vi "CRYSoundCard Editor.vi"() -> ()   [LabVIEW 2013]
uses:
  Typedef Control/CRYHardware.ctl
  Typedef Control/CRYHardware Channel Info.ctl
  <vilib>/Utility/miscctls.llb/LVBoundsTypeDef.ctl
  Typedef Control/CRYCalibration Channel ID Cluster.ctl
  CRYProject/CRYProject Editor Global.vi
  CRYMainGlobal.vi
  CRYWindow/SubVI/CRYMain Sub Window Global.vi
  Calibration/SubVI/CRYCal Global.vi
panel:
  in  "AI_HW_Changed":bool caption="啊瓷"
  in  "AO_HW_Changed":bool caption="啊瓷"
  in  "Mode":string
  out "O_Name":string[][](array[string])
  out "I_Name":string[][](array[string])
  in  "DC_Table":string[][](table)
  in  "DC_Enable":bool caption="使能"
  out "EndFlag":bool
  in  "AddStep":bool caption="Save As"
  in  "I_Cal Channel ID":T1
  in  "O_Cal Channel ID":T1
  in  "Curve Change":enum16{"Curves", "Values", "Results", "WFM"}[](array[ring])
  in  "stop":bool
  in  "Load Test":bool
  in  "Board Tab":enum32{"Page 1", "Page 2"}(tab)
  in  "Refresh":bool caption="Open_Table"
  in  "Main Tab":enum32{"Audio", "", "Help 3", "Help"}(tab)
  in  "Audio I/O Tab":enum32{"Output", "Input"}(tab)
  in  "AO_Launch":bool caption="Open_Table"
  in  "AO_Select Channel1":u16(ring) caption="选择通道" items=["左边", "右边"]
  in  "AO_Audio Driver":enum32{"Radio Selection 1", "Radio Selection 2"}(radio) caption="声卡驱动"
  out "AO_%FSD":dbl=100.0 caption="%FSD"
  in  "AO_Rename":bool caption="Open_Table"
  in  "AO_Delete":bool caption="Open_Table"
  in  "AO_Vp":dbl=0.01 caption="峰值电压（Vp）" min=0.01 format="%#.3p"
  in  "AO_Bit Depth":u16(ring) caption="比特数" items=["8 bit"=8, "16 bit"=16, "24 bit"=24, "32 bit"=32]
  in  "AO_Alias freq":u32 caption="分析频率上限" max=22050 format="%#_6f"
  in  "AO_Sampling Rate":u32(ring) caption="采样率" items=["8000 Hz"=8000, "11025 Hz"=11025, "16000 Hz"=16000, "22050 Hz"=22050, "32000 Hz"=32000, "44100 Hz"=44100, "48000 Hz"=48000, "88200 Hz"=88200, "96000 Hz"=96000, "176400 Hz"=176400, "192000 Hz"=192000, "200000 Hz"=200000, "User"=0]
  in  "AO_Select SMode":enum32{"Analog", "Digital"}(radio) caption="AO_Select Channel2"
  in  "AO_Sampling User":u32=1 caption="(Hz)" min=8000 max=200000
  in  "AO_Device Name":u16(ring) caption="设备名称" items=["扬声器 (High Definition Audio 设备)", "数字音频(S/PDIF) (High Definition A", "扬声器 (QUARTET Audio Driver)", "SPDIF 接口 (QUARTET Audio Driver)"]
  out "Advance Out Rect":bool
  in  "AO_Add":bool caption="Open_Table"
  in  "AO_SoundCard Channel":u16(ring) caption="声卡通道" items=["Output 1", "Output 2", "Output 3", "Output 4"]
  in  "AI_Audio Driver":enum32{"Radio Selection 1", "Radio Selection 2"}(radio) caption="声卡驱动"
  out "Advance In Rect":bool
  in  "AI_Vp":dbl=0.01 caption="峰值电压（Vp）" min=0.01 format="%#.3p"
  in  "AI_Bit Depth":u16(ring) caption="比特数" items=["8 bit"=8, "16 bit"=16, "24 bit"=24, "32 bit"=32]
  in  "AI_Alias freq":u32 caption="分析频率上限" max=22050 format="%#_6f"
  in  "AI_Sampling Rate":u32(ring) caption="采样率" items=["8000 Hz"=8000, "11025 Hz"=11025, "16000 Hz"=16000, "22050 Hz"=22050, "32000 Hz"=32000, "44100 Hz"=44100, "48000 Hz"=48000, "88200 Hz"=88200, "96000 Hz"=96000, "176400 Hz"=176400, "192000 Hz"=192000, "200000 Hz"=200000, "User"=0]
  in  "AI_Select SMode":enum32{"Analog", "Digital"}(radio) caption="AI_Select Channel2"
  in  "AI_Latency":u32 caption="延迟"
  in  "AI_Device Name":u16(ring) caption="设备名称" items=["麦克风 (QUARTET Audio Driver)", "线路 (QUARTET Audio Driver)"]
  in  "AI_Sampling User":u32 caption="(Hz)" min=8000 max=200000
  in  "AI_SoundCard Channel":u16(ring) caption="声卡通道" items=["Input 1", "Input 2", "Input 3", "Input 4"]
  in  "AI_Add":bool caption="Open_Table"
  in  "AI_Delete":bool caption="Open_Table"
  in  "AI_Rename":bool caption="Open_Table"
  out "AI_%FSD":dbl=100.0 caption="%FSD"
  in  "AI_Select Channel1":u16(ring) caption="选择通道" items=["左边", "右边"]
  in  "AI_Launch":bool caption="Open_Table"
  in  "Advanced View":bool
  in  "Calibration Seq":u16(ring) caption="校准序列" items=["CRY6181 Calibration"]
  in  "Calibrartion":bool caption="Open_Table"
  in  "D_Select Channel":enum32{"Radio Selection 1", "Radio Selection 2"}(radio) caption="选择通道"
  in  "D_Port No.":u32(ring) caption="端口编号"
  in  "D_PortWidth":u32 caption="端口宽度"
  in  "D_No.of Ports":u8=1 caption="端口数量" min=1
  in  "D_Device ID":u32 caption="设备编号" format="%_1f"
  in  "D_Enable":bool caption="启用"
  in  "I_Data bits":u8 caption="数据位" min=5 max=8
  in  "I_Baud":u16 caption="波特率"
  in  "I_COM Port":u8=1 caption="串行通讯端口" min=1
  in  "I_Flow control":u8(ring) caption="流控制" items=["Xon/Xoff", "Hardware", "None"]
  in  "I_Stop bits":u8(ring) caption="停止位" items=["1", "1.5", "2"]
  in  "I_Parity":u8(ring) caption="奇偶性" items=["None", "Odd", "Even", "Mark", "Space"]
  in  "I_No":u32(ring) caption="接口号"
  in  "I_Type":u8(ring) caption="类型" items=["IEEE-488", "RS-232", "Footswitch", "Buzzer"]
  in  "I_How many":u32 caption="接口数量"
  in  "I_Dev ID IEEE":u8 caption="设备标识 IEEE"
  in  "Help":string
  in  "Open_Table":bool
  in  "SaveSoundCard":bool caption="Apply"
  in  "Cancel":bool caption="Apply"
  in  "Load...":bool caption="Apply"
  in  "Revert":bool caption="Apply"
  out "Channel Info":T2={"ID"=0, "Name"="", "Digital"=FALSE, "Input"=FALSE, "Device Name"="", "Hardware Ch ID"=0, "Vmax (V)"=0.0, "Latency (samples)"=0.0, "Sampling Rate (Hz)"=0, "Bit Depth"=0, "Anti-aliasing Factor (%fs)"=0.475, "DAQmx Channel"="", "term config"=-1, "Coupling"=10050, "IEPE en"=FALSE, "ASIOChannel Name"="", "Audio Driver"=0, "ASIOChannel Index"=0} {"Coupling" items=["Default"=-1, "RSE"=10083, "NRSE"=10078, "Differential"=10106, "Pseudodifferential"=12529]; "term config" items=["Default"=-1, "RSE"=10083, "NRSE"=10078, "Differential"=10106, "Pseudodifferential"=12529]; "Anti-aliasing Factor (%fs)" format="%.2f"}
  out "O_Channel Info":T2[](array[typedef]) {"Coupling" items=["Default"=-1, "RSE"=10083, "NRSE"=10078, "Differential"=10106, "Pseudodifferential"=12529]; "term config" items=["Default"=-1, "RSE"=10083, "NRSE"=10078, "Differential"=10106, "Pseudodifferential"=12529]; "Anti-aliasing Factor (%fs)" format="%.2f"}
  in  "I_Channel Info":T2[](array[typedef]) {"Coupling" items=["Default"=-1, "RSE"=10083, "NRSE"=10078, "Differential"=10106, "Pseudodifferential"=12529]; "term config" items=["Default"=-1, "RSE"=10083, "NRSE"=10078, "Differential"=10106, "Pseudodifferential"=12529]; "Anti-aliasing Factor (%fs)" format="%.2f"}
  out "I_Device Info":T3(array[cluster])
  out "O_Device Info":T3(array[cluster])
  out "Proper VI No":i32
  out "VIMiniumBound":T4
  in  "SoundCard":T5={"Name"="", "Analog I/O"=0, "Digital I/O"=0, "Channels"=2, "Dig Dev ID"=1, "N ports"=3, "Interface"=0, "Dig I/O Ports"=[{"port #"=1, "width"=8, "direction"=0}, {"port #"=2, "width"=8, "direction"=0}, {"port #"=3, "width"=8, "direction"=0}], "Interf settings"=[], "N interfs"=3, "udev SNs"=[], "udev enable"=FALSE, "Channel Array"=[], "Cal sequence"="", "SelectedIn"=0, "SelectedOut"=0, "SelectedTab"=0, "State"=FALSE, "Help"="", "Advanced"=FALSE, "In Audio Driver"=0, "Out Audio Driver"=0} caption="Hardware" {"Channel Array"."Coupling" items=["Default"=-1, "RSE"=10083, "NRSE"=10078, "Differential"=10106, "Pseudodifferential"=12529]; "Channel Array"."term config" items=["Default"=-1, "RSE"=10083, "NRSE"=10078, "Differential"=10106, "Pseudodifferential"=12529]; "Channel Array"."Anti-aliasing Factor (%fs)" format="%.2f"}
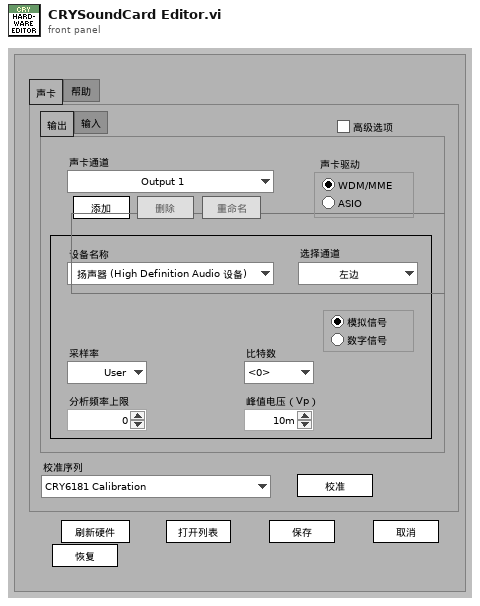
[diagram p1: front panel]
types:
  T1 = typedef "CRYCalibration Channel ID Cluster.ctl" = cluster{"Edit Name":string, "Edit ID":i8}[]
  T2 = typedef "CRYHardware Channel Info.ctl" = cluster{"ID":i32, "Name":string, "Digital":bool, "Input":bool, "Device Name":string, "Hardware Ch ID":u8, "Vmax (V)":dbl, "Latency (samples)":dbl, "Sampling Rate (Hz)":u32, "Bit Depth":u32, "Anti-aliasing Factor (%fs)":sgl, "DAQmx Channel":tag, "term config":i32, "Coupling":i32, "IEPE en":bool, "ASIOChannel Name":string, "Audio Driver":u16, "ASIOChannel Index":u8}
  T3 = cluster{"Name":string, "MinFreq":dbl, "MaxFreq":dbl, "Channel":i32[], "Depths":i32[], "Channel Names":string[], "SampleRates Array":dbl[], "Driver Type":string}[]
  T4 = typedef "LVBoundsTypeDef.ctl" = cluster{"Width":u32, "Height":u32}
  T5 = typedef "CRYHardware.ctl" = cluster{"Name":string, "Analog I/O":u16, "Digital I/O":u16, "Channels":u8, "Dig Dev ID":u8, "N ports":u8, "Interface":u32, "Dig I/O Ports":cluster{"port #":i16, "width":i16, "direction":i32}[], "Interf settings":cluster{"Type":u16, "COM Port":u8, "Baud rate":u32, "Data bits":u32, "Parity":u16, "Stop bits":u16, "Flow control":u16, "Dev ID IEEE":u8}[], "N interfs":i32, "udev SNs":i16[], "udev enable":bool, "Channel Array":T2[], "Cal sequence":string, "SelectedIn":u16, "SelectedOut":u16, "SelectedTab":u16, "State":bool, "Help":string, "Advanced":bool, "In Audio Driver":u16, "Out Audio Driver":u16}
  T6 = typedef "CRYStep.ctl" = cluster{"No.VI":i32, "Category":string, "StepName":string, "Seq setup flattened":string, "Comment":string, "Steps config.":bool[], "Jump config":i32[], "Start":dbl, "Increment":dbl, "Name":string, "Unit":string, "Y data":u16, "Y prefix":string, "Y dB ref":dbl, "Y unit":string, "Repeat State Array":cluster{"Start":dbl, "Increment":dbl, "Count":i32, "Num":i32}[]}
  T7 = enum8{"Enabled", "Disabled", "Disabled and Grayed Out"}
  T8 = enum16{"OK", "Yes", "YesNo", "YesNoCancel", "ReplaceAppend"}
  T9 = cluster{"port #":i16, "width":i16, "direction":i32}[]
  T10 = cluster{"port #":i16, "width":i16, "direction":i32}
  T11 = cluster{"Type":u16, "COM Port":u8, "Baud rate":u32, "Data bits":u32, "Parity":u16, "Stop bits":u16, "Flow control":u16, "Dev ID IEEE":u8}
  T12 = cluster{"Name":string, "MinFreq":dbl, "MaxFreq":dbl, "Channel":i32[], "Depths":i32[], "Channel Names":string[], "SampleRates Array":dbl[], "Driver Type":string}
  T13 = typedef "LVStringsAndValuesArrayTypeDef_U32.ctl" = cluster{"String":string, "Value":u32}[]
  T14 = cluster{"Type":u16, "COM Port":u8, "Baud rate":u32, "Data bits":u32, "Parity":u16, "Stop bits":u16, "Flow control":u16, "Dev ID IEEE":u8}[]
  T15 = cluster{bool, "AO_Add":bool, "AO_Delete":bool, "AO_Rename":bool, "AI_Add":bool, "AI_Delete":bool, "AI_Rename":bool, "Open_Table":bool, "Calibrartion":bool, "SaveSoundCard":bool, "Cancel":bool}
  T16 = typedef "CRYData Cluster Array.ctl" = T17[]
  T17 = typedef "CRYData Cluster.ctl" = cluster{"Name":string, "Curve":cluster{"x":dbl, "y":dbl, "z":dbl}[], "X data":u16, "Y data":u16, "Z data":u16, "X axis":u16, "Y axis":u16, "Z axis":u16, "X unit":string, "Y unit":string, "Z unit":string, "X dB ref":dbl, "Y dB ref":dbl, "Z dB ref":dbl, "single val":bool, "protected":bool, "display X":bool, "display Y":bool, "display Z":bool, "Test Info":string, "Step No.":i32, "Plot Settings":cluster{"Color":u32, "Interpolation":u8, "Point Style":u8, "Line Style":u8, "Point Color":u32, "Line Width":u8, "Bar Plot Style":u8, "Fill To":i16}, "AutoProtect":bool}
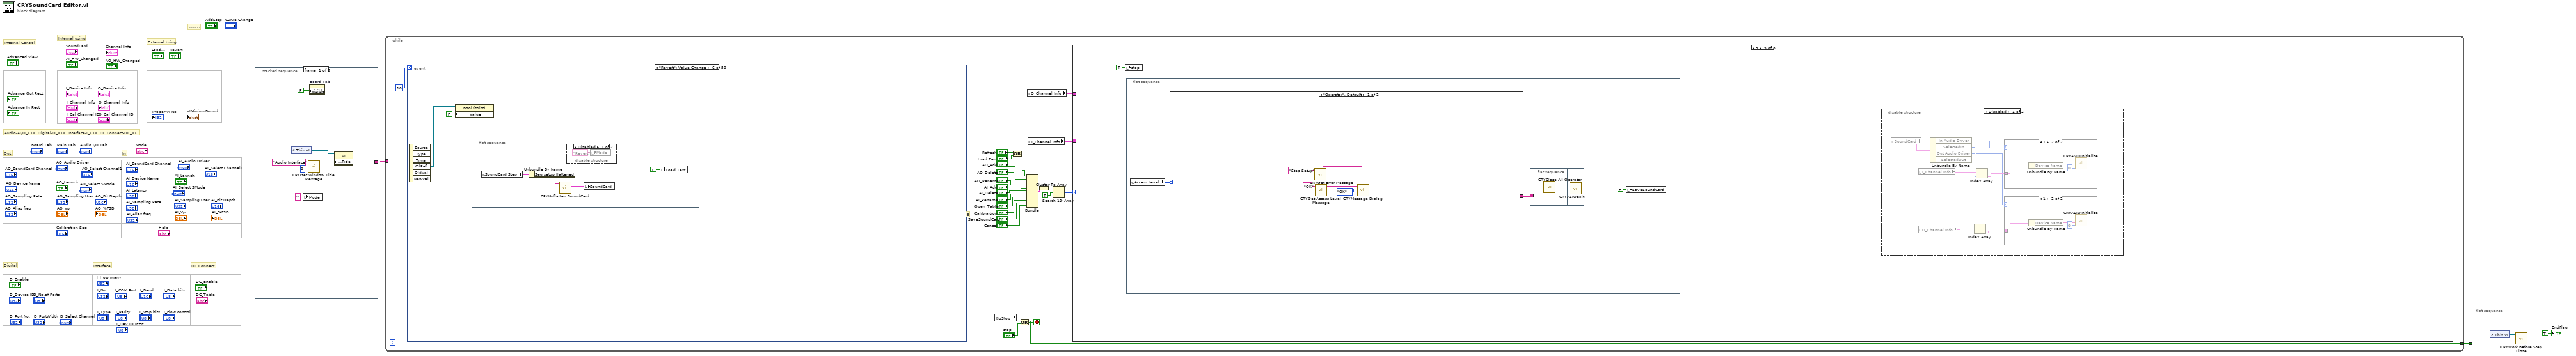
[diagram p0: block diagram]
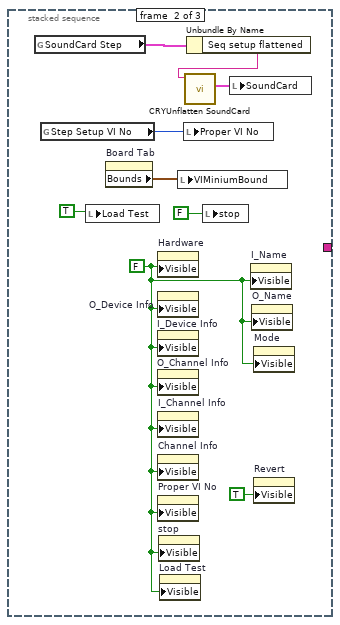
[diagram p2: hidden frame]
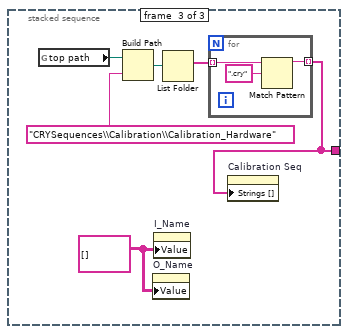
[diagram p3: hidden frame]
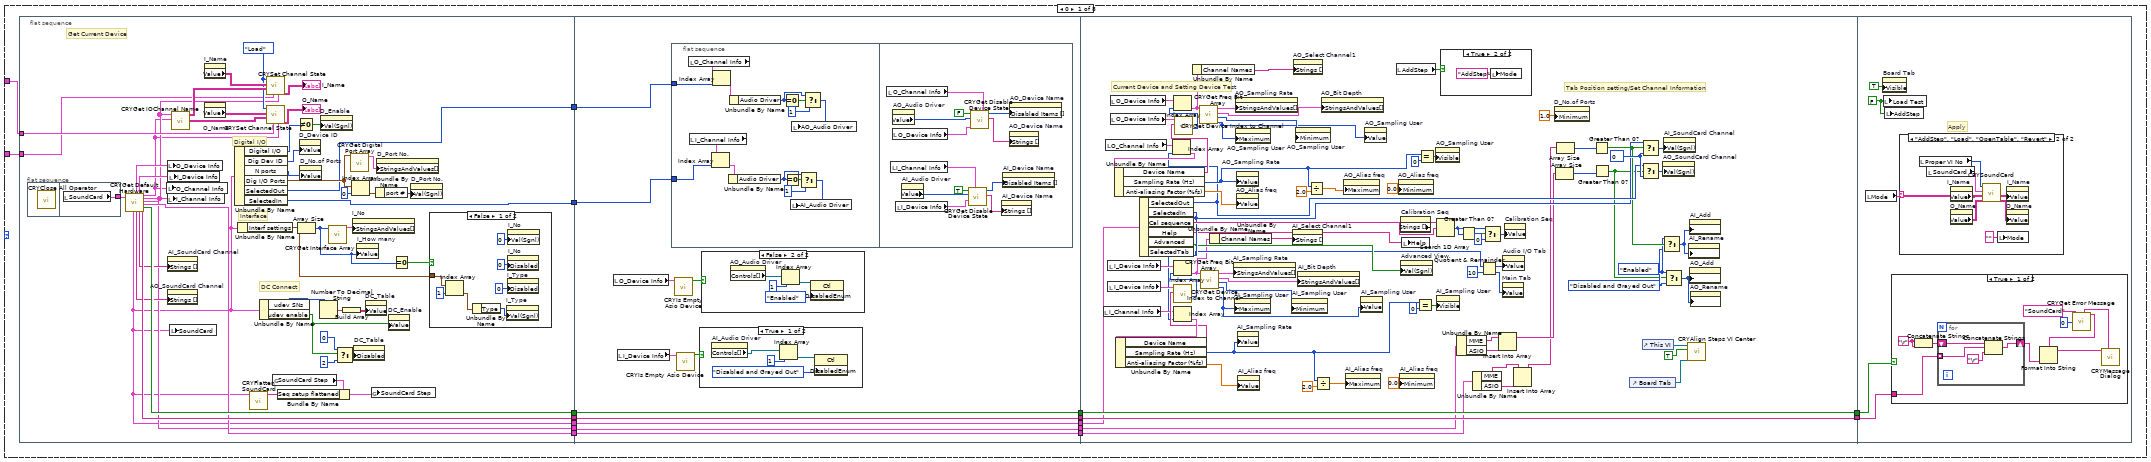
[diagram p4: hidden frame]
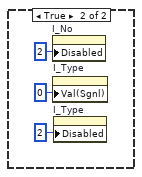
[diagram p5: hidden frame]
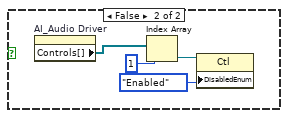
[diagram p6: hidden frame]
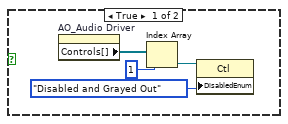
[diagram p7: hidden frame]
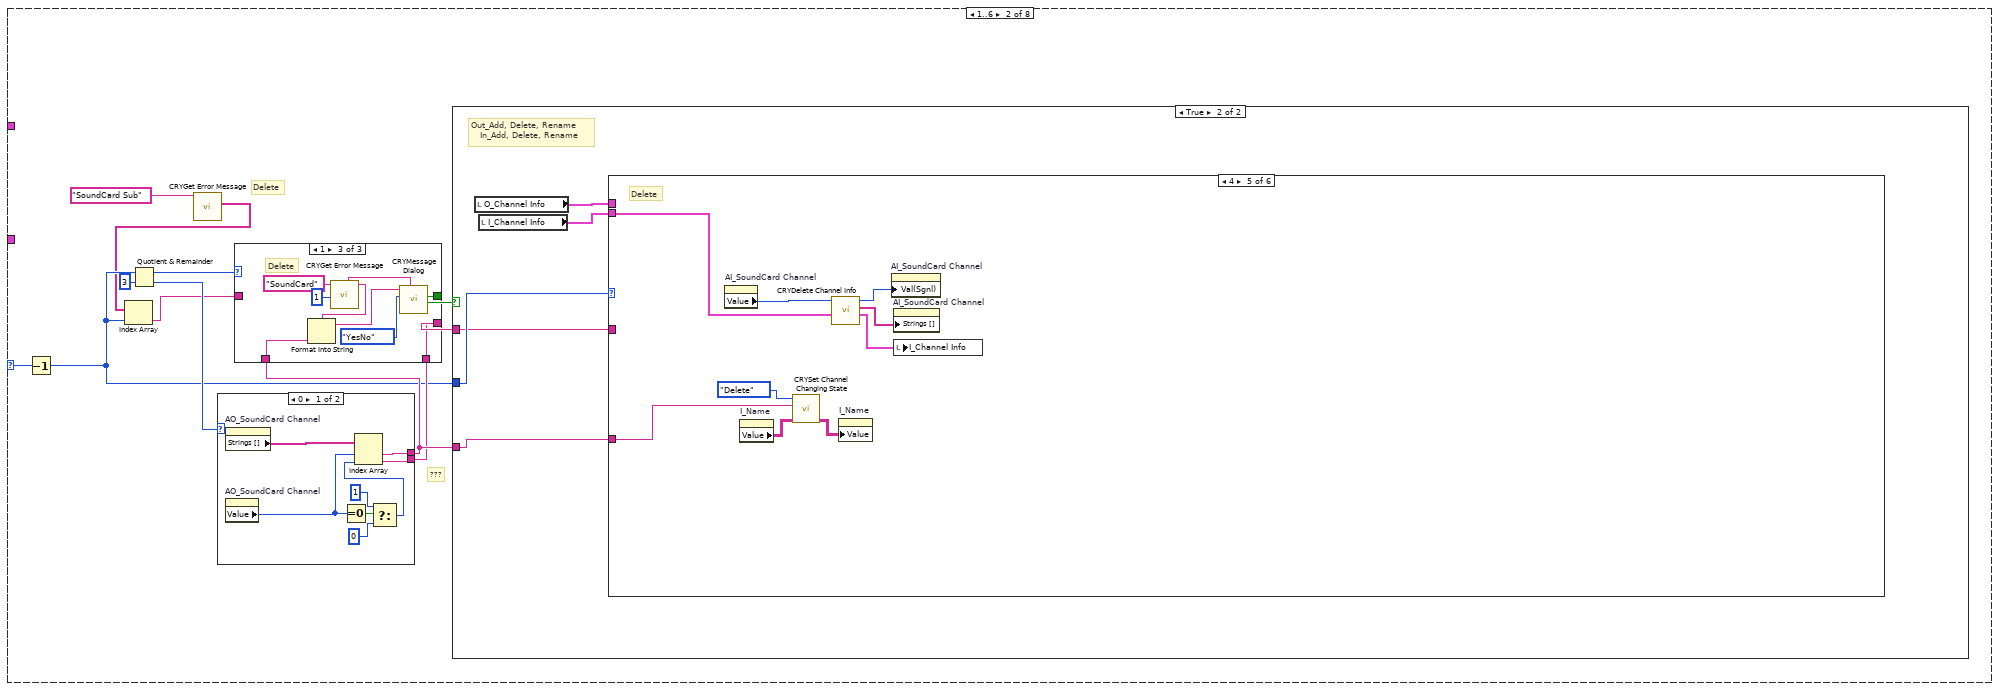
[diagram p11: hidden frame]
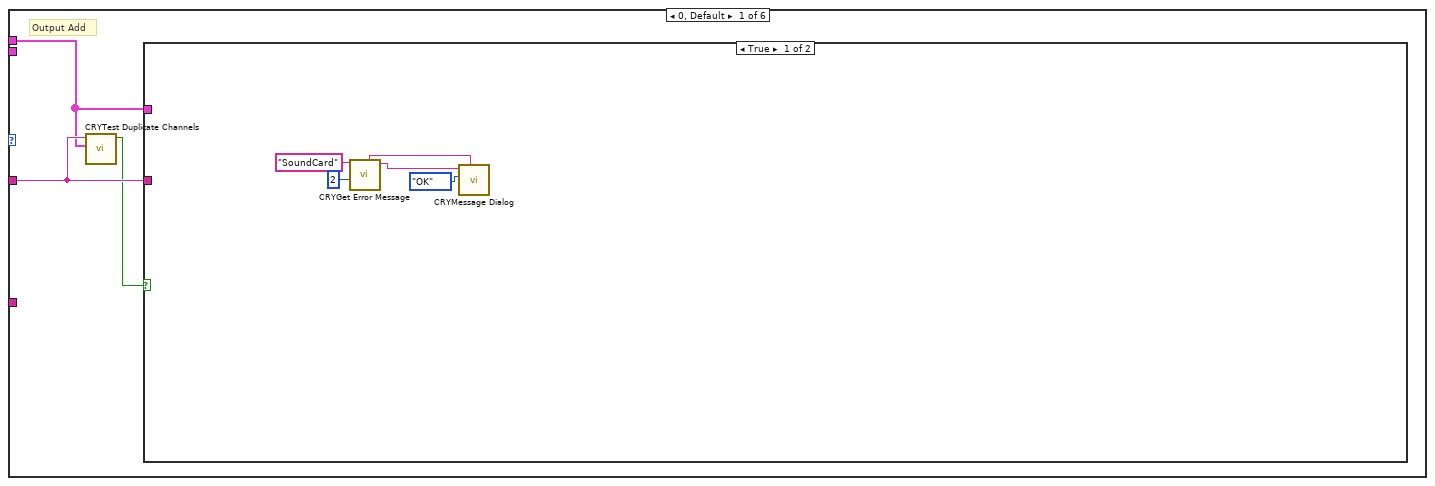
[diagram p13: hidden frame]
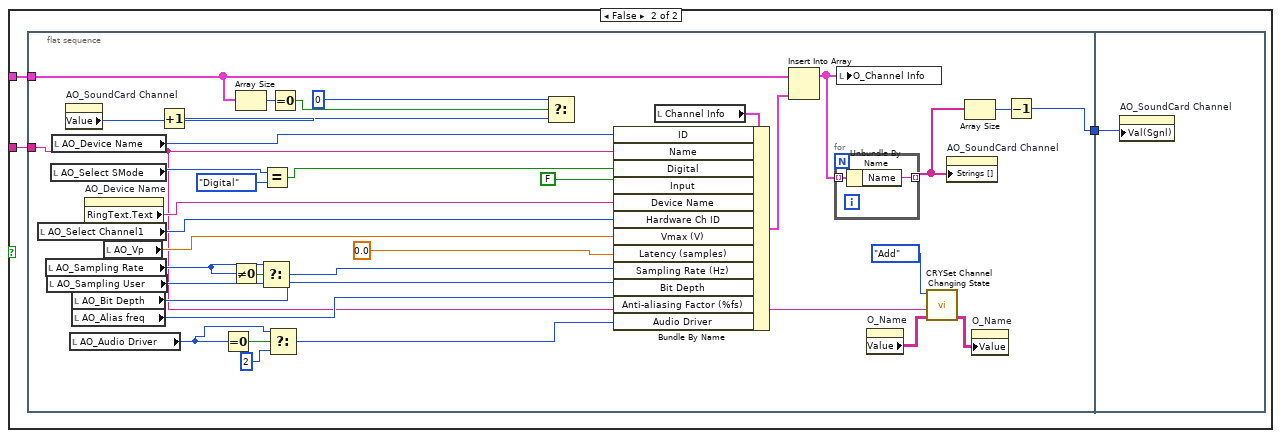
[diagram p14: hidden frame]
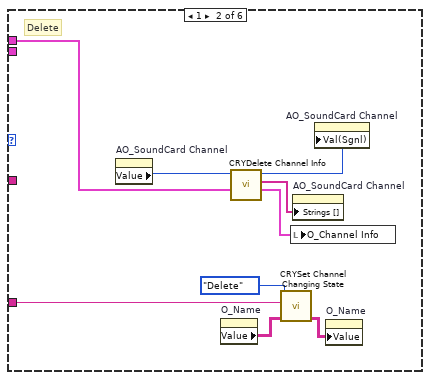
[diagram p15: hidden frame]
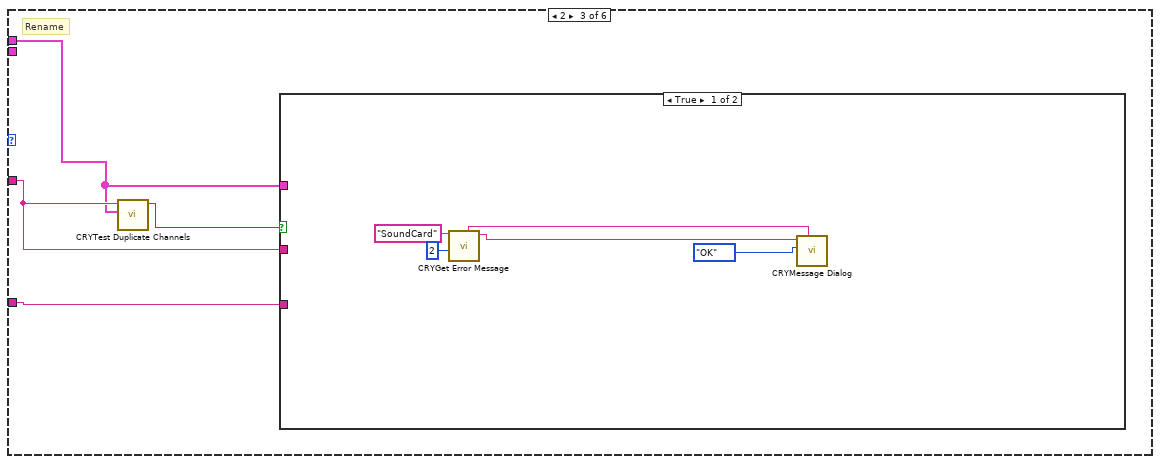
[diagram p16: hidden frame]
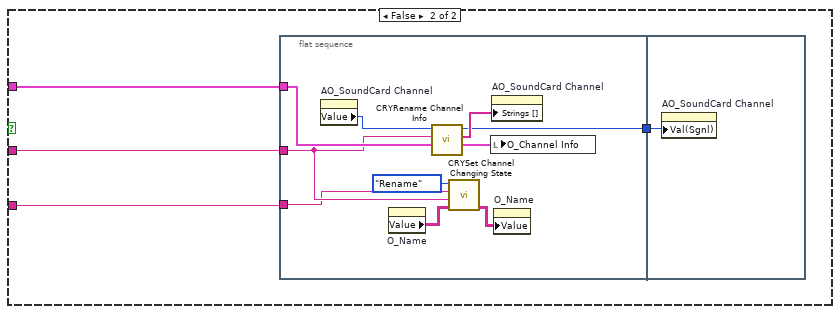
[diagram p17: hidden frame]
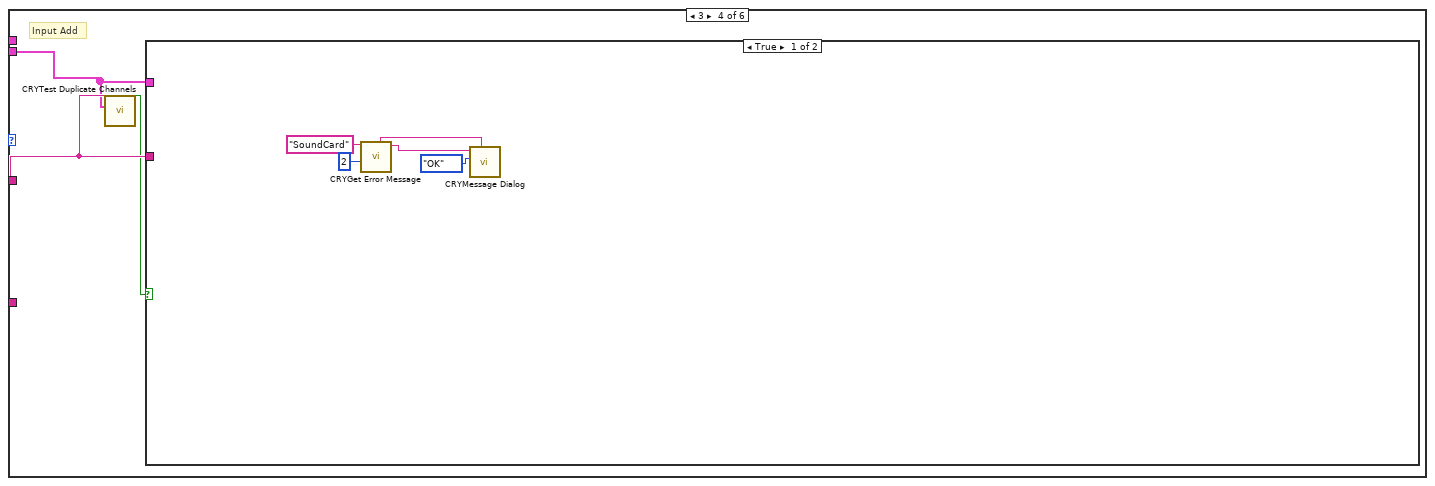
[diagram p18: hidden frame]
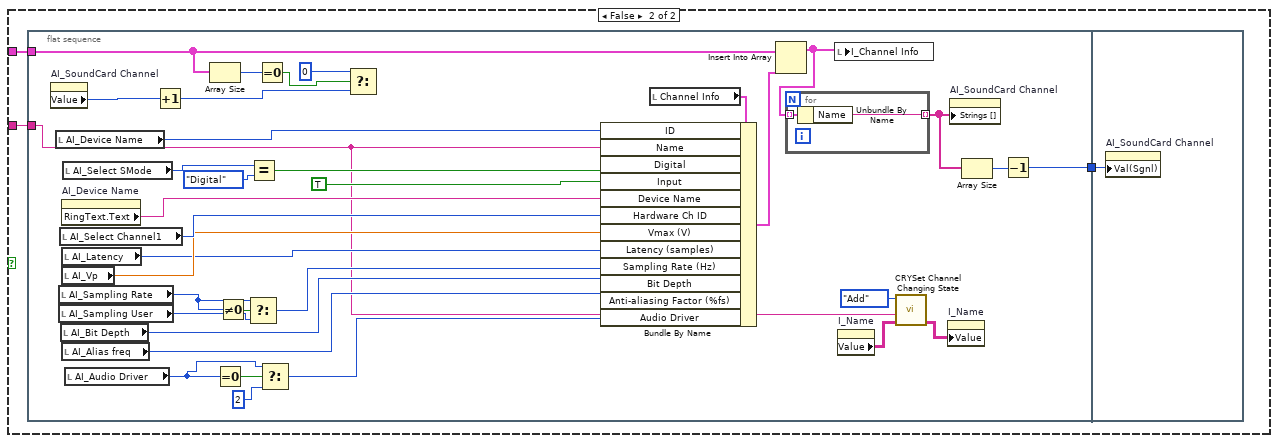
[diagram p19: hidden frame]
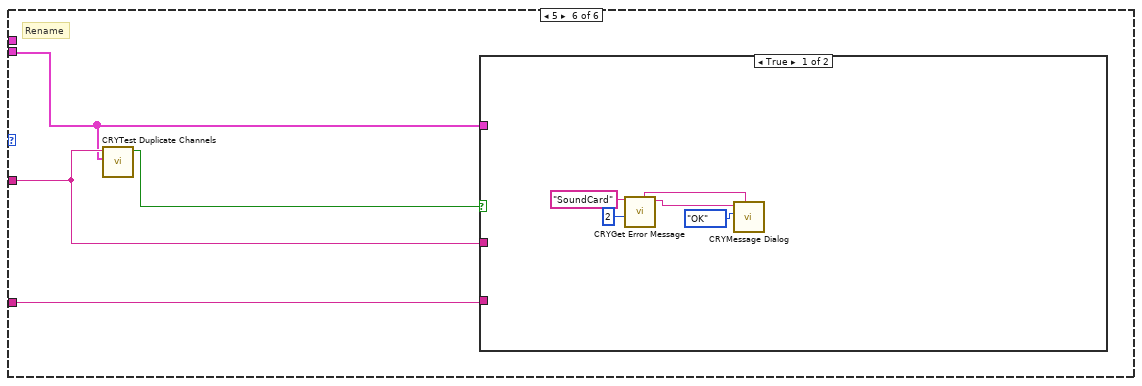
[diagram p20: hidden frame]
diagram:
  # "Internal using"
  # "??????"
  # "Internal Control"
  # "External Using"
  # "DC Connect"
  # "Interface"
  # "Digital"
  # "Out"
  # "In"
  # "Audio-AI/O_XXX, Digital-D_XXX, Interface-I_XXX, DC Connect-DC_XX"
  n1 = stacked-sequence {
    tunnel: [_ _ w19] -> w2
    frame #0 {
      n2 = control-ref of="This VI"() -> (w3:refnum<vi>)
      n3 = local write "Mode"("" ("Mode")) -> ()
      n4 = call "CRYGet Window Title Message.vi"("No"=0, "Kind"="Audio Interface") -> ("Multibyte String"=w4:string)  [unwired: 4 in, 5 out]
      n5 = property on="Board Tab" class="TabCtl (strict)"("Visible"=FALSE) -> ()  [unwired: 2 in, 2 out]
      n6 = property class="VI"(reference=w3, "Front Panel.Title"=w4) -> ()  [unwired: 1 in, 2 out]
    }
    frame #1 {
      w10 = FALSE ("Visible")
      n7 = global read "CRYProject Editor Global.vi" "SoundCard Step"() -> (w17:T6)
      n8 = global read "CRYProject Editor Global.vi" "Step Setup VI No"() -> (w14:i32)
      n9 = local write "Load Test"(TRUE ("Load Test")) -> ()
      n10 = property on="Board Tab" class="TabCtl (strict)"() -> ("Bounds"=w12:T4)  [unwired: 2 in, 2 out]
      n11 = property on="Hardware" class="Clust (strict)"("Visible"=w10) -> ()  [unwired: 2 in, 2 out]
      n12 = property on="O_Device Info" class="Arr (strict)"("Visible"=w10) -> ()  [unwired: 2 in, 2 out]
      n13 = property on="I_Device Info" class="Arr (strict)"("Visible"=w10) -> ()  [unwired: 2 in, 2 out]
      n14 = property on="O_Channel Info" class="Arr (strict)"("Visible"=w10) -> ()  [unwired: 2 in, 2 out]
      n15 = property on="I_Channel Info" class="Arr (strict)"("Visible"=w10) -> ()  [unwired: 2 in, 2 out]
      n16 = property on="Channel Info" class="Clust (strict)"("Visible"=w10) -> ()  [unwired: 2 in, 2 out]
      n17 = property on="Proper VI No" class="DigNum (strict)"("Visible"=w10) -> ()  [unwired: 2 in, 2 out]
      n18 = property on="stop" class="Bool (strict)"("Visible"=w10) -> ()  [unwired: 2 in, 2 out]
      n19 = property on="Load Test" class="Bool (strict)"("Visible"=w10) -> ()  [unwired: 2 in, 2 out]
      n20 = local write "VIMiniumBound"(w12) -> ()
      n21 = local write "Proper VI No"(w14) -> ()
      n22 = Unbundle By Name(w17) -> ("Seq setup flattened"=w16:string)
      n23 = call "CRYUnflatten SoundCard.vi"("Flatten SoundCard"=w16) -> ("SoundCard"=w13:T5)  [unwired: 10 out]
      n24 = local write "stop"(FALSE ("Open Table")) -> ()
      n25 = local write "SoundCard"(w13) -> ()
      n26 = property on="I_Name" class="Arr (strict)"("Visible"=w10) -> ()  [unwired: 2 in, 2 out]
      n27 = property on="O_Name" class="Arr (strict)"("Visible"=w10) -> ()  [unwired: 2 in, 2 out]
      n28 = property on="Mode" class="Str"("Visible"=w10) -> ()  [unwired: 2 in, 2 out]
      n29 = property on="Revert" class="Bool (strict)"("Visible"=TRUE) -> ()  [unwired: 2 in, 2 out]
    }
    frame #2 {
      w18 = string[][] [] ("I_Name")
      n30 = global read "CRYMainGlobal.vi" "top path"() -> (w21:path)
      n31 = Build Path(base path=w21, name or relative path="CRYSequences\\Calibration\\Calibration_Hardware") -> (appended path=w23:path)
      n32 = property on="O_Name" class="Arr (strict)"("Value"=w18) -> ()  [unwired: 2 in, 2 out]
      n33 = property on="I_Name" class="Arr (strict)"("Value"=w18) -> ()  [unwired: 2 in, 2 out]
      n34 = List Folder(path=w23) -> (filenames=w22:string[])  [unwired: 1 in, 5 out]
      n35 = for {
        tunnel: w22 -> [w25] mode=indexing
        tunnel: [w24] -> w19 mode=indexing
        n36 = Match Pattern(string=w25, regular expression=".cry") -> (before substring=w24:string)  [unwired: 4 out]
      }
      n37 = property on="Calibration Seq" class="Ring (strict)"("Strings []"=w19) -> ()  [unwired: 2 in, 2 out]
    }
  }
  n38 = while {
    tunnel: w2 -> [_]
    tunnel: [w29] -> w1
    stop <- w29 stop-if-true
    # "8"
    n39 = event shown="[5] \"Revert\": Value Change" {
      selector: _ -> [_ _ _ _ _ _ _ _ _ _ _ _ _ _ _ _ _ _ _ _ _ _ _ _ _ _ _ _ _ _ _ _ _ _ _ _ _ _ _ _ _ _ _ _ _ _ _ _ _ _]
      dyn-events: _ -> [_ _ _ _ _ _ _ _ _ _ _ _ _ _ _ _ _ _ _ _ _ _ _ _ _ _ _ _ _ _ _ _ _ _ _ _ _ _ _ _ _ _ _ _ _ _ _ _ _ _]
      timeout: 10 -> [_ _ _ _ _ _ _ _ _ _ _ _ _ _ _ _ _ _ _ _ _ _ _ _ _ _ _ _ _ _ _ _ _ _ _ _ _ _ _ _ _ _ _ _ _ _ _ _ _ _]
      event Timeout {
        n40 = event-data() -> ()  [unwired: 3 out]
      }
      event Pane Size {
        n41 = event-data() -> ()  [unwired: 7 out]
        n42 = control-ref of="Board Tab"() -> (w808:refnum<vi>)
        n43 = control-ref of="This VI"() -> (w806:refnum<vi>)
        n44 = call "CRYAlign Steps VI Center.vi"("Tab2"=w808, "Input/Output"=TRUE ("Preview"), "VIRef"=w806) -> ()  [unwired: 1 in, 8 out]
      }
      event "Load...": Value Change {
        n45 = event-data() -> ("CtlRef"=w809:refnum<vi>)  [unwired: 6 out]
        n46 = local read "Load Test"() -> (w811:bool)
        n47 = property class="Bool (strict)"(reference=w809, "Value"=FALSE) -> ()  [unwired: 1 in, 2 out]
        n48 = case shown="False" w811 {
          frame True {
          }
          frame False {
            n49 = global read "CRYMainGlobal.vi" "Steps path"() -> (w816:path)
            n50 = Build Path(base path=w816, name or relative path="CRYSoundCard") -> (appended path=w815:path)
            n51 = call "CRYStep Read.vi"("Category Name"="SoundCard" ("Step File Name"), "Step File Path"=w815) -> ("status"=w814:bool, "selected path"=w812:path, "Flatten Step"=w813:string)  [unwired: 2 in, 3 out]
            n52 = case shown="True" w814 {
              tunnel: w813 -> [_ w819]
              tunnel: w812 -> [_ w820]
              frame False {
              }
              frame True {
                n53 = call "CRYUnflatten SoundCard.vi"("Flatten SoundCard"=w819) -> ("Error?"=w821:bool, "SoundCard"=w822:T5)  [unwired: 9 out]
                n54 = case shown="False" w821 {
                  tunnel: w822 -> [w825 _]
                  tunnel: w820 -> [w824 _]
                  tunnel: w819 -> [w823 _]
                  frame False {
                    n55 = flat-sequence {
                      tunnel: w824 -> [w828]
                      tunnel: w825 -> [w827]
                      tunnel: w823 -> [w826]
                      frame #0 {
                        # "Applay"
                        n56 = Strip Path(path=w828) -> (name=w838:string)  [unwired: 1 out]
                        n57 = Reverse String(1:w838) -> (0:w837:string)
                        n58 = local write "Mode"("Load" ("Mode")) -> ()
                        n59 = Match Pattern(string=w837, regular expression="[.]") -> (after substring=w836:string)  [unwired: 4 out]
                        n60 = global read "CRYProject Editor Global.vi" "SoundCard Step"() -> (w830:T6)
                        n61 = Bundle By Name(cluster=w830, "Seq setup flattened"=w826) -> (w829:T6)
                        n62 = local read "Proper VI No"() -> (w831:i32)
                        n63 = Reverse String(1:w836) -> (0:w835:string)
                        n64 = global write "CRYProject Editor Global.vi" "G_Audi Interface Step path"(w828) -> ()
                        n65 = local write "SoundCard"(w827) -> ()
                        n66 = call "CRYPreUpdate Sequence.vi"("EventName"="Load", "StepName Arg3"=w835, "Proper VI No"=w831, "Project View Step Name Identifier Arg1"="", "Step flattened Arg2"=w826, "AllChangeFlg"=TRUE ("Name/Identifier")) -> ()  [unwired: 10 in]
                        n67 = global write "CRYProject Editor Global.vi" "SoundCard Step"(w829) -> ()
                      }
                      frame #1 {
                        n68 = local write "Load Test"(TRUE ("Load Test")) -> ()
                      }
                    }
                  }
                  frame True {
                  }
                }
              }
            }
          }
        }
      }
      event "AO_Launch": Value Change {
        n69 = event-data() -> ("CtlRef"=w843:refnum<vi>)  [unwired: 6 out]
        n70 = flat-sequence {
          tunnel: w843 -> [w844]
          tunnel: [w844] -> w842
          tunnel: w842 -> [w845]
          frame #0 {
            n71 = call "CRYClose All Operator.vi"() -> ()  [unwired: 12 in]
          }
          frame #1 {
            n72 = property class="Bool (strict)"(reference=w845, "Value"=FALSE) -> ()  [unwired: 1 in, 2 out]
          }
          frame #2 {
            n73 = property on="AO_Sampling Rate" class="Ring (strict)"() -> ("RingText.Text"=w848:string)  [unwired: 2 in, 2 out]
            n74 = property on="AO_Device Name" class="Ring (strict)"() -> ("RingText.Text"=w847:string)  [unwired: 2 in, 2 out]
            n75 = Decimal String To Number(string=w848, default (0L)=44100 ("default (0 I32)")) -> (number=w850:i32)  [unwired: 1 in, 1 out]
            n76 = call "CRYASIOLaunchControlPanel.vi"("Fs"=w850, "Driver Name"=w847) -> ()  [unwired: 9 in, 1 out]
          }
        }
      }
      event "AI_Launch": Value Change {
        n77 = event-data() -> ("CtlRef"=w852:refnum<vi>)  [unwired: 6 out]
        n78 = flat-sequence {
          tunnel: w852 -> [w853]
          tunnel: [w853] -> w851
          tunnel: w851 -> [w855]
          frame #0 {
            n79 = call "CRYClose All Operator.vi"() -> ()  [unwired: 12 in]
          }
          frame #1 {
            n80 = property class="Bool (strict)"(reference=w855, "Value"=FALSE) -> ()  [unwired: 1 in, 2 out]
          }
          frame #2 {
            n81 = property on="AI_Sampling Rate" class="Ring (strict)"() -> ("RingText.Text"=w859:string)  [unwired: 2 in, 2 out]
            n82 = property on="AI_Device Name" class="Ring (strict)"() -> ("RingText.Text"=w858:string)  [unwired: 2 in, 2 out]
            n83 = Decimal String To Number(string=w859, default (0L)=44100 ("default (0 I32)")) -> (number=w857:i32)  [unwired: 1 in, 1 out]
            n84 = call "CRYASIOLaunchControlPanel.vi"("Fs"=w857, "Driver Name"=w858) -> ()  [unwired: 9 in, 1 out]
          }
        }
      }
      event "Revert": Value Change {
        n85 = event-data() -> ("CtlRef"=w861:refnum<vi>)  [unwired: 6 out]
        n86 = property class="Bool (strict)"(reference=w861, "Value"=FALSE) -> ()  [unwired: 1 in, 2 out]
        n87 = flat-sequence {
          frame #0 {
            n88 = global read "CRYProject Editor Global.vi" "SoundCard Step"() -> (w864:T6)
            n89 = Unbundle By Name(w864) -> ("Seq setup flattened"=w863:string)
            n90 = call "CRYUnflatten SoundCard.vi"("Flatten SoundCard"=w863) -> ("SoundCard"=w862:T5)  [unwired: 10 out]
            n91 = disable-structure shown="Disabled" {
              frame Disabled {
                n92 = local write "Mode"("Revert" ("Mode")) -> ()
              }
              frame Enabled {
              }
            }
            n93 = local write "SoundCard"(w862) -> ()
          }
          frame #1 {
            n94 = local write "Load Test"(TRUE ("Load Test")) -> ()
          }
        }
      }
      event Panel Close {
        n95 = event-data() -> ()  [unwired: 5 out]
        n96 = local write "Cancel"(TRUE ("Cancel")) -> ()
        n97 = control-ref of="This VI"() -> (w868:refnum<vi>)
        n98 = call "CRYWork Before Step Close.vi"("StepVI Ref"=w868) -> ()  [unwired: 11 in]
      }
      event "Main Tab": Value Change {
        n99 = event-data() -> ("NewVal"=w872:enum32{"Audio", "", "Help 3", "Help"})  [unwired: 6 out]
        n100 = property on="Audio I/O Tab" class="TabCtl (strict)"() -> ("Value"=w871:enum32{"Output", "Input"})  [unwired: 2 in, 2 out]
        n101 = Multiply(x=w872, y=u16 10) -> (x*y=w874:u32)
        n102 = Add(x=w874, y=w871) -> (x+y=w873:u32)
        n103 = local read "SoundCard"() -> (w870:T5)
        n104 = Bundle By Name(cluster=w870, "SelectedTab"=w873) -> (w869:T5)
        n105 = local write "SoundCard"(w869) -> ()
      }
      event "Audio I/O Tab": Value Change {
        n106 = event-data() -> ("NewVal"=w880:enum32{"Output", "Input"})  [unwired: 6 out]
        n107 = property on="Main Tab" class="TabCtl (strict)"() -> ("Value"=w878:enum32{"Audio", "", "Help 3", "Help"})  [unwired: 2 in, 2 out]
        n108 = Multiply(x=w878, y=u16 10) -> (x*y=w881:u32)
        n109 = Add(x=w881, y=w880) -> (x+y=w879:u32)
        n110 = local read "SoundCard"() -> (w877:T5)
        n111 = Bundle By Name(cluster=w877, "SelectedTab"=w879) -> (w876:T5)
        n112 = local write "SoundCard"(w876) -> ()
      }
      event "AO_SoundCard Channel": Value Change {
        n113 = event-data() -> ("NewVal"=w902:u16)  [unwired: 6 out]
        n114 = local read "O_Channel Info"() -> (w912:T2[])
        n115 = local read "SoundCard"() -> (w899:T5)
        n116 = Bundle By Name(cluster=w899, "SelectedOut"=w902) -> (w898:T5)
        n117 = Index Array(array=w912, index=w902) -> (element=w911:T2)
        n118 = flat-sequence {
          tunnel: w897 -> [w935]
          frame #0 {
            n119 = local write "AO_HW_Changed"(TRUE ("HW_Changed")) -> ()
          }
          frame #1 {
            n120 = property on="AO_Audio Driver" class="RadioBtnsControl (strict)"("Val(Sgnl)"=w935) -> ()  [unwired: 2 in, 2 out]
          }
        }
        n121 = Unbundle By Name(w911) -> ("Name"=w895:string, "Digital"=w906:bool, "Device Name"=w901:string, "Hardware Ch ID"=w908:u8, "Vmax (V)"=w909:dbl, "Sampling Rate (Hz)"=w904:u32, "Bit Depth"=w910:u32, "Anti-aliasing Factor (%fs)"=w903:sgl, "Audio Driver"=w897:u16)  [unwired: 2 out]
        n122 = local write "SoundCard"(w898) -> ()
        n123 = local write "AO_Bit Depth"(w910) -> ()
        n124 = local write "AO_Alias freq"(w903) -> ()
        n125 = local write "AO_Vp"(w909) -> ()
        n126 = local write "AO_Select Channel1"(w908) -> ()
        n127 = Select(t=enum32{"Analog", "Digital"}."Digital" ("AO_Select Channel2"), s=w906, f=enum32{"Analog", "Digital"}."Analog" ("AO_Select Channel2")) -> (s? t:f=w900:enum32{"Analog", "Digital"})
        n128 = local read "O_Channel Info"() -> (w892:T2[])
        n129 = property on="AO_Audio Driver" class="RadioBtnsControl (strict)"() -> ("Value"=w893:enum32{"Radio Selection 1", "Radio Selection 2"})  [unwired: 2 in, 2 out]
        n130 = local read "O_Device Info"() -> (w890:T3)
        n131 = property on="AO_Select SMode" class="RadioBtnsControl (strict)"("Val(Sgnl)"=w900) -> ()  [unwired: 2 in, 2 out]
        n132 = call "CRYGet Disable Device State.vi"("O_Channel Info"=w892, "O_Device Info In"=w890, "Audio Driver"=w893, "In/Out"=FALSE) -> ("All I/O_Device Info Out"=w885:T3)  [unwired: 5 in, 2 out]
        n133 = call "CRYGet Device Index to Channel.vi"("Device Name In"=w901, "Device Info In"=w885) -> ("Device Index Out"=w883:i32)  [unwired: 9 out]
        n134 = Index Array(array=w885, index=w883) -> (element=w889:T12)
        n135 = Unbundle By Name(w889) -> ("Channel Names"=w888:string[])
        n136 = Index Array(array=w888) -> (element=w887:string)  [unwired: 1 in]
        n137 = Not Equal?(x=w887, y="No") -> (x != y?=w884:bool)
        n138 = case shown="True" w884 {
          tunnel: w904 -> [_ w917]
          frame False {
          }
          frame True {
            n139 = property on="AO_Sampling Rate" class="Ring (strict)"() -> ("StringsAndValues[]"=w921:T13)  [unwired: 2 in, 2 out]
            n140 = for {
              tunnel: w921 -> [w933] mode=indexing
              shift-right: [w932] -> w916
              shift-left: u32[] [] -> [w930]
              n141 = Unbundle By Name(w933) -> ("Value"=w931:u32)
              n142 = Insert Into Array(array=w930, new element=w931) -> (w932:u32[])  [unwired: 1 in]
            }
            n143 = Search 1D Array(1D array=w916, element=w917) -> (index of element=w919:i32)  [unwired: 1 out]
            n144 = Equal?(x=w919, y=-1) -> (x = y?=w918:bool)
            n145 = case shown="True" w918 {
              tunnel: w919 -> [_ w928]
              tunnel: w917 -> [w922 _]
              tunnel: w916 -> [_ w929]
              frame True {
                w923 = u32 0 items=["User"] ("AO_Sampling Rate")
                n146 = property on="AO_Sampling User" class="DigNum (strict)"("Visible"=TRUE) -> ()  [unwired: 2 in, 2 out]
                n147 = property on="AO_Sampling User" class="DigNum (strict)"("Value"=w922) -> ()  [unwired: 2 in, 2 out]
                n148 = property on="AO_Sampling Rate" class="Ring (strict)"("Value"=w923) -> ()  [unwired: 2 in, 2 out]
              }
              frame False {
                n149 = Index Array(array=w929, index=w928) -> (element=w926:u32)
                n150 = Equal?(x=w926, y=u32 0) -> (x = y?=w925:bool)
                n151 = property on="AO_Sampling Rate" class="Ring (strict)"("Value"=w926) -> ()  [unwired: 2 in, 2 out]
                n152 = property on="AO_Sampling User" class="DigNum (strict)"("Visible"=w925) -> ()  [unwired: 2 in, 2 out]
              }
            }
          }
        }
        n153 = case shown="0, Default" w883 {
          selector: w883 -> [_ w914]
          frame -1 {
            n154 = property on="AO_Device Name" class="Ring (strict)"("Value"=0) -> ()  [unwired: 2 in, 2 out]
          }
          frame 0, Default {
            n155 = property on="AO_Device Name" class="Ring (strict)"("Value"=w914) -> ()  [unwired: 2 in, 2 out]
          }
        }
        n156 = call "CRYGet Button State.vi"("Channel Name"=w895, "Input/Output"=FALSE) -> ("State"=w894:T7)  [unwired: 8 in, 1 out]
        n157 = property on="AO_Delete" class="Bool"("DisabledEnum"=w894) -> ()  [unwired: 2 in, 2 out]
        n158 = property on="AO_Rename" class="Bool"("DisabledEnum"=w894) -> ()  [unwired: 2 in, 2 out]
      }
      event "AI_SoundCard Channel": Value Change {
        n159 = event-data() -> ("NewVal"=w956:u16)  [unwired: 6 out]
        n160 = local read "I_Channel Info"() -> (w966:T2[])
        n161 = local read "SoundCard"() -> (w952:T5)
        n162 = Bundle By Name(cluster=w952, "SelectedIn"=w956) -> (w951:T5)
        n163 = Index Array(array=w966, index=w956) -> (element=w965:T2)
        n164 = local write "SoundCard"(w951) -> ()
        n165 = Unbundle By Name(w965) -> ("Name"=w949:string, "Digital"=w960:bool, "Device Name"=w955:string, "Hardware Ch ID"=w962:u8, "Vmax (V)"=w963:dbl, "Latency (samples)"=w954:dbl, "Sampling Rate (Hz)"=w958:u32, "Bit Depth"=w964:u32, "Anti-aliasing Factor (%fs)"=w957:sgl, "Audio Driver"=w950:u16)  [unwired: 2 out]
        n166 = flat-sequence {
          tunnel: w950 -> [w988]
          frame #0 {
            n167 = local write "AI_HW_Changed"(TRUE ("HW_Changed")) -> ()
          }
          frame #1 {
            n168 = property on="AI_Audio Driver" class="RadioBtnsControl (strict)"("Val(Sgnl)"=w988) -> ()  [unwired: 2 in, 2 out]
          }
        }
        n169 = local write "AI_Select Channel1"(w962) -> ()
        n170 = local write "AI_Bit Depth"(w964) -> ()
        n171 = local write "AI_Vp"(w963) -> ()
        n172 = local write "AI_Latency"(w954) -> ()
        n173 = local write "AI_Alias freq"(w957) -> ()
        n174 = local read "I_Channel Info"() -> (w946:T2[])
        n175 = local read "I_Device Info"() -> (w945:T3)
        n176 = property on="AI_Audio Driver" class="RadioBtnsControl (strict)"() -> ("Value"=w947:enum32{"Radio Selection 1", "Radio Selection 2"})  [unwired: 2 in, 2 out]
        n177 = Select(t=enum32{"Analog", "Digital"}."Digital" ("AO_Select Channel2"), s=w960, f=enum32{"Analog", "Digital"}."Analog" ("AO_Select Channel2")) -> (s? t:f=w953:enum32{"Analog", "Digital"})
        n178 = property on="AI_Select SMode" class="RadioBtnsControl (strict)"("Val(Sgnl)"=w953) -> ()  [unwired: 2 in, 2 out]
        n179 = call "CRYGet Disable Device State.vi"("I_Channel Info"=w946, "I_Device Info In"=w945, "Audio Driver"=w947, "In/Out"=TRUE) -> ("All I/O_Device Info Out"=w943:T3)  [unwired: 5 in, 2 out]
        n180 = call "CRYGet Device Index to Channel.vi"("Device Name In"=w955, "Device Info In"=w943) -> ("Device Index Out"=w936:i32)  [unwired: 9 out]
        n181 = Index Array(array=w943, index=w936) -> (element=w942:T12)
        n182 = Unbundle By Name(w942) -> ("Channel Names"=w941:string[])
        n183 = Index Array(array=w941) -> (element=w940:string)  [unwired: 1 in]
        n184 = Not Equal?(x=w940, y="No") -> (x != y?=w937:bool)
        n185 = case shown="True" w937 {
          tunnel: w958 -> [_ w970]
          frame False {
          }
          frame True {
            n186 = property on="AI_Sampling Rate" class="Ring (strict)"() -> ("StringsAndValues[]"=w974:T13)  [unwired: 2 in, 2 out]
            n187 = for {
              tunnel: w974 -> [w986] mode=indexing
              shift-right: [w985] -> w969
              shift-left: u32[] [] -> [w983]
              n188 = Unbundle By Name(w986) -> ("Value"=w984:u32)
              n189 = Insert Into Array(array=w983, new element=w984) -> (w985:u32[])  [unwired: 1 in]
            }
            n190 = Search 1D Array(1D array=w969, element=w970) -> (index of element=w972:i32)  [unwired: 1 out]
            n191 = Equal?(x=w972, y=-1) -> (x = y?=w971:bool)
            n192 = case shown="False" w971 {
              tunnel: w972 -> [_ w981]
              tunnel: w970 -> [w975 _]
              tunnel: w969 -> [_ w982]
              frame True {
                w976 = u32 0 items=["User"] ("AO_Sampling Rate")
                n193 = property on="AI_Sampling User" class="DigNum (strict)"("Visible"=TRUE) -> ()  [unwired: 2 in, 2 out]
                n194 = property on="AI_Sampling User" class="DigNum (strict)"("Value"=w975) -> ()  [unwired: 2 in, 2 out]
                n195 = property on="AI_Sampling Rate" class="Ring (strict)"("Value"=w976) -> ()  [unwired: 2 in, 2 out]
              }
              frame False {
                n196 = Index Array(array=w982, index=w981) -> (element=w979:u32)
                n197 = Equal?(x=w979, y=u32 0) -> (x = y?=w978:bool)
                n198 = property on="AI_Sampling Rate" class="Ring (strict)"("Value"=w979) -> ()  [unwired: 2 in, 2 out]
                n199 = property on="AI_Sampling User" class="DigNum (strict)"("Visible"=w978) -> ()  [unwired: 2 in, 2 out]
              }
            }
          }
        }
        n200 = case shown="0, Default" w936 {
          selector: w936 -> [_ w967]
          frame -1 {
          }
          frame 0, Default {
            n201 = property on="AI_Device Name" class="Ring (strict)"("Value"=w967) -> ()  [unwired: 2 in, 2 out]
          }
        }
        n202 = call "CRYGet Button State.vi"("Channel Name"=w949, "Input/Output"=TRUE) -> ("State"=w948:T7)  [unwired: 8 in, 1 out]
        n203 = property on="AI_Delete" class="Bool"("DisabledEnum"=w948) -> ()  [unwired: 2 in, 2 out]
        n204 = property on="AI_Rename" class="Bool"("DisabledEnum"=w948) -> ()  [unwired: 2 in, 2 out]
      }
      event "AO_Audio Driver": Value Change {
        n205 = event-data() -> ("NewVal"=w1002:enum32{"Radio Selection 1", "Radio Selection 2"})  [unwired: 6 out]
        n206 = flat-sequence {
          tunnel: w1002 -> [w1005]
          tunnel: [w1005] -> w1000
          tunnel: [w1003] -> w999
          frame #0 {
            n207 = Equal To 0?(x=w1005) -> (x = 0?=w1010:bool)
            n208 = To Unsigned Long Integer(number=w1005) -> (unsigned 32bit integer=w1008:u32)
            n209 = Select(t=w1008, s=w1010, f=u32 2) -> (s? t:f=w1007:u32)
            n210 = local read "O_Channel Info"() -> (w1003:T2[])
            n211 = property on="AO_SoundCard Channel" class="Ring (strict)"() -> ("Value"=w1017:u16)  [unwired: 2 in, 2 out]
            n212 = To Unsigned Word Integer(number=w1007) -> (unsigned 16bit integer=w1006:u16)
            n213 = Index Array(array=w1003, index=w1017) -> (element=w1016:T2)
            n214 = Bundle By Name(cluster=w1016, "Audio Driver"=w1006) -> (w1015:T2)
            n215 = local read "I_Channel Info"() -> (w1014:T2[])
            n216 = Replace Array Subset(array=w1003, new element=w1015, index=w1017) -> (w1004:T2[])
            n217 = local read "SoundCard"() -> (w1013:T5)
            n218 = local write "O_Channel Info"(w1004) -> ()
            n219 = Insert Into Array(array=w1004, new element=w1014) -> (w1012:T2[])  [unwired: 1 in]
            n220 = Bundle By Name(cluster=w1013, "Channel Array"=w1012, "Out Audio Driver"=w1005) -> (w1011:T5)
            n221 = local write "SoundCard"(w1011) -> ()
          }
        }
        n222 = flat-sequence {
          tunnel: [w1018] -> w1001
          tunnel: [w1019] -> _
          tunnel: [w1018] -> _
          frame #0 {
            n223 = call "CRYClose All Operator.vi"() -> ()  [unwired: 12 in]
          }
          frame #1 {
            n224 = call "CRYGet Default Hardware.vi"() -> ("O_Device Info Out"=w1018:T3, "I_Device Info Out"=w1019:T3)  [unwired: 1 in, 17 out]
            n225 = local write "O_Device Info"(w1018) -> ()
            n226 = local write "I_Device Info"(w1019) -> ()
          }
        }
        n227 = property on="AI_Device Name" class="Ring (strict)"() -> ("Value"=w995:u16)  [unwired: 2 in, 2 out]
        n228 = property on="AI_Device Name" class="Ring (strict)"() -> ("Disabled Items []"=w996:i32[])  [unwired: 2 in, 2 out]
        n229 = case shown="\"Radio Selection 2\"" w1000 {
          tunnel: w1001 -> [_ _]
          tunnel: w999 -> [w1033 w1075]
          tunnel: [w1021 w1065] -> w998
          tunnel: [w1020 w1064] -> w993
          frame "Radio Selection 1", Default {
            n230 = property on="AO_Audio Driver" class="RadioBtnsControl (strict)"() -> ("Value"=w1029:enum32{"Radio Selection 1", "Radio Selection 2"})  [unwired: 2 in, 2 out]
            n231 = local read "O_Device Info"() -> (w1031:T3)
            n232 = property on="Advanced View" class="Bool (strict)"() -> ("Value"=w1032:bool)  [unwired: 2 in, 2 out]
            n233 = case shown="True" w1032 {
              frame False {
              }
              frame True {
                n234 = property on="AO_Launch" class="Bool (strict)"("Visible"=FALSE) -> ()  [unwired: 2 in, 2 out]
              }
            }
            n235 = call "CRYGet Disable Device State.vi"("O_Channel Info"=w1033, "O_Device Info In"=w1031, "Audio Driver"=w1029, "In/Out"=FALSE) -> ("All I/O_Device Info Out"=w1030:T3, "Device Names"=w1028:string[], "Disabled Items"=w1023:i32[])  [unwired: 5 in]
            n236 = flat-sequence {
              tunnel: w1028 -> [w1039]
              tunnel: [w1039] -> _
              tunnel: [w1037] -> w1022
              tunnel: w1023 -> [w1044]
              tunnel: [w1044] -> w1027
              frame #0 {
                n237 = local read "AO_HW_Changed"() -> (w1038:bool)
                n238 = property on="AO_Device Name" class="Ring (strict)"("Strings []"=w1039) -> ()  [unwired: 2 in, 2 out]
                n239 = case shown="True" w1038 {
                  tunnel: [w1040 w1042] -> w1037
                  frame False {
                    w1040 = 0
                    n240 = property on="AO_Device Name" class="Ring (strict)"("Val(Sgnl)"=w1040) -> (error out=w1041:errorcluster)  [unwired: 2 in, 1 out]
                    n241 = property on="AO_Select Channel1" class="Ring (strict)"(error in=w1041, "Val(Sgnl)"=w1040) -> ()  [unwired: 1 in, 2 out]
                  }
                  frame True {
                    n242 = property on="AO_Device Name" class="Ring (strict)"() -> ("Value"=w1042:u16)  [unwired: 2 in, 2 out]
                    n243 = local write "AO_HW_Changed"(FALSE ("HW_Changed")) -> ()
                  }
                }
              }
              frame #1 {
                n244 = property on="AO_Device Name" class="Ring (strict)"("Disabled Items []"=w1044) -> ()  [unwired: 2 in, 2 out]
              }
            }
            n245 = Search 1D Array(1D array=w1023, element=w1022) -> (index of element=w1024:i32)  [unwired: 1 in]
            n246 = Less Than 0?(x=w1024) -> (x < 0?=w1020:bool)
            n247 = Select(t=T7."Enabled" ("Disabled"), s=w1020, f=T7."Disabled and Grayed Out" ("Disabled")) -> (s? t:f=w1021:T7)
            n248 = Array Size(array=w1028) -> (size(s)=w1035:i32)
            n249 = case shown="1, Default" w1035 {
              tunnel: w1030 -> [_ w1063]
              tunnel: w1027 -> [_ _]
              tunnel: w1022 -> [_ w1053]
              frame 0 {
                n250 = local read "O_Channel Info"() -> (w1047:T2[])
                n251 = property on="AO_SoundCard Channel" class="Ring (strict)"() -> ("Value"=w1046:u16)  [unwired: 2 in, 2 out]
                n252 = property on="AO_Select Channel1" class="Ring (strict)"("Strings []"=string[] []) -> ()  [unwired: 2 in, 2 out]
                n253 = Index Array(array=w1047, index=w1046) -> (element=w1048:T2)
                n254 = Bundle By Name(cluster=w1048, "Device Name"="") -> (w1049:T2)
                n255 = Replace Array Subset(array=w1047, new element=w1049, index=w1046) -> (w1050:T2[])
                n256 = property on="AO_Sampling Rate" class="Ring (strict)"("StringsAndValues[]"=cluster{"String":string, "Value":ext}[] []) -> ()  [unwired: 2 in, 2 out]
                n257 = local write "O_Channel Info"(w1050) -> ()
              }
              frame 1, Default {
                n258 = local read "O_Channel Info"() -> (w1056:T2[])
                n259 = property on="AO_SoundCard Channel" class="Ring (strict)"() -> ("Value"=w1054:u16)  [unwired: 2 in, 2 out]
                n260 = property on="AO_Device Name" class="Ring (strict)"() -> ("RingText.Text"=w1055:string)  [unwired: 2 in, 2 out]
                n261 = Index Array(array=w1063, index=w1053) -> (element=w1060:T12)
                n262 = Unbundle By Name(w1060) -> ("Channel Names"=w1062:string[])
                n263 = call "CRYGet Freq Bit Array.vi"("Device Infor"=w1060) -> ("Samplein Rate"=w1061:cluster{"String":string, "Value":ext}[])  [unwired: 1 in, 9 out]
                n264 = Index Array(array=w1056, index=w1054) -> (element=w1057:T2)
                n265 = Bundle By Name(cluster=w1057, "Device Name"=w1055) -> (w1058:T2)
                n266 = property on="AO_Sampling Rate" class="Ring (strict)"("StringsAndValues[]"=w1061) -> ()  [unwired: 2 in, 2 out]
                n267 = Replace Array Subset(array=w1056, new element=w1058, index=w1054) -> (w1059:T2[])
                n268 = property on="AO_Select Channel1" class="Ring (strict)"("Strings []"=w1062) -> ()  [unwired: 2 in, 2 out]
                n269 = local write "O_Channel Info"(w1059) -> ()
              }
            }
          }
          frame "Radio Selection 2" {
            n270 = local read "O_Device Info"() -> (w1074:T3)
            n271 = property on="Advanced View" class="Bool (strict)"() -> ("Value"=w1077:bool)  [unwired: 2 in, 2 out]
            n272 = property on="AO_Audio Driver" class="RadioBtnsControl (strict)"() -> ("Value"=w1072:enum32{"Radio Selection 1", "Radio Selection 2"})  [unwired: 2 in, 2 out]
            n273 = case shown="True" w1077 {
              frame False {
              }
              frame True {
                n274 = property on="AO_Launch" class="Bool (strict)"("Visible"=TRUE) -> ()  [unwired: 2 in, 2 out]
              }
            }
            n275 = call "CRYGet Disable Device State.vi"("O_Channel Info"=w1075, "O_Device Info In"=w1074, "Audio Driver"=w1072, "In/Out"=FALSE) -> ("All I/O_Device Info Out"=w1073:T3, "Device Names"=w1071:string[], "Disabled Items"=w1067:i32[])  [unwired: 5 in]
            n276 = flat-sequence {
              tunnel: w1071 -> [w1080]
              tunnel: [w1081] -> w1066
              tunnel: w1067 -> [w1087]
              frame #0 {
                n277 = local read "AO_HW_Changed"() -> (w1082:bool)
                n278 = property on="AO_Device Name" class="Ring (strict)"("Strings []"=w1080) -> ()  [unwired: 2 in, 2 out]
                n279 = case shown="False" w1082 {
                  tunnel: [w1083 w1085] -> w1081
                  frame False {
                    w1083 = 0
                    n280 = property on="AO_Device Name" class="Ring (strict)"("Val(Sgnl)"=w1083) -> (error out=w1084:errorcluster)  [unwired: 2 in, 1 out]
                    n281 = property on="AO_Select Channel1" class="Ring (strict)"(error in=w1084, "Val(Sgnl)"=w1083) -> ()  [unwired: 1 in, 2 out]
                  }
                  frame True {
                    n282 = property on="AO_Device Name" class="Ring (strict)"() -> ("Value"=w1085:u16)  [unwired: 2 in, 2 out]
                    n283 = local write "AO_HW_Changed"(FALSE ("HW_Changed")) -> ()
                  }
                }
              }
              frame #1 {
                n284 = property on="AO_Device Name" class="Ring (strict)"("Disabled Items []"=w1087) -> ()  [unwired: 2 in, 2 out]
              }
            }
            n285 = Search 1D Array(1D array=w1067, element=w1066) -> (index of element=w1068:i32)  [unwired: 1 in]
            n286 = Less Than 0?(x=w1068) -> (x < 0?=w1064:bool)
            n287 = Select(t=T7."Enabled" ("Disabled"), s=w1064, f=T7."Disabled and Grayed Out" ("Disabled")) -> (s? t:f=w1065:T7)
            n288 = Array Size(array=w1071) -> (size(s)=w1078:i32)
            n289 = case shown="1, Default" w1078 {
              tunnel: w1073 -> [_ w1106]
              tunnel: w1066 -> [_ w1096]
              frame 0 {
                n290 = local read "O_Channel Info"() -> (w1090:T2[])
                n291 = property on="AO_SoundCard Channel" class="Ring (strict)"() -> ("Value"=w1089:u16)  [unwired: 2 in, 2 out]
                n292 = property on="AO_Select Channel1" class="Ring (strict)"("Strings []"=string[] []) -> ()  [unwired: 2 in, 2 out]
                n293 = Index Array(array=w1090, index=w1089) -> (element=w1091:T2)
                n294 = Bundle By Name(cluster=w1091, "Device Name"="") -> (w1092:T2)
                n295 = Replace Array Subset(array=w1090, new element=w1092, index=w1089) -> (w1093:T2[])
                n296 = property on="AO_Sampling Rate" class="Ring (strict)"("StringsAndValues[]"=cluster{"String":string, "Value":ext}[] []) -> ()  [unwired: 2 in, 2 out]
                n297 = local write "O_Channel Info"(w1093) -> ()
              }
              frame 1, Default {
                n298 = local read "O_Channel Info"() -> (w1099:T2[])
                n299 = property on="AO_SoundCard Channel" class="Ring (strict)"() -> ("Value"=w1097:u16)  [unwired: 2 in, 2 out]
                n300 = property on="AO_Device Name" class="Ring (strict)"() -> ("RingText.Text"=w1098:string)  [unwired: 2 in, 2 out]
                n301 = Index Array(array=w1106, index=w1096) -> (element=w1103:T12)
                n302 = Unbundle By Name(w1103) -> ("Channel Names"=w1105:string[])
                n303 = call "CRYGet Freq Bit Array.vi"("Device Infor"=w1103) -> ("Samplein Rate"=w1104:cluster{"String":string, "Value":ext}[])  [unwired: 1 in, 9 out]
                n304 = Index Array(array=w1099, index=w1097) -> (element=w1100:T2)
                n305 = Bundle By Name(cluster=w1100, "Device Name"=w1098) -> (w1101:T2)
                n306 = property on="AO_Sampling Rate" class="Ring (strict)"("StringsAndValues[]"=w1104) -> ()  [unwired: 2 in, 2 out]
                n307 = Replace Array Subset(array=w1099, new element=w1101, index=w1097) -> (w1102:T2[])
                n308 = property on="AO_Select Channel1" class="Ring (strict)"("Strings []"=w1105) -> ()  [unwired: 2 in, 2 out]
                n309 = local write "O_Channel Info"(w1102) -> ()
              }
            }
          }
        }
        n310 = Search 1D Array(1D array=w996, element=w995) -> (index of element=w997:i32)  [unwired: 1 in]
        n311 = Less Than 0?(x=w997) -> (x < 0?=w994:bool)
        n312 = And(x=w993, y=w994) -> (x .and. y?=w990:bool)
        n313 = Select(t=T7."Enabled" ("Disabled"), s=w990, f=T7."Disabled and Grayed Out" ("Disabled")) -> (s? t:f=w989:T7)
        n314 = property on="Calibration Seq" class="Ring (strict)"("DisabledEnum"=w989) -> ()  [unwired: 2 in, 2 out]
        n315 = property on="Calibrartion" class="Bool (strict)"("DisabledEnum"=w989) -> ()  [unwired: 2 in, 2 out]
        n316 = property on="AO_Launch" class="Bool (strict)"("DisabledEnum"=w998) -> ()  [unwired: 2 in, 2 out]
        n317 = property on="AO_Sampling Rate" class="Ring (strict)"("DisabledEnum"=w998) -> ()  [unwired: 2 in, 2 out]
        n318 = property on="AO_Alias freq" class="DigNum (strict)"("DisabledEnum"=w998) -> ()  [unwired: 2 in, 2 out]
        n319 = property on="AO_Select SMode" class="RadioBtnsControl (strict)"("DisabledEnum"=w998) -> ()  [unwired: 2 in, 2 out]
        n320 = property on="AO_Sampling User" class="DigNum (strict)"("DisabledEnum"=w998) -> ()  [unwired: 2 in, 2 out]
        n321 = property on="AO_Vp" class="DigNum (strict)"("DisabledEnum"=w998) -> ()  [unwired: 2 in, 2 out]
        n322 = property on="AO_Select Channel1" class="Ring (strict)"("DisabledEnum"=w998) -> ()  [unwired: 2 in, 2 out]
        n323 = property on="AO_Bit Depth" class="Ring (strict)"("DisabledEnum"=w998) -> ()  [unwired: 2 in, 2 out]
      }
      event "AI_Audio Driver": Value Change {
        n324 = event-data() -> ("NewVal"=w1119:enum32{"Radio Selection 1", "Radio Selection 2"})  [unwired: 6 out]
        n325 = flat-sequence {
          tunnel: w1119 -> [w1123]
          tunnel: [w1123] -> w1118
          tunnel: [w1121] -> w1117
          frame #0 {
            n326 = Equal To 0?(x=w1123) -> (x = 0?=w1130:bool)
            n327 = To Unsigned Long Integer(number=w1123) -> (unsigned 32bit integer=w1128:u32)
            n328 = property on="AI_SoundCard Channel" class="Ring (strict)"() -> ("Value"=w1125:u16)  [unwired: 2 in, 2 out]
            n329 = local read "I_Channel Info"() -> (w1121:T2[])
            n330 = Select(t=w1128, s=w1130, f=u32 2) -> (s? t:f=w1127:u32)
            n331 = To Unsigned Word Integer(number=w1127) -> (unsigned 16bit integer=w1126:u16)
            n332 = Index Array(array=w1121, index=w1125) -> (element=w1135:T2)
            n333 = Bundle By Name(cluster=w1135, "Audio Driver"=w1126) -> (w1134:T2)
            n334 = Replace Array Subset(array=w1121, new element=w1134, index=w1125) -> (w1122:T2[])
            n335 = local read "O_Channel Info"() -> (w1124:T2[])
            n336 = local read "SoundCard"() -> (w1133:T5)
            n337 = local write "I_Channel Info"(w1122) -> ()
            n338 = Insert Into Array(array=w1124, new element=w1122) -> (w1132:T2[])  [unwired: 1 in]
            n339 = Bundle By Name(cluster=w1133, "Channel Array"=w1132, "In Audio Driver"=w1123) -> (w1131:T5)
            n340 = local write "SoundCard"(w1131) -> ()
          }
        }
        n341 = flat-sequence {
          tunnel: [w1136] -> w1120
          frame #0 {
            n342 = call "CRYClose All Operator.vi"() -> ()  [unwired: 12 in]
          }
          frame #1 {
            n343 = call "CRYGet Default Hardware.vi"() -> ("O_Device Info Out"=w1136:T3, "I_Device Info Out"=w1137:T3)  [unwired: 1 in, 17 out]
            n344 = local write "O_Device Info"(w1136) -> ()
            n345 = local write "I_Device Info"(w1137) -> ()
          }
        }
        n346 = property on="AO_Device Name" class="Ring (strict)"() -> ("Disabled Items []"=w1112:i32[])  [unwired: 2 in, 2 out]
        n347 = property on="AO_Device Name" class="Ring (strict)"() -> ("Value"=w1111:u16)  [unwired: 2 in, 2 out]
        n348 = Search 1D Array(1D array=w1112, element=w1111) -> (index of element=w1113:i32)  [unwired: 1 in]
        n349 = Less Than 0?(x=w1113) -> (x < 0?=w1110:bool)
        n350 = case shown="\"Radio Selection 2\"" w1118 {
          tunnel: w1120 -> [_ _]
          tunnel: w1117 -> [w1149 w1191]
          tunnel: [w1141 w1182] -> w1116
          tunnel: [w1138 w1181] -> w1109
          frame "Radio Selection 2" {
            n351 = local read "I_Device Info"() -> (w1148:T3)
            n352 = property on="Advanced View" class="Bool (strict)"() -> ("Value"=w1151:bool)  [unwired: 2 in, 2 out]
            n353 = property on="AI_Audio Driver" class="RadioBtnsControl (strict)"() -> ("Value"=w1146:enum32{"Radio Selection 1", "Radio Selection 2"})  [unwired: 2 in, 2 out]
            n354 = case shown="True" w1151 {
              frame False {
              }
              frame True {
                n355 = property on="AI_Launch" class="Bool (strict)"("Visible"=TRUE) -> ()  [unwired: 2 in, 2 out]
              }
            }
            n356 = call "CRYGet Disable Device State.vi"("I_Channel Info"=w1149, "I_Device Info In"=w1148, "Audio Driver"=w1146, "In/Out"=TRUE) -> ("All I/O_Device Info Out"=w1147:T3, "Device Names"=w1145:string[], "Disabled Items"=w1140:i32[])  [unwired: 5 in]
            n357 = Search 1D Array(1D array=w1140, element=w1139) -> (index of element=w1142:i32)  [unwired: 1 in]
            n358 = flat-sequence {
              tunnel: [w1154] -> _
              tunnel: [w1155] -> w1139
              tunnel: w1145 -> [w1154]
              tunnel: w1140 -> [w1161]
              frame #0 {
                n359 = local read "AI_HW_Changed"() -> (w1156:bool)
                n360 = property on="AI_Device Name" class="Ring (strict)"("Strings []"=w1154) -> ()  [unwired: 2 in, 2 out]
                n361 = case shown="False" w1156 {
                  tunnel: [w1157 w1159] -> w1155
                  frame False {
                    w1157 = 0
                    n362 = property on="AI_Device Name" class="Ring (strict)"("Val(Sgnl)"=w1157) -> (error out=w1158:errorcluster)  [unwired: 2 in, 1 out]
                    n363 = property on="AI_Select Channel1" class="Ring (strict)"(error in=w1158, "Val(Sgnl)"=w1157) -> ()  [unwired: 1 in, 2 out]
                  }
                  frame True {
                    n364 = property on="AI_Device Name" class="Ring (strict)"() -> ("Value"=w1159:u16)  [unwired: 2 in, 2 out]
                    n365 = local write "AI_HW_Changed"(FALSE ("HW_Changed")) -> ()
                  }
                }
              }
              frame #1 {
                n366 = property on="AI_Device Name" class="Ring (strict)"("Disabled Items []"=w1161) -> ()  [unwired: 2 in, 2 out]
              }
            }
            n367 = Less Than 0?(x=w1142) -> (x < 0?=w1138:bool)
            n368 = Select(t=T7."Enabled" ("Disabled"), s=w1138, f=T7."Disabled and Grayed Out" ("Disabled")) -> (s? t:f=w1141:T7)
            n369 = Array Size(array=w1145) -> (size(s)=w1152:i32)
            n370 = case shown="1, Default" w1152 {
              tunnel: w1147 -> [_ w1180]
              tunnel: w1139 -> [_ w1170]
              frame 0 {
                n371 = local read "I_Channel Info"() -> (w1162:T2[])
                n372 = property on="AI_SoundCard Channel" class="Ring (strict)"() -> ("Value"=w1165:u16)  [unwired: 2 in, 2 out]
                n373 = property on="AI_Select Channel1" class="Ring (strict)"("Strings []"=string[] []) -> ()  [unwired: 2 in, 2 out]
                n374 = Index Array(array=w1162, index=w1165) -> (element=w1163:T2)
                n375 = Bundle By Name(cluster=w1163, "Device Name"="") -> (w1164:T2)
                n376 = Replace Array Subset(array=w1162, new element=w1164, index=w1165) -> (w1166:T2[])
                n377 = property on="AI_Sampling Rate" class="Ring (strict)"("StringsAndValues[]"=cluster{"String":string, "Value":ext}[] []) -> ()  [unwired: 2 in, 2 out]
                n378 = local write "I_Channel Info"(w1166) -> ()
              }
              frame 1, Default {
                n379 = property on="AI_Device Name" class="Ring (strict)"() -> ("RingText.Text"=w1171:string)  [unwired: 2 in, 2 out]
                n380 = local read "I_Channel Info"() -> (w1172:T2[])
                n381 = property on="AI_SoundCard Channel" class="Ring (strict)"() -> ("Value"=w1175:u16)  [unwired: 2 in, 2 out]
                n382 = Index Array(array=w1180, index=w1170) -> (element=w1179:T12)
                n383 = Unbundle By Name(w1179) -> ("Channel Names"=w1177:string[])
                n384 = call "CRYGet Freq Bit Array.vi"("Device Infor"=w1179) -> ("Samplein Rate"=w1178:cluster{"String":string, "Value":ext}[])  [unwired: 1 in, 9 out]
                n385 = Index Array(array=w1172, index=w1175) -> (element=w1173:T2)
                n386 = Bundle By Name(cluster=w1173, "Device Name"=w1171) -> (w1174:T2)
                n387 = property on="AI_Sampling Rate" class="Ring (strict)"("StringsAndValues[]"=w1178) -> ()  [unwired: 2 in, 2 out]
                n388 = Replace Array Subset(array=w1172, new element=w1174, index=w1175) -> (w1176:T2[])
                n389 = property on="AI_Select Channel1" class="Ring (strict)"("Strings []"=w1177) -> ()  [unwired: 2 in, 2 out]
                n390 = local write "I_Channel Info"(w1176) -> ()
              }
            }
          }
          frame "Radio Selection 1", Default {
            n391 = local read "I_Device Info"() -> (w1192:T3)
            n392 = property on="AI_Audio Driver" class="RadioBtnsControl (strict)"() -> ("Value"=w1189:enum32{"Radio Selection 1", "Radio Selection 2"})  [unwired: 2 in, 2 out]
            n393 = property on="Advanced View" class="Bool (strict)"() -> ("Value"=w1194:bool)  [unwired: 2 in, 2 out]
            n394 = case shown="True" w1194 {
              frame False {
              }
              frame True {
                n395 = property on="AI_Launch" class="Bool (strict)"("Visible"=FALSE) -> ()  [unwired: 2 in, 2 out]
              }
            }
            n396 = call "CRYGet Disable Device State.vi"("I_Channel Info"=w1191, "I_Device Info In"=w1192, "Audio Driver"=w1189, "In/Out"=TRUE) -> ("All I/O_Device Info Out"=w1190:T3, "Device Names"=w1188:string[], "Disabled Items"=w1187:i32[])  [unwired: 5 in]
            n397 = flat-sequence {
              tunnel: w1188 -> [w1199]
              tunnel: [w1197] -> w1186
              tunnel: w1187 -> [w1204]
              frame #0 {
                n398 = local read "AI_HW_Changed"() -> (w1198:bool)
                n399 = property on="AI_Device Name" class="Ring (strict)"("Strings []"=w1199) -> ()  [unwired: 2 in, 2 out]
                n400 = case shown="True" w1198 {
                  tunnel: [w1200 w1202] -> w1197
                  frame False {
                    w1200 = 0
                    n401 = property on="AI_Device Name" class="Ring (strict)"("Val(Sgnl)"=w1200) -> (error out=w1201:errorcluster)  [unwired: 2 in, 1 out]
                    n402 = property on="AI_Select Channel1" class="Ring (strict)"(error in=w1201, "Val(Sgnl)"=w1200) -> ()  [unwired: 1 in, 2 out]
                  }
                  frame True {
                    n403 = property on="AI_Device Name" class="Ring (strict)"() -> ("Value"=w1202:u16)  [unwired: 2 in, 2 out]
                    n404 = local write "AI_HW_Changed"(FALSE ("HW_Changed")) -> ()
                  }
                }
              }
              frame #1 {
                n405 = property on="AI_Device Name" class="Ring (strict)"("Disabled Items []"=w1204) -> ()  [unwired: 2 in, 2 out]
              }
            }
            n406 = Search 1D Array(1D array=w1187, element=w1186) -> (index of element=w1183:i32)  [unwired: 1 in]
            n407 = Less Than 0?(x=w1183) -> (x < 0?=w1181:bool)
            n408 = Select(t=T7."Enabled" ("Disabled"), s=w1181, f=T7."Disabled and Grayed Out" ("Disabled")) -> (s? t:f=w1182:T7)
            n409 = Array Size(array=w1188) -> (size(s)=w1195:i32)
            n410 = case shown="1, Default" w1195 {
              tunnel: w1190 -> [_ w1223]
              tunnel: w1186 -> [_ w1213]
              frame 0 {
                n411 = local read "I_Channel Info"() -> (w1205:T2[])
                n412 = property on="AI_SoundCard Channel" class="Ring (strict)"() -> ("Value"=w1208:u16)  [unwired: 2 in, 2 out]
                n413 = property on="AI_Select Channel1" class="Ring (strict)"("Strings []"=string[] []) -> ()  [unwired: 2 in, 2 out]
                n414 = Index Array(array=w1205, index=w1208) -> (element=w1206:T2)
                n415 = Bundle By Name(cluster=w1206, "Device Name"="") -> (w1207:T2)
                n416 = Replace Array Subset(array=w1205, new element=w1207, index=w1208) -> (w1209:T2[])
                n417 = property on="AI_Sampling Rate" class="Ring (strict)"("StringsAndValues[]"=cluster{"String":string, "Value":ext}[] []) -> ()  [unwired: 2 in, 2 out]
                n418 = local write "I_Channel Info"(w1209) -> ()
              }
              frame 1, Default {
                n419 = property on="AI_Device Name" class="Ring (strict)"() -> ("RingText.Text"=w1214:string)  [unwired: 2 in, 2 out]
                n420 = local read "I_Channel Info"() -> (w1215:T2[])
                n421 = property on="AI_SoundCard Channel" class="Ring (strict)"() -> ("Value"=w1218:u16)  [unwired: 2 in, 2 out]
                n422 = Index Array(array=w1223, index=w1213) -> (element=w1222:T12)
                n423 = call "CRYGet Freq Bit Array.vi"("Device Infor"=w1222) -> ("Samplein Rate"=w1221:cluster{"String":string, "Value":ext}[])  [unwired: 1 in, 9 out]
                n424 = Unbundle By Name(w1222) -> ("Channel Names"=w1220:string[])
                n425 = Index Array(array=w1215, index=w1218) -> (element=w1216:T2)
                n426 = Bundle By Name(cluster=w1216, "Device Name"=w1214) -> (w1217:T2)
                n427 = property on="AI_Sampling Rate" class="Ring (strict)"("StringsAndValues[]"=w1221) -> ()  [unwired: 2 in, 2 out]
                n428 = Replace Array Subset(array=w1215, new element=w1217, index=w1218) -> (w1219:T2[])
                n429 = property on="AI_Select Channel1" class="Ring (strict)"("Strings []"=w1220) -> ()  [unwired: 2 in, 2 out]
                n430 = local write "I_Channel Info"(w1219) -> ()
              }
            }
          }
        }
        n431 = And(x=w1109, y=w1110) -> (x .and. y?=w1108:bool)
        n432 = Select(t=T7."Enabled" ("Disabled"), s=w1108, f=T7."Disabled and Grayed Out" ("Disabled")) -> (s? t:f=w1107:T7)
        n433 = property on="Calibration Seq" class="Ring (strict)"("DisabledEnum"=w1107) -> ()  [unwired: 2 in, 2 out]
        n434 = property on="Calibrartion" class="Bool (strict)"("DisabledEnum"=w1107) -> ()  [unwired: 2 in, 2 out]
        n435 = property on="AI_Launch" class="Bool (strict)"("DisabledEnum"=w1116) -> ()  [unwired: 2 in, 2 out]
        n436 = property on="AI_Latency" class="DigNum (strict)"("DisabledEnum"=w1116) -> ()  [unwired: 2 in, 2 out]
        n437 = property on="AI_Sampling Rate" class="Ring (strict)"("DisabledEnum"=w1116) -> ()  [unwired: 2 in, 2 out]
        n438 = property on="AI_Alias freq" class="DigNum (strict)"("DisabledEnum"=w1116) -> ()  [unwired: 2 in, 2 out]
        n439 = property on="AI_Select Channel1" class="Ring (strict)"("DisabledEnum"=w1116) -> ()  [unwired: 2 in, 2 out]
        n440 = property on="AI_Select SMode" class="RadioBtnsControl (strict)"("DisabledEnum"=w1116) -> ()  [unwired: 2 in, 2 out]
        n441 = property on="AI_Sampling User" class="DigNum (strict)"("DisabledEnum"=w1116) -> ()  [unwired: 2 in, 2 out]
        n442 = property on="AI_Vp" class="DigNum (strict)"("DisabledEnum"=w1116) -> ()  [unwired: 2 in, 2 out]
        n443 = property on="AI_Bit Depth" class="Ring (strict)"("DisabledEnum"=w1116) -> ()  [unwired: 2 in, 2 out]
      }
      event "Advanced View": Value Change {
        n444 = event-data() -> ("NewVal"=w1225:bool)  [unwired: 6 out]
        n445 = property on="AO_Sampling Rate" class="Ring (strict)"("Visible"=w1225) -> ()  [unwired: 2 in, 2 out]
        n446 = property on="AO_Alias freq" class="DigNum (strict)"("Visible"=w1225) -> ()  [unwired: 2 in, 2 out]
        n447 = property on="AO_Bit Depth" class="Ring (strict)"("Visible"=w1225) -> ()  [unwired: 2 in, 2 out]
        n448 = property on="AO_Sampling Rate" class="Ring (strict)"() -> ("Value"=w1226:u32)  [unwired: 2 in, 2 out]
        n449 = property on="AO_Device Name" class="Ring (strict)"("Visible"=w1225) -> ()  [unwired: 2 in, 2 out]
        n450 = property on="AO_Select SMode" class="RadioBtnsControl (strict)"("Visible"=w1225) -> ()  [unwired: 2 in, 2 out]
        n451 = property on="Advance Out Rect" class="Bool (strict)"("Visible"=w1225) -> ()  [unwired: 2 in, 2 out]
        n452 = case shown="True" w1225 {
          frame False {
            w1239 = FALSE ("Visible")
            n453 = property on="AO_%FSD" class="DigNum (strict)"("Visible"=w1239) -> ()  [unwired: 2 in, 2 out]
            n454 = property on="AO_Vp" class="DigNum (strict)"("Visible"=w1239) -> ()  [unwired: 2 in, 2 out]
          }
          frame True {
            n455 = property on="AO_Select SMode" class="RadioBtnsControl (strict)"() -> ("Value"=w1243:enum32{"Analog", "Digital"})  [unwired: 2 in, 2 out]
            n456 = Equal?(x=w1243, y=enum32{"Analog", "Digital"}."Digital") -> (x = y?=w1241:bool)
            n457 = Not(x=w1241) -> (.not. x?=w1240:bool)
            n458 = property on="AO_%FSD" class="DigNum (strict)"("Visible"=w1241) -> ()  [unwired: 2 in, 2 out]
            n459 = property on="AO_Vp" class="DigNum (strict)"("Visible"=w1240) -> ()  [unwired: 2 in, 2 out]
          }
        }
        n460 = Equal?(x=w1226, y=u32 0) -> (x = y?=w1228:bool)
        n461 = And(x=w1228, y=w1225) -> (x .and. y?=w1227:bool)
        n462 = property on="AO_Sampling User" class="DigNum (strict)"("Visible"=w1227) -> ()  [unwired: 2 in, 2 out]
        n463 = property on="AO_Select Channel1" class="Ring (strict)"("Visible"=w1225) -> ()  [unwired: 2 in, 2 out]
        n464 = property on="Advance In Rect" class="Bool (strict)"("Visible"=w1225) -> ()  [unwired: 2 in, 2 out]
        n465 = property on="AI_Device Name" class="Ring (strict)"("Visible"=w1225) -> ()  [unwired: 2 in, 2 out]
        n466 = property on="AI_Select SMode" class="RadioBtnsControl (strict)"("Visible"=w1225) -> ()  [unwired: 2 in, 2 out]
        n467 = property on="AI_Sampling Rate" class="Ring (strict)"("Visible"=w1225) -> ()  [unwired: 2 in, 2 out]
        n468 = property on="AI_Alias freq" class="DigNum (strict)"("Visible"=w1225) -> ()  [unwired: 2 in, 2 out]
        n469 = property on="AI_Bit Depth" class="Ring (strict)"("Visible"=w1225) -> ()  [unwired: 2 in, 2 out]
        n470 = property on="AI_Sampling Rate" class="Ring (strict)"() -> ("Value"=w1231:u32)  [unwired: 2 in, 2 out]
        n471 = property on="AI_Select Channel1" class="Ring (strict)"("Visible"=w1225) -> ()  [unwired: 2 in, 2 out]
        n472 = Equal?(x=w1231, y=u32 0) -> (x = y?=w1233:bool)
        n473 = case shown="False" w1225 {
          frame False {
            w1244 = FALSE ("Visible")
            n474 = property on="AI_Vp" class="DigNum (strict)"("Visible"=w1244) -> ()  [unwired: 2 in, 2 out]
            n475 = property on="AI_%FSD" class="DigNum (strict)"("Visible"=w1244) -> ()  [unwired: 2 in, 2 out]
          }
          frame True {
            n476 = property on="AI_Select SMode" class="RadioBtnsControl (strict)"() -> ("Value"=w1247:enum32{"Analog", "Digital"})  [unwired: 2 in, 2 out]
            n477 = Equal?(x=w1247, y=enum32{"Analog", "Digital"}."Digital") -> (x = y?=w1245:bool)
            n478 = Not(x=w1245) -> (.not. x?=w1246:bool)
            n479 = property on="AI_Vp" class="DigNum (strict)"("Visible"=w1246) -> ()  [unwired: 2 in, 2 out]
            n480 = property on="AI_%FSD" class="DigNum (strict)"("Visible"=w1245) -> ()  [unwired: 2 in, 2 out]
          }
        }
        n481 = And(x=w1233, y=w1225) -> (x .and. y?=w1230:bool)
        n482 = disable-structure shown="Disabled" {
          disable-tunnel: w1225 -> [w1238 _]
          frame Disabled {
            n483 = property on="Calibration Seq" class="Ring (strict)"("Visible"=w1238) -> ()  [unwired: 2 in, 2 out]
            n484 = property on="Calibrartion" class="Bool (strict)"("Visible"=w1238) -> ()  [unwired: 2 in, 2 out]
          }
          frame Enabled {
          }
        }
        n485 = property on="AI_Latency" class="DigNum (strict)"("Visible"=w1225) -> ()  [unwired: 2 in, 2 out]
        n486 = local read "AO_Audio Driver"() -> (w1224:enum32{"Radio Selection 1", "Radio Selection 2"})
        n487 = property on="AI_Sampling User" class="DigNum (strict)"("Visible"=w1230) -> ()  [unwired: 2 in, 2 out]
        n488 = local read "SoundCard"() -> (w1235:T5)
        n489 = Bundle By Name(cluster=w1235, "Advanced"=w1225) -> (w1234:T5)
        n490 = local write "SoundCard"(w1234) -> ()
        n491 = case shown="\"Radio Selection 2\"" w1224 {
          tunnel: w1225 -> [_ w1237]
          frame "Radio Selection 1", Default {
            w1236 = FALSE ("Visible")
            n492 = property on="AO_Launch" class="Bool (strict)"("Visible"=w1236) -> ()  [unwired: 2 in, 2 out]
            n493 = property on="AI_Launch" class="Bool (strict)"("Visible"=w1236) -> ()  [unwired: 2 in, 2 out]
          }
          frame "Radio Selection 2" {
            n494 = property on="AO_Launch" class="Bool (strict)"("Visible"=w1237) -> ()  [unwired: 2 in, 2 out]
            n495 = property on="AI_Launch" class="Bool (strict)"("Visible"=w1237) -> ()  [unwired: 2 in, 2 out]
          }
        }
      }
      event "AO_Device Name": Value Change {
        n496 = event-data() -> ("NewVal"=w1279:u16)  [unwired: 6 out]
        n497 = local read "O_Device Info"() -> (w1267:T3)
        n498 = for {
          tunnel: w1267 -> [w1300] mode=indexing
          shift-right: [w1298] -> w1265
          shift-left: T3 [] ("O_Device Info") -> [w1299]
          n499 = local read "AO_Audio Driver"() -> (w1302:enum32{"Radio Selection 1", "Radio Selection 2"})
          n500 = Unbundle By Name(w1300) -> ("Driver Type"=w1301:string)
          n501 = case shown="\"Radio Selection 2\"" w1302 {
            tunnel: w1301 -> [w1308 w1318]
            tunnel: w1300 -> [w1305 w1315]
            tunnel: w1299 -> [w1304 w1314]
            tunnel: [w1303 w1313] -> w1298
            frame "Radio Selection 1", Default {
              n502 = Equal?(x=w1308, y="MME") -> (x = y?=w1306:bool)
              n503 = case shown="True" w1306 {
                tunnel: w1305 -> [_ w1312]
                tunnel: w1304 -> [w1309 w1311]
                tunnel: [w1309 w1310] -> w1303
                frame False {
                }
                frame True {
                  n504 = Build Array (concatenate)(w1311, w1312) -> (w1310:T3)
                }
              }
            }
            frame "Radio Selection 2" {
              n505 = Equal?(x=w1318, y="ASIO") -> (x = y?=w1316:bool)
              n506 = case shown="True" w1316 {
                tunnel: w1315 -> [_ w1322]
                tunnel: w1314 -> [w1319 w1321]
                tunnel: [w1319 w1320] -> w1313
                frame False {
                }
                frame True {
                  n507 = Build Array (concatenate)(w1321, w1322) -> (w1320:T3)
                }
              }
            }
          }
        }
        n508 = Index Array(array=w1265, index=w1279) -> (element=w1283:T12)
        n509 = flat-sequence {
          tunnel: w1268 -> [w1296]
          tunnel: [w1297] -> w1264
          frame #0 {
            n510 = property on="AO_Select Channel1" class="Ring (strict)"("Strings []"=w1296) -> ()  [unwired: 2 in, 2 out]
          }
          frame #1 {
            n511 = property on="AO_Select Channel1" class="Ring (strict)"() -> ("RingText.Text"=w1297:string)  [unwired: 2 in, 2 out]
          }
        }
        n512 = Unbundle By Name(w1283) -> ("Name"=w1282:string, "Channel Names"=w1268:string[])
        n513 = call "CRYGet Freq Bit Array.vi"("Device Infor"=w1283) -> ("MaxFreq"=w1280:u32, "MinFreq"=w1281:u32, "Bit Depth"=w1292:cluster{"String":string, "Value":ext}[], "Samplein Rate"=w1276:cluster{"String":string, "Value":ext}[])  [unwired: 1 in, 6 out]
        n514 = property on="AO_Sampling Rate" class="Ring (strict)"("StringsAndValues[]"=w1276) -> ()  [unwired: 2 in, 2 out]
        n515 = property on="AO_Bit Depth" class="Ring (strict)"("StringsAndValues[]"=w1292) -> ()  [unwired: 2 in, 2 out]
        n516 = property on="AO_Sampling User" class="DigNum (strict)"("Minimum"=w1281) -> ()  [unwired: 2 in, 2 out]
        n517 = property on="AO_Sampling User" class="DigNum (strict)"("Maximum"=w1280) -> ()  [unwired: 2 in, 2 out]
        n518 = Index Array(array=w1292, index=0) -> (element=w1294:cluster{"String":string, "Value":ext})
        n519 = Unbundle By Name(w1294) -> ()  [unwired: 1 out]
        n520 = property on="AO_Bit Depth" class="Ring (strict)"() -> ("Value"=w1278:u16)  [unwired: 2 in, 2 out]
        n521 = property on="AO_Device Name" class="Ring (strict)"() -> ("Value"=w1258:u16)  [unwired: 2 in, 2 out]
        n522 = property on="AI_Device Name" class="Ring (strict)"() -> ("Value"=w1254:u16)  [unwired: 2 in, 2 out]
        n523 = property on="AO_Device Name" class="Ring (strict)"() -> ("Disabled Items []"=w1257:i32[])  [unwired: 2 in, 2 out]
        n524 = property on="AI_Device Name" class="Ring (strict)"() -> ("Disabled Items []"=w1252:i32[])  [unwired: 2 in, 2 out]
        n525 = local read "O_Channel Info"() -> (w1291:T2[])
        n526 = property on="AO_SoundCard Channel" class="Ring (strict)"() -> ("Value"=w1290:u16)  [unwired: 2 in, 2 out]
        n527 = Search 1D Array(1D array=w1252, element=w1254) -> (index of element=w1253:i32)  [unwired: 1 in]
        n528 = for {
          tunnel: w1276 -> [w1324] mode=indexing
          tunnel: [w1323] -> w1277 mode=indexing
          n529 = Unbundle By Name(w1324) -> ("Value"=w1323:ext)
        }
        n530 = Less Than 0?(x=w1253) -> (x < 0?=w1255:bool)
        n531 = property on="AO_Sampling Rate" class="Ring (strict)"() -> ("Value"=w1275:u32)  [unwired: 2 in, 2 out]
        n532 = Index Array(array=w1291, index=w1290) -> (element=w1289:T2)
        n533 = Search 1D Array(1D array=w1277, element=w1275) -> (index of element=w1273:i32)  [unwired: 1 out]
        n534 = Search 1D Array(1D array=w1257, element=w1258) -> (index of element=w1251:i32)  [unwired: 1 in]
        n535 = Not Equal To 0?(x=w1273) -> (x != 0?=w1274:bool)
        n536 = local read "I_Channel Info"() -> (w1286:T2[])
        n537 = Less Than 0?(x=w1251) -> (x < 0?=w1262:bool)
        n538 = Select(t=w1273, s=w1274, f=0) -> (s? t:f=w1271:i32)
        n539 = Index Array(array=w1276, index=w1271) -> (element=w1293:cluster{"String":string, "Value":ext})
        n540 = Unbundle By Name(w1293) -> ("Value"=w1287:ext)
        n541 = Bundle By Name(cluster=w1289, "ID"=w1279, "Sampling Rate (Hz)"=w1287, "Bit Depth"=w1278, "Device Name"=w1282, "ASIOChannel Name"=w1264) -> (w1288:T2)
        n542 = Replace Array Subset(array=w1291, new element=w1288, index=w1290) -> (w1284:T2[])
        n543 = local write "O_Channel Info"(w1284) -> ()
        n544 = And(x=w1255, y=w1262) -> (x .and. y?=w1260:bool)
        n545 = property on="AO_Sampling Rate" class="Ring (strict)"("Val(Sgnl)"=w1287) -> ()  [unwired: 2 in, 2 out]
        n546 = Select(t=T7."Enabled" ("Disabled"), s=w1260, f=T7."Disabled and Grayed Out" ("Disabled")) -> (s? t:f=w1263:T7)
        n547 = Select(t=T7."Enabled" ("Disabled"), s=w1262, f=T7."Disabled and Grayed Out" ("Disabled")) -> (s? t:f=w1259:T7)
        n548 = Insert Into Array(array=w1284, new element=w1286) -> (w1285:T2[])  [unwired: 1 in]
        n549 = property on="AO_Launch" class="Bool (strict)"("DisabledEnum"=w1259) -> ()  [unwired: 2 in, 2 out]
        n550 = property on="AO_Sampling Rate" class="Ring (strict)"("DisabledEnum"=w1259) -> ()  [unwired: 2 in, 2 out]
        n551 = property on="AO_Alias freq" class="DigNum (strict)"("DisabledEnum"=w1259) -> ()  [unwired: 2 in, 2 out]
        n552 = property on="Calibrartion" class="Bool (strict)"("DisabledEnum"=w1263) -> ()  [unwired: 2 in, 2 out]
        n553 = local read "SoundCard"() -> (w1270:T5)
        n554 = Bundle By Name(cluster=w1270, "Channel Array"=w1285) -> (w1269:T5)
        n555 = property on="Calibration Seq" class="Ring (strict)"("DisabledEnum"=w1263) -> ()  [unwired: 2 in, 2 out]
        n556 = property on="AO_Select SMode" class="RadioBtnsControl (strict)"("DisabledEnum"=w1259) -> ()  [unwired: 2 in, 2 out]
        n557 = property on="AO_Sampling User" class="DigNum (strict)"("DisabledEnum"=w1259) -> ()  [unwired: 2 in, 2 out]
        n558 = property on="AO_Vp" class="DigNum (strict)"("DisabledEnum"=w1259) -> ()  [unwired: 2 in, 2 out]
        n559 = local write "SoundCard"(w1269) -> ()
        n560 = property on="AO_Select Channel1" class="Ring (strict)"("DisabledEnum"=w1259) -> ()  [unwired: 2 in, 2 out]
        n561 = property on="AO_Bit Depth" class="Ring (strict)"("DisabledEnum"=w1259) -> ()  [unwired: 2 in, 2 out]
      }
      event "AI_Device Name": Value Change {
        n562 = event-data() -> ("NewVal"=w1356:u16)  [unwired: 6 out]
        n563 = local read "I_Device Info"() -> (w1344:T3)
        n564 = for {
          tunnel: w1344 -> [w1376] mode=indexing
          shift-right: [w1374] -> w1343
          shift-left: T3 [] ("O_Device Info") -> [w1375]
          n565 = local read "AI_Audio Driver"() -> (w1378:enum32{"Radio Selection 1", "Radio Selection 2"})
          n566 = Unbundle By Name(w1376) -> ("Driver Type"=w1377:string)
          n567 = case shown="\"Radio Selection 1\", Default" w1378 {
            tunnel: w1377 -> [w1384 w1394]
            tunnel: w1376 -> [w1381 w1391]
            tunnel: w1375 -> [w1380 w1390]
            tunnel: [w1379 w1389] -> w1374
            frame "Radio Selection 1", Default {
              n568 = Equal?(x=w1384, y="MME") -> (x = y?=w1382:bool)
              n569 = case shown="True" w1382 {
                tunnel: w1381 -> [_ w1388]
                tunnel: w1380 -> [w1385 w1387]
                tunnel: [w1385 w1386] -> w1379
                frame False {
                }
                frame True {
                  n570 = Build Array (concatenate)(w1387, w1388) -> (w1386:T3)
                }
              }
            }
            frame "Radio Selection 2" {
              n571 = Equal?(x=w1394, y="ASIO") -> (x = y?=w1392:bool)
              n572 = case shown="True" w1392 {
                tunnel: w1391 -> [_ w1398]
                tunnel: w1390 -> [w1395 w1397]
                tunnel: [w1395 w1396] -> w1389
                frame False {
                }
                frame True {
                  n573 = Build Array (concatenate)(w1397, w1398) -> (w1396:T3)
                }
              }
            }
          }
        }
        n574 = Index Array(array=w1343, index=w1356) -> (element=w1360:T12)
        n575 = call "CRYGet Freq Bit Array.vi"("Device Infor"=w1360) -> ("MaxFreq"=w1357:u32, "MinFreq"=w1358:u32, "Bit Depth"=w1368:cluster{"String":string, "Value":ext}[], "Samplein Rate"=w1354:cluster{"String":string, "Value":ext}[])  [unwired: 1 in, 6 out]
        n576 = Unbundle By Name(w1360) -> ("Name"=w1359:string, "Channel Names"=w1342:string[])
        n577 = property on="AI_Bit Depth" class="Ring (strict)"("StringsAndValues[]"=w1368) -> ()  [unwired: 2 in, 2 out]
        n578 = property on="AI_Sampling Rate" class="Ring (strict)"("StringsAndValues[]"=w1354) -> ()  [unwired: 2 in, 2 out]
        n579 = flat-sequence {
          tunnel: w1342 -> [w1372]
          tunnel: [w1373] -> w1340
          frame #0 {
            n580 = property on="AI_Select Channel1" class="Ring (strict)"("Strings []"=w1372) -> ()  [unwired: 2 in, 2 out]
          }
          frame #1 {
            n581 = property on="AI_Select Channel1" class="Ring (strict)"() -> ("RingText.Text"=w1373:string)  [unwired: 2 in, 2 out]
          }
        }
        n582 = property on="AI_Sampling User" class="DigNum (strict)"("Minimum"=w1358) -> ()  [unwired: 2 in, 2 out]
        n583 = property on="AI_Sampling User" class="DigNum (strict)"("Maximum"=w1357) -> ()  [unwired: 2 in, 2 out]
        n584 = Index Array(array=w1368, index=0) -> (element=w1370:cluster{"String":string, "Value":ext})
        n585 = Unbundle By Name(w1370) -> ()  [unwired: 1 out]
        n586 = property on="AI_Bit Depth" class="Ring (strict)"() -> ("Value"=w1355:u16)  [unwired: 2 in, 2 out]
        n587 = local read "I_Channel Info"() -> (w1367:T2[])
        n588 = for {
          tunnel: w1354 -> [w1400] mode=indexing
          tunnel: [w1399] -> w1353 mode=indexing
          n589 = Unbundle By Name(w1400) -> ("Value"=w1399:ext)
        }
        n590 = property on="AI_SoundCard Channel" class="Ring (strict)"() -> ("Value"=w1366:u16)  [unwired: 2 in, 2 out]
        n591 = property on="AI_Sampling Rate" class="Ring (strict)"() -> ("Value"=w1352:u32)  [unwired: 2 in, 2 out]
        n592 = Search 1D Array(1D array=w1353, element=w1352) -> (index of element=w1350:i32)  [unwired: 1 out]
        n593 = property on="AO_Device Name" class="Ring (strict)"() -> ("Value"=w1325:u16)  [unwired: 2 in, 2 out]
        n594 = property on="AI_Device Name" class="Ring (strict)"() -> ("Value"=w1334:u16)  [unwired: 2 in, 2 out]
        n595 = property on="AO_Device Name" class="Ring (strict)"() -> ("Disabled Items []"=w1326:i32[])  [unwired: 2 in, 2 out]
        n596 = property on="AI_Device Name" class="Ring (strict)"() -> ("Disabled Items []"=w1333:i32[])  [unwired: 2 in, 2 out]
        n597 = Not Equal To 0?(x=w1350) -> (x != 0?=w1351:bool)
        n598 = Index Array(array=w1367, index=w1366) -> (element=w1365:T2)
        n599 = Select(t=w1350, s=w1351, f=0) -> (s? t:f=w1348:i32)
        n600 = Index Array(array=w1354, index=w1348) -> (element=w1369:cluster{"String":string, "Value":ext})
        n601 = Unbundle By Name(w1369) -> ("Value"=w1347:ext)
        n602 = Bundle By Name(cluster=w1365, "ID"=w1356, "Sampling Rate (Hz)"=w1347, "Bit Depth"=w1355, "Device Name"=w1359, "ASIOChannel Name"=w1340) -> (w1364:T2)
        n603 = property on="AI_Sampling Rate" class="Ring (strict)"("Val(Sgnl)"=w1347) -> ()  [unwired: 2 in, 2 out]
        n604 = Replace Array Subset(array=w1367, new element=w1364, index=w1366) -> (w1361:T2[])
        n605 = Search 1D Array(1D array=w1326, element=w1325) -> (index of element=w1327:i32)  [unwired: 1 in]
        n606 = local write "I_Channel Info"(w1361) -> ()
        n607 = local read "O_Channel Info"() -> (w1362:T2[])
        n608 = Less Than 0?(x=w1327) -> (x < 0?=w1331:bool)
        n609 = local read "SoundCard"() -> (w1346:T5)
        n610 = Search 1D Array(1D array=w1333, element=w1334) -> (index of element=w1328:i32)  [unwired: 1 in]
        n611 = Insert Into Array(array=w1362, new element=w1361) -> (w1363:T2[])  [unwired: 1 in]
        n612 = Bundle By Name(cluster=w1346, "Channel Array"=w1363) -> (w1345:T5)
        n613 = Less Than 0?(x=w1328) -> (x < 0?=w1339:bool)
        n614 = And(x=w1331, y=w1339) -> (x .and. y?=w1338:bool)
        n615 = Select(t=T7."Enabled" ("Disabled"), s=w1339, f=T7."Disabled and Grayed Out" ("Disabled")) -> (s? t:f=w1332:T7)
        n616 = Select(t=T7."Enabled" ("Disabled"), s=w1338, f=T7."Disabled and Grayed Out" ("Disabled")) -> (s? t:f=w1337:T7)
        n617 = local write "SoundCard"(w1345) -> ()
        n618 = property on="AI_Launch" class="Bool (strict)"("DisabledEnum"=w1332) -> ()  [unwired: 2 in, 2 out]
        n619 = property on="AI_Latency" class="DigNum (strict)"("DisabledEnum"=w1332) -> ()  [unwired: 2 in, 2 out]
        n620 = property on="AI_Sampling Rate" class="Ring (strict)"("DisabledEnum"=w1332) -> ()  [unwired: 2 in, 2 out]
        n621 = property on="AI_Alias freq" class="DigNum (strict)"("DisabledEnum"=w1332) -> ()  [unwired: 2 in, 2 out]
        n622 = property on="Calibrartion" class="Bool (strict)"("DisabledEnum"=w1337) -> ()  [unwired: 2 in, 2 out]
        n623 = property on="Calibration Seq" class="Ring (strict)"("DisabledEnum"=w1337) -> ()  [unwired: 2 in, 2 out]
        n624 = property on="AI_Select Channel1" class="Ring (strict)"("DisabledEnum"=w1332) -> ()  [unwired: 2 in, 2 out]
        n625 = property on="AI_Select SMode" class="RadioBtnsControl (strict)"("DisabledEnum"=w1332) -> ()  [unwired: 2 in, 2 out]
        n626 = property on="AI_Sampling User" class="DigNum (strict)"("DisabledEnum"=w1332) -> ()  [unwired: 2 in, 2 out]
        n627 = property on="AI_Vp" class="DigNum (strict)"("DisabledEnum"=w1332) -> ()  [unwired: 2 in, 2 out]
        n628 = property on="AI_Bit Depth" class="Ring (strict)"("DisabledEnum"=w1332) -> ()  [unwired: 2 in, 2 out]
      }
      event "AI_Latency": Value Change {
        n629 = event-data() -> ("NewVal"=w1403:u32)  [unwired: 6 out]
        n630 = local read "I_Channel Info"() -> (w1408:T2[])
        n631 = property on="AI_SoundCard Channel" class="Ring (strict)"() -> ("Value"=w1407:u16)  [unwired: 2 in, 2 out]
        n632 = Index Array(array=w1408, index=w1407) -> (element=w1410:T2)
        n633 = Bundle By Name(cluster=w1410, "Latency (samples)"=w1403) -> (w1409:T2)
        n634 = Replace Array Subset(array=w1408, new element=w1409, index=w1407) -> (w1404:T2[])
        n635 = local write "I_Channel Info"(w1404) -> ()
        n636 = local read "O_Channel Info"() -> (w1406:T2[])
        n637 = local read "SoundCard"() -> (w1402:T5)
        n638 = Insert Into Array(array=w1406, new element=w1404) -> (w1405:T2[])  [unwired: 1 in]
        n639 = Bundle By Name(cluster=w1402, "Channel Array"=w1405) -> (w1401:T5)
        n640 = local write "SoundCard"(w1401) -> ()
      }
      event "AO_Sampling Rate": Value Change {
        n641 = event-data() -> ("OldVal"=w1426:u32, "NewVal"=w1425:u32)  [unwired: 5 out]
        n642 = Equal?(x=w1425, y=u32 0) -> (x = y?=w1427:bool)
        n643 = Select(t=w1426, s=w1427, f=w1425) -> (s? t:f=w1422:u32)
        n644 = property on="AO_Sampling User" class="DigNum (strict)"("Visible"=w1427) -> ()  [unwired: 2 in, 2 out]
        n645 = property on="AO_Sampling User" class="DigNum (strict)"("Value"=w1426) -> ()  [unwired: 2 in, 2 out]
        n646 = Divide(x=w1422, y=2.0) -> (x/y=w1421:dbl)
        n647 = Divide(x=w1422, y=2.10526) -> (x/y=w1420:dbl)
        n648 = property on="AO_Alias freq" class="DigNum (strict)"("Maximum"=w1421) -> ()  [unwired: 2 in, 2 out]
        n649 = local read "O_Channel Info"() -> (w1419:T2[])
        n650 = property on="AO_SoundCard Channel" class="Ring (strict)"() -> ("Value"=w1418:u16)  [unwired: 2 in, 2 out]
        n651 = property on="AO_Alias freq" class="DigNum (strict)"("Value"=w1420) -> ()  [unwired: 2 in, 2 out]
        n652 = Index Array(array=w1419, index=w1418) -> (element=w1417:T2)
        n653 = Bundle By Name(cluster=w1417, "Sampling Rate (Hz)"=w1422, "Anti-aliasing Factor (%fs)"=w1420) -> (w1416:T2)
        n654 = Replace Array Subset(array=w1419, new element=w1416, index=w1418) -> (w1412:T2[])
        n655 = local read "I_Channel Info"() -> (w1415:T2[])
        n656 = local read "SoundCard"() -> (w1414:T5)
        n657 = local write "O_Channel Info"(w1412) -> ()
        n658 = Insert Into Array(array=w1412, new element=w1415) -> (w1413:T2[])  [unwired: 1 in]
        n659 = Bundle By Name(cluster=w1414, "Channel Array"=w1413) -> (w1411:T5)
        n660 = local write "SoundCard"(w1411) -> ()
      }
      event "AI_Sampling Rate": Value Change {
        n661 = event-data() -> ("OldVal"=w1444:u32, "NewVal"=w1443:u32)  [unwired: 5 out]
        n662 = Equal?(x=w1443, y=u32 0) -> (x = y?=w1445:bool)
        n663 = Select(t=w1444, s=w1445, f=w1443) -> (s? t:f=w1441:u32)
        n664 = property on="AI_Sampling User" class="DigNum (strict)"("Visible"=w1445) -> ()  [unwired: 2 in, 2 out]
        n665 = property on="AI_Sampling User" class="DigNum (strict)"("Value"=w1444) -> ()  [unwired: 2 in, 2 out]
        n666 = Divide(x=w1441, y=2.0) -> (x/y=w1439:dbl)
        n667 = Divide(x=w1441, y=2.10526) -> (x/y=w1438:dbl)
        n668 = property on="AI_Alias freq" class="DigNum (strict)"("Maximum"=w1439) -> ()  [unwired: 2 in, 2 out]
        n669 = property on="AI_Alias freq" class="DigNum (strict)"("Value"=w1438) -> ()  [unwired: 2 in, 2 out]
        n670 = local read "I_Channel Info"() -> (w1437:T2[])
        n671 = property on="AI_SoundCard Channel" class="Ring (strict)"() -> ("Value"=w1436:u16)  [unwired: 2 in, 2 out]
        n672 = Index Array(array=w1437, index=w1436) -> (element=w1435:T2)
        n673 = Bundle By Name(cluster=w1435, "Sampling Rate (Hz)"=w1441, "Anti-aliasing Factor (%fs)"=w1438) -> (w1434:T2)
        n674 = Replace Array Subset(array=w1437, new element=w1434, index=w1436) -> (w1430:T2[])
        n675 = local write "I_Channel Info"(w1430) -> ()
        n676 = local read "O_Channel Info"() -> (w1433:T2[])
        n677 = local read "SoundCard"() -> (w1432:T5)
        n678 = Insert Into Array(array=w1433, new element=w1430) -> (w1431:T2[])  [unwired: 1 in]
        n679 = Bundle By Name(cluster=w1432, "Channel Array"=w1431) -> (w1429:T5)
        n680 = local write "SoundCard"(w1429) -> ()
      }
      event "AO_Bit Depth": Value Change {
        n681 = event-data() -> ("NewVal"=w1452:u16)  [unwired: 1 out]
        n682 = local read "O_Channel Info"() -> (w1456:T2[])
        n683 = property on="AO_SoundCard Channel" class="Ring (strict)"() -> ("Value"=w1455:u16)  [unwired: 2 in, 2 out]
        n684 = Index Array(array=w1456, index=w1455) -> (element=w1454:T2)
        n685 = Bundle By Name(cluster=w1454, "Bit Depth"=w1452) -> (w1453:T2)
        n686 = local read "I_Channel Info"() -> (w1449:T2[])
        n687 = local read "SoundCard"() -> (w1450:T5)
        n688 = Replace Array Subset(array=w1456, new element=w1453, index=w1455) -> (w1448:T2[])
        n689 = local write "O_Channel Info"(w1448) -> ()
        n690 = Insert Into Array(array=w1448, new element=w1449) -> (w1451:T2[])  [unwired: 1 in]
        n691 = Bundle By Name(cluster=w1450, "Channel Array"=w1451) -> (w1447:T5)
        n692 = local write "SoundCard"(w1447) -> ()
      }
      event "AI_Bit Depth": Value Change {
        n693 = event-data() -> ("NewVal"=w1462:u16)  [unwired: 1 out]
        n694 = local read "I_Channel Info"() -> (w1466:T2[])
        n695 = property on="AI_SoundCard Channel" class="Ring (strict)"() -> ("Value"=w1465:u16)  [unwired: 2 in, 2 out]
        n696 = Index Array(array=w1466, index=w1465) -> (element=w1464:T2)
        n697 = Bundle By Name(cluster=w1464, "Bit Depth"=w1462) -> (w1463:T2)
        n698 = Replace Array Subset(array=w1466, new element=w1463, index=w1465) -> (w1458:T2[])
        n699 = local write "I_Channel Info"(w1458) -> ()
        n700 = local read "O_Channel Info"() -> (w1461:T2[])
        n701 = local read "SoundCard"() -> (w1460:T5)
        n702 = Insert Into Array(array=w1461, new element=w1458) -> (w1459:T2[])  [unwired: 1 in]
        n703 = Bundle By Name(cluster=w1460, "Channel Array"=w1459) -> (w1457:T5)
        n704 = local write "SoundCard"(w1457) -> ()
      }
      event "AO_Sampling User": Value Change {
        n705 = event-data() -> ("NewVal"=w1468:u32)  [unwired: 1 out]
        n706 = Divide(x=w1468, y=2.0) -> (x/y=w1473:dbl)
        n707 = local read "O_Channel Info"() -> (w1477:T2[])
        n708 = property on="AO_SoundCard Channel" class="Ring (strict)"() -> ("Value"=w1476:u16)  [unwired: 2 in, 2 out]
        n709 = property on="AO_Alias freq" class="DigNum (strict)"("Maximum"=w1473) -> ()  [unwired: 2 in, 2 out]
        n710 = property on="AO_Alias freq" class="DigNum (strict)"("Value"=w1473) -> ()  [unwired: 2 in, 2 out]
        n711 = Index Array(array=w1477, index=w1476) -> (element=w1475:T2)
        n712 = Bundle By Name(cluster=w1475, "Sampling Rate (Hz)"=w1468, "Anti-aliasing Factor (%fs)"=w1473) -> (w1474:T2)
        n713 = local read "I_Channel Info"() -> (w1470:T2[])
        n714 = Replace Array Subset(array=w1477, new element=w1474, index=w1476) -> (w1469:T2[])
        n715 = local read "SoundCard"() -> (w1471:T5)
        n716 = local write "O_Channel Info"(w1469) -> ()
        n717 = Insert Into Array(array=w1469, new element=w1470) -> (w1472:T2[])  [unwired: 1 in]
        n718 = Bundle By Name(cluster=w1471, "Channel Array"=w1472) -> (w1467:T5)
        n719 = local write "SoundCard"(w1467) -> ()
      }
      event "AI_Sampling User": Value Change {
        n720 = event-data() -> ("NewVal"=w1480:u32)  [unwired: 1 out]
        n721 = local read "I_Channel Info"() -> (w1489:T2[])
        n722 = Divide(x=w1480, y=2.0) -> (x/y=w1485:dbl)
        n723 = property on="AI_SoundCard Channel" class="Ring (strict)"() -> ("Value"=w1488:u16)  [unwired: 2 in, 2 out]
        n724 = property on="AI_Alias freq" class="DigNum (strict)"("Maximum"=w1485) -> ()  [unwired: 2 in, 2 out]
        n725 = property on="AI_Alias freq" class="DigNum (strict)"("Value"=w1485) -> ()  [unwired: 2 in, 2 out]
        n726 = Index Array(array=w1489, index=w1488) -> (element=w1487:T2)
        n727 = Bundle By Name(cluster=w1487, "Sampling Rate (Hz)"=w1480, "Anti-aliasing Factor (%fs)"=w1485) -> (w1486:T2)
        n728 = local read "O_Channel Info"() -> (w1484:T2[])
        n729 = Replace Array Subset(array=w1489, new element=w1486, index=w1488) -> (w1481:T2[])
        n730 = local read "SoundCard"() -> (w1483:T5)
        n731 = local write "I_Channel Info"(w1481) -> ()
        n732 = Insert Into Array(array=w1484, new element=w1481) -> (w1482:T2[])  [unwired: 1 in]
        n733 = Bundle By Name(cluster=w1483, "Channel Array"=w1482) -> (w1479:T5)
        n734 = local write "SoundCard"(w1479) -> ()
      }
      event "AO_Alias freq": Value Change {
        n735 = event-data() -> ("NewVal"=w1500:u32)  [unwired: 1 out]
        n736 = local read "O_Channel Info"() -> (w1499:T2[])
        n737 = property on="AO_SoundCard Channel" class="Ring (strict)"() -> ("Value"=w1498:u16)  [unwired: 2 in, 2 out]
        n738 = Index Array(array=w1499, index=w1498) -> (element=w1496:T2)
        n739 = Bundle By Name(cluster=w1496, "Anti-aliasing Factor (%fs)"=w1500) -> (w1497:T2)
        n740 = Replace Array Subset(array=w1499, new element=w1497, index=w1498) -> (w1492:T2[])
        n741 = local read "I_Channel Info"() -> (w1493:T2[])
        n742 = local read "SoundCard"() -> (w1494:T5)
        n743 = local write "O_Channel Info"(w1492) -> ()
        n744 = Insert Into Array(array=w1492, new element=w1493) -> (w1495:T2[])  [unwired: 1 in]
        n745 = Bundle By Name(cluster=w1494, "Channel Array"=w1495) -> (w1491:T5)
        n746 = local write "SoundCard"(w1491) -> ()
      }
      event "AI_Alias freq": Value Change {
        n747 = event-data() -> ("NewVal"=w1503:u32)  [unwired: 1 out]
        n748 = local read "I_Channel Info"() -> (w1509:T2[])
        n749 = To Single Precision Float(number=w1503) -> (single precision float=w1502:sgl)
        n750 = property on="AI_SoundCard Channel" class="Ring (strict)"() -> ("Value"=w1508:u16)  [unwired: 2 in, 2 out]
        n751 = Index Array(array=w1509, index=w1508) -> (element=w1510:T2)
        n752 = Bundle By Name(cluster=w1510, "Anti-aliasing Factor (%fs)"=w1502) -> (w1511:T2)
        n753 = Replace Array Subset(array=w1509, new element=w1511, index=w1508) -> (w1504:T2[])
        n754 = local write "I_Channel Info"(w1504) -> ()
        n755 = local read "O_Channel Info"() -> (w1507:T2[])
        n756 = local read "SoundCard"() -> (w1506:T5)
        n757 = Insert Into Array(array=w1507, new element=w1504) -> (w1505:T2[])  [unwired: 1 in]
        n758 = Bundle By Name(cluster=w1506, "Channel Array"=w1505) -> (w1501:T5)
        n759 = local write "SoundCard"(w1501) -> ()
      }
      event "AO_Select Channel1": Value Change {
        n760 = event-data() -> ("NewVal"=w1519:u16, "CtlRef"=w1513:refnum<vi>)  [unwired: 1 out]
        n761 = property class="Ring (strict)"(reference=w1513) -> ("RingText.Text"=w1512:string)  [unwired: 1 in, 2 out]
        n762 = local read "O_Channel Info"() -> (w1523:T2[])
        n763 = property on="AO_SoundCard Channel" class="Ring (strict)"() -> ("Value"=w1522:u16)  [unwired: 2 in, 2 out]
        n764 = Index Array(array=w1523, index=w1522) -> (element=w1520:T2)
        n765 = Bundle By Name(cluster=w1520, "Hardware Ch ID"=w1519, "ASIOChannel Name"=w1512) -> (w1521:T2)
        n766 = Replace Array Subset(array=w1523, new element=w1521, index=w1522) -> (w1515:T2[])
        n767 = local read "I_Channel Info"() -> (w1516:T2[])
        n768 = local write "O_Channel Info"(w1515) -> ()
        n769 = local read "SoundCard"() -> (w1517:T5)
        n770 = Insert Into Array(array=w1515, new element=w1516) -> (w1518:T2[])  [unwired: 1 in]
        n771 = Bundle By Name(cluster=w1517, "Channel Array"=w1518) -> (w1514:T5)
        n772 = local write "SoundCard"(w1514) -> ()
      }
      event "AI_Select Channel1": Value Change {
        n773 = event-data() -> ("NewVal"=w1533:u16, "CtlRef"=w1525:refnum<vi>)  [unwired: 1 out]
        n774 = property class="Ring (strict)"(reference=w1525) -> ("RingText.Text"=w1524:string)  [unwired: 1 in, 2 out]
        n775 = local read "I_Channel Info"() -> (w1532:T2[])
        n776 = property on="AI_SoundCard Channel" class="Ring (strict)"() -> ("Value"=w1531:u16)  [unwired: 2 in, 2 out]
        n777 = Index Array(array=w1532, index=w1531) -> (element=w1534:T2)
        n778 = Bundle By Name(cluster=w1534, "Hardware Ch ID"=w1533, "ASIOChannel Name"=w1524) -> (w1535:T2)
        n779 = Replace Array Subset(array=w1532, new element=w1535, index=w1531) -> (w1527:T2[])
        n780 = local write "I_Channel Info"(w1527) -> ()
        n781 = local read "O_Channel Info"() -> (w1530:T2[])
        n782 = local read "SoundCard"() -> (w1529:T5)
        n783 = Insert Into Array(array=w1530, new element=w1527) -> (w1528:T2[])  [unwired: 1 in]
        n784 = Bundle By Name(cluster=w1529, "Channel Array"=w1528) -> (w1526:T5)
        n785 = local write "SoundCard"(w1526) -> ()
      }
      event "AO_Select SMode": Value Change {
        n786 = event-data() -> ("NewVal"=w1545:enum32{"Analog", "Digital"})  [unwired: 1 out]
        n787 = property on="Advanced View" class="Bool (strict)"() -> ("Value"=w1539:bool)  [unwired: 2 in, 2 out]
        n788 = Equal?(x=w1545, y=enum32{"Analog", "Digital"}."Digital" ("AO_Select Channel2")) -> (x = y?=w1537:bool)
        n789 = case shown="True" w1539 {
          tunnel: w1537 -> [_ w1554]
          frame False {
            w1552 = FALSE ("Visible")
            n790 = property on="AO_Vp" class="DigNum (strict)"("Visible"=w1552) -> ()  [unwired: 2 in, 2 out]
            n791 = property on="AO_%FSD" class="DigNum (strict)"("Visible"=w1552) -> ()  [unwired: 2 in, 2 out]
          }
          frame True {
            n792 = Not(x=w1554) -> (.not. x?=w1553:bool)
            n793 = property on="AO_Vp" class="DigNum (strict)"("Visible"=w1553) -> ()  [unwired: 2 in, 2 out]
            n794 = property on="AO_%FSD" class="DigNum (strict)"("Visible"=w1554) -> ()  [unwired: 2 in, 2 out]
          }
        }
        n795 = case shown="False" w1537 {
          tunnel: [w1550 w1551] -> w1536
          frame False {
            n796 = local read "AO_Vp"() -> (w1550:dbl)
          }
          frame True {
            w1551 = 1.0 ("AO_Vp")
            n797 = local write "AO_Vp"(w1551) -> ()
          }
        }
        n798 = property on="AO_SoundCard Channel" class="Ring (strict)"() -> ("Value"=w1548:u16)  [unwired: 2 in, 2 out]
        n799 = local read "O_Channel Info"() -> (w1549:T2[])
        n800 = Index Array(array=w1549, index=w1548) -> (element=w1546:T2)
        n801 = Bundle By Name(cluster=w1546, "Digital"=w1537, "Vmax (V)"=w1536) -> (w1547:T2)
        n802 = local read "I_Channel Info"() -> (w1541:T2[])
        n803 = Replace Array Subset(array=w1549, new element=w1547, index=w1548) -> (w1540:T2[])
        n804 = local write "O_Channel Info"(w1540) -> ()
        n805 = Insert Into Array(array=w1540, new element=w1541) -> (w1543:T2[])  [unwired: 1 in]
        n806 = local read "SoundCard"() -> (w1542:T5)
        n807 = Bundle By Name(cluster=w1542, "Channel Array"=w1543) -> (w1538:T5)
        n808 = local write "SoundCard"(w1538) -> ()
      }
      event "AI_Select SMode": Value Change {
        n809 = event-data() -> ("NewVal"=w1565:enum32{"Analog", "Digital"})  [unwired: 1 out]
        n810 = property on="Advanced View" class="Bool (strict)"() -> ("Value"=w1558:bool)  [unwired: 2 in, 2 out]
        n811 = Equal?(x=w1565, y=enum32{"Analog", "Digital"}."Digital" ("AO_Select Channel2")) -> (x = y?=w1556:bool)
        n812 = case shown="False" w1558 {
          tunnel: w1556 -> [_ w1572]
          frame False {
            w1571 = FALSE ("Visible")
            n813 = property on="AI_Vp" class="DigNum (strict)"("Visible"=w1571) -> ()  [unwired: 2 in, 2 out]
            n814 = property on="AI_%FSD" class="DigNum (strict)"("Visible"=w1571) -> ()  [unwired: 2 in, 2 out]
          }
          frame True {
            n815 = Not(x=w1572) -> (.not. x?=w1573:bool)
            n816 = property on="AI_Vp" class="DigNum (strict)"("Visible"=w1573) -> ()  [unwired: 2 in, 2 out]
            n817 = property on="AI_%FSD" class="DigNum (strict)"("Visible"=w1572) -> ()  [unwired: 2 in, 2 out]
          }
        }
        n818 = case shown="False" w1556 {
          tunnel: [w1569 w1570] -> w1555
          frame False {
            n819 = local read "AI_Vp"() -> (w1569:dbl)
          }
          frame True {
            w1570 = 1.0 ("AI_Vp")
            n820 = local write "AI_Vp"(w1570) -> ()
          }
        }
        n821 = local read "I_Channel Info"() -> (w1563:T2[])
        n822 = property on="AI_SoundCard Channel" class="Ring (strict)"() -> ("Value"=w1564:u16)  [unwired: 2 in, 2 out]
        n823 = Index Array(array=w1563, index=w1564) -> (element=w1567:T2)
        n824 = Bundle By Name(cluster=w1567, "Digital"=w1556, "Vmax (V)"=w1555) -> (w1568:T2)
        n825 = Replace Array Subset(array=w1563, new element=w1568, index=w1564) -> (w1559:T2[])
        n826 = local write "I_Channel Info"(w1559) -> ()
        n827 = local read "O_Channel Info"() -> (w1562:T2[])
        n828 = Insert Into Array(array=w1562, new element=w1559) -> (w1560:T2[])  [unwired: 1 in]
        n829 = local read "SoundCard"() -> (w1561:T5)
        n830 = Bundle By Name(cluster=w1561, "Channel Array"=w1560) -> (w1557:T5)
        n831 = local write "SoundCard"(w1557) -> ()
      }
      event "AO_Vp": Value Change {
        w1576 = 0.01 ("y")
        n832 = event-data() -> ("NewVal"=w1577:dbl)  [unwired: 1 out]
        n833 = Greater?(x=w1577, y=w1576) -> (0:w1578:bool)
        n834 = local read "O_Channel Info"() -> (w1586:T2[])
        n835 = property on="AO_SoundCard Channel" class="Ring (strict)"() -> ("Value"=w1585:u16)  [unwired: 2 in, 2 out]
        n836 = Select(t=w1577, s=w1578, f=w1576) -> (s? t:f=w1575:dbl)
        n837 = property on="AO_Vp" class="DigNum (strict)"("Value"=w1575) -> ()  [unwired: 2 in, 2 out]
        n838 = Index Array(array=w1586, index=w1585) -> (element=w1584:T2)
        n839 = Bundle By Name(cluster=w1584, "Vmax (V)"=w1575) -> (w1583:T2)
        n840 = local read "I_Channel Info"() -> (w1580:T2[])
        n841 = Replace Array Subset(array=w1586, new element=w1583, index=w1585) -> (w1579:T2[])
        n842 = local read "SoundCard"() -> (w1581:T5)
        n843 = local write "O_Channel Info"(w1579) -> ()
        n844 = Insert Into Array(array=w1579, new element=w1580) -> (w1582:T2[])  [unwired: 1 in]
        n845 = Bundle By Name(cluster=w1581, "Channel Array"=w1582) -> (w1574:T5)
        n846 = local write "SoundCard"(w1574) -> ()
      }
      event "AI_Vp": Value Change {
        w1589 = 0.01 ("y")
        n847 = event-data() -> ("NewVal"=w1590:dbl)  [unwired: 1 out]
        n848 = Greater?(x=w1590, y=w1589) -> (0:w1591:bool)
        n849 = local read "I_Channel Info"() -> (w1597:T2[])
        n850 = property on="AI_SoundCard Channel" class="Ring (strict)"() -> ("Value"=w1596:u16)  [unwired: 2 in, 2 out]
        n851 = Select(t=w1590, s=w1591, f=w1589) -> (s? t:f=w1588:dbl)
        n852 = Index Array(array=w1597, index=w1596) -> (element=w1599:T2)
        n853 = Bundle By Name(cluster=w1599, "Vmax (V)"=w1588) -> (w1598:T2)
        n854 = property on="AI_Vp" class="DigNum (strict)"("Value"=w1588) -> ()  [unwired: 2 in, 2 out]
        n855 = Replace Array Subset(array=w1597, new element=w1598, index=w1596) -> (w1592:T2[])
        n856 = local write "I_Channel Info"(w1592) -> ()
        n857 = local read "O_Channel Info"() -> (w1595:T2[])
        n858 = local read "SoundCard"() -> (w1594:T5)
        n859 = Insert Into Array(array=w1595, new element=w1592) -> (w1593:T2[])  [unwired: 1 in]
        n860 = Bundle By Name(cluster=w1594, "Channel Array"=w1593) -> (w1587:T5)
        n861 = local write "SoundCard"(w1587) -> ()
      }
      event "D_Enable": Value Change {
        n862 = event-data() -> ("NewVal"=w1603:bool)  [unwired: 1 out]
        n863 = Select(t=u8 0 ("Disabled"), s=w1603, f=u8 2 ("Disabled")) -> (s? t:f=w1604:u8)
        n864 = property on="D_Device ID" class="DigNum (strict)"("Disabled"=w1604) -> ()  [unwired: 2 in, 2 out]
        n865 = property on="D_No.of Ports" class="DigNum (strict)"("Disabled"=w1604) -> ()  [unwired: 2 in, 2 out]
        n866 = property on="D_Port No." class="Ring (strict)"("Disabled"=w1604) -> ()  [unwired: 2 in, 2 out]
        n867 = property on="D_PortWidth" class="DigNum (strict)"("Disabled"=w1604) -> ()  [unwired: 2 in, 2 out]
        n868 = property on="D_Select Channel" class="RadioBtnsControl (strict)"("Disabled"=w1604) -> ()  [unwired: 2 in, 2 out]
        n869 = Boolean To (0,1)(Boolean=w1603) -> (0, 1=w1601:i16)
        n870 = local read "SoundCard"() -> (w1602:T5)
        n871 = Bundle By Name(cluster=w1602, "Digital I/O"=w1601) -> (w1600:T5)
        n872 = local write "SoundCard"(w1600) -> ()
      }
      event "D_No.of Ports": Value Change {
        # "Digital I/O"
        n873 = event-data() -> ("NewVal"=w1608:u8)  [unwired: 1 out]
        n874 = for {
          N: w1608 -> [_]
          shift-right: [w1625] -> w1612
          shift-left: T9 [] -> [w1624]
          i -> [w1626]
          n875 = Increment(x=w1626) -> (x+1=w1622:i32)
          n876 = Bundle By Name(cluster=T10 {"port #"=0, "width"=0, "direction"=0} ("element"), "port #"=w1622, "width"=i16 8, "direction"=0) -> (w1623:T10)
          n877 = Insert Into Array(array=w1624, new element=w1623) -> (w1625:T9)  [unwired: 1 in]
        }
        n878 = local read "SoundCard"() -> (w1616:T5)
        n879 = Bundle By Name(cluster=w1616, "N ports"=w1608, "Dig I/O Ports"=w1612) -> (w1607:T5)
        n880 = Index Array(array=w1612, index=0) -> (element=w1615:T10)
        n881 = call "CRYGet Digital Port Array.vi"("Dig I/O Ports"=w1612) -> ("Digital Port Array"=w1618:cluster{"String":string, "Value":ext}[])  [unwired: 10 out]
        n882 = Unbundle By Name(w1615) -> ("port #"=w1613:i16, "width"=w1610:i16, "direction"=w1611:i32)
        n883 = property on="D_Port No." class="Ring (strict)"("StringsAndValues[]"=w1618) -> ()  [unwired: 2 in, 2 out]
        n884 = local write "SoundCard"(w1607) -> ()
        n885 = Decrement(x=w1613) -> (x-1=w1609:i16)
        n886 = property on="D_Select Channel" class="RadioBtnsControl (strict)"("Value"=w1611) -> ()  [unwired: 2 in, 2 out]
        n887 = property on="D_PortWidth" class="DigNum (strict)"("Value"=w1610) -> ()  [unwired: 2 in, 2 out]
        n888 = property on="D_Port No." class="Ring (strict)"("Value"=w1609) -> ()  [unwired: 2 in, 2 out]
      }
      event "D_Port No.": Value Change {
        n889 = event-data() -> ("NewVal"=w1627:u32)  [unwired: 1 out]
        n890 = local read "SoundCard"() -> (w1632:T5)
        n891 = Unbundle By Name(w1632) -> ("Dig I/O Ports"=w1630:T9)
        n892 = Index Array(array=w1630, index=w1627) -> (element=w1631:T10)
        n893 = Unbundle By Name(w1631) -> ("width"=w1628:i16, "direction"=w1629:i32)
        n894 = property on="D_Select Channel" class="RadioBtnsControl (strict)"("Value"=w1629) -> ()  [unwired: 2 in, 2 out]
        n895 = property on="D_PortWidth" class="DigNum (strict)"("Value"=w1628) -> ()  [unwired: 2 in, 2 out]
      }
      event "D_PortWidth": Value Change {
        n896 = event-data() -> ("NewVal"=w1635:u32)  [unwired: 1 out]
        n897 = local read "SoundCard"() -> (w1636:T5)
        n898 = Unbundle By Name(w1636) -> ("Dig I/O Ports"=w1640:T9)
        n899 = property on="D_Port No." class="Ring (strict)"() -> ("Value"=w1634:u32)  [unwired: 2 in, 2 out]
        n900 = Index Array(array=w1640, index=w1634) -> (element=w1639:T10)
        n901 = Bundle By Name(cluster=w1639, "width"=w1635) -> (w1638:T10)
        n902 = Replace Array Subset(array=w1640, new element=w1638, index=w1634) -> (w1637:T9)
        n903 = Bundle By Name(cluster=w1636, "Dig I/O Ports"=w1637) -> (w1633:T5)
        n904 = local write "SoundCard"(w1633) -> ()
      }
      event "D_Select Channel": Value Change {
        n905 = event-data() -> ("NewVal"=w1645:enum32{"Radio Selection 1", "Radio Selection 2"})  [unwired: 1 out]
        n906 = local read "SoundCard"() -> (w1643:T5)
        n907 = Unbundle By Name(w1643) -> ("Dig I/O Ports"=w1648:T9)
        n908 = property on="D_Port No." class="Ring (strict)"() -> ("Value"=w1642:u32)  [unwired: 2 in, 2 out]
        n909 = Index Array(array=w1648, index=w1642) -> (element=w1647:T10)
        n910 = Bundle By Name(cluster=w1647, "direction"=w1645) -> (w1646:T10)
        n911 = Replace Array Subset(array=w1648, new element=w1646, index=w1642) -> (w1644:T9)
        n912 = Bundle By Name(cluster=w1643, "Dig I/O Ports"=w1644) -> (w1641:T5)
        n913 = local write "SoundCard"(w1641) -> ()
      }
      event "I_How many": Value Change {
        n914 = event-data() -> ("OldVal"=w1655:u32, "NewVal"=w1650:u32)  [unwired: 1 out]
        n915 = local read "SoundCard"() -> (w1662:T5)
        n916 = Unbundle By Name(w1662) -> ("Interf settings"=w1652:T14, "N interfs"=w1661:i32)
        n917 = call "CRYGet Interface Array.vi"("N interfs"=w1650) -> ("Interface no Array"=w1663:cluster{"String":string, "Value":ext}[])  [unwired: 10 out]
        n918 = property on="I_No" class="Ring (strict)"("StringsAndValues[]"=w1663) -> ()  [unwired: 2 in, 2 out]
        n919 = To Double Precision Float(number=w1661) -> (double precision float=w1657:dbl)
        n920 = Subtract(x=w1657, y=w1650) -> (x-y=w1658:dbl)
        n921 = Absolute Value(x=w1658) -> (abs(x)=w1656:dbl)
        n922 = Less Than 0?(x=w1658) -> (x < 0?=w1660:bool)
        n923 = To Unsigned Long Integer(number=w1656) -> (unsigned 32bit integer=w1654:u32)
        n924 = case shown="True" w1660 {
          tunnel: w1652 -> [w1676 w1680]
          tunnel: [w1675 w1678] -> w1659
          tunnel: w1654 -> [w1674 w1677]
          tunnel: w1650 -> [w1673 _]
          frame False {
            n925 = Delete From Array(array=w1676, length=w1674, index=w1673) -> (array with subset deleted=w1675:T14)  [unwired: 1 out]
          }
          frame True {
            # "Insert"
            n926 = for {
              N: w1677 -> [_]
              tunnel: T11 {"Type"=0, "COM Port"=0, "Baud rate"=0, "Data bits"=0, "Parity"=0, "Stop bits"=0, "Flow control"=0, "Dev ID IEEE"=0} ("element") -> [w1690]
              shift-right: [w1689] -> w1678
              shift-left: w1680 -> [w1691]
              w1681 = u8 2 items=["Xon/Xoff", "Hardware", "None"] ("I_Flow control")
              w1682 = u8 0 items=["None", "Odd", "Even", "Mark", "Space"] ("I_Parity")
              w1683 = u8 1 items=["IEEE-488", "RS-232", "Footswitch", "Buzzer"] ("I_Type")
              n927 = Bundle By Name(cluster=w1690, "Type"=w1683, "COM Port"=u8 1, "Baud rate"=u32 9600, "Data bits"=u32 8, "Parity"=w1682, "Stop bits"=u16 0, "Flow control"=w1681, "Dev ID IEEE"=u8 1) -> (w1692:T11)
              n928 = Insert Into Array(array=w1691, new element=w1692) -> (w1689:T14)  [unwired: 1 in]
            }
          }
        }
        n929 = To Long Integer(number=w1650) -> (32bit integer=w1653:i32)
        n930 = Equal To 0?(x=w1653) -> (x = 0?=w1651:bool)
        n931 = Bundle By Name(cluster=w1662, "N interfs"=w1653, "Interf settings"=w1659) -> (w1649:T5)
        n932 = case shown="False" w1651 {
          tunnel: w1655 -> [w1666 _]
          frame False {
            n933 = Equal To 0?(x=w1666) -> (x = 0?=w1665:bool)
            n934 = case shown="True" w1665 {
              frame False {
              }
              frame True {
                n935 = property on="I_No" class="Ring (strict)"("Disabled"=u8 0) -> ()  [unwired: 2 in, 2 out]
                n936 = property on="I_Type" class="Ring (strict)"("Disabled"=u8 0 ("Value (Signaling)")) -> ()  [unwired: 2 in, 2 out]
                n937 = property on="I_Type" class="Ring (strict)"("Val(Sgnl)"=u8 0 ("Value (Signaling)")) -> ()  [unwired: 2 in, 2 out]
              }
            }
            n938 = property on="I_No" class="Ring (strict)"("Val(Sgnl)"=u32 0 ("Value (Signaling)")) -> ()  [unwired: 2 in, 2 out]
          }
          frame True {
            n939 = property on="I_No" class="Ring (strict)"("Disabled"=u8 2) -> ()  [unwired: 2 in, 2 out]
            n940 = property on="I_Type" class="Ring (strict)"("Val(Sgnl)"=u8 0 ("Value (Signaling)")) -> ()  [unwired: 2 in, 2 out]
            n941 = property on="I_Type" class="Ring (strict)"("Disabled"=u8 2 ("Value (Signaling)")) -> ()  [unwired: 2 in, 2 out]
          }
        }
        n942 = local write "SoundCard"(w1649) -> ()
      }
      event "I_No": Value Change {
        n943 = event-data() -> ("NewVal"=w1693:u32)  [unwired: 1 out]
        n944 = local read "SoundCard"() -> (w1694:T5)
        n945 = Unbundle By Name(w1694) -> ("Interf settings"=w1704:T14)
        n946 = Index Array(array=w1704, index=w1693) -> (element=w1703:T11)
        n947 = Unbundle By Name(w1703) -> ("Type"=w1695:u16, "COM Port"=w1702:u8, "Baud rate"=w1701:u32, "Data bits"=w1700:u32, "Parity"=w1699:u16, "Stop bits"=w1698:u16, "Flow control"=w1697:u16, "Dev ID IEEE"=w1696:u8)
        n948 = local write "I_Flow control"(w1697) -> ()
        n949 = local write "I_COM Port"(w1702) -> ()
        n950 = local write "I_Data bits"(w1700) -> ()
        n951 = local write "I_Stop bits"(w1698) -> ()
        n952 = local write "I_Baud"(w1701) -> ()
        n953 = local write "I_Parity"(w1699) -> ()
        n954 = local write "I_Dev ID IEEE"(w1696) -> ()
        n955 = property on="I_Type" class="Ring (strict)"("Val(Sgnl)"=w1695) -> ()  [unwired: 2 in, 2 out]
      }
      event "I_Type": Value Change {
        n956 = event-data() -> ("NewVal"=w1712:u8)  [unwired: 1 out]
        n957 = Equal To 0?(x=w1712) -> (x = 0?=w1718:bool)
        n958 = Not(x=w1718) -> (.not. x?=w1719:bool)
        n959 = property on="I_COM Port" class="DigNum (strict)"("Visible"=w1719) -> ()  [unwired: 2 in, 2 out]
        n960 = property on="I_Baud" class="DigNum (strict)"("Visible"=w1719) -> ()  [unwired: 2 in, 2 out]
        n961 = property on="I_Data bits" class="DigNum (strict)"("Visible"=w1719) -> ()  [unwired: 2 in, 2 out]
        n962 = property on="I_Parity" class="Ring (strict)"("Visible"=w1719) -> ()  [unwired: 2 in, 2 out]
        n963 = property on="I_Stop bits" class="Ring (strict)"("Visible"=w1719) -> ()  [unwired: 2 in, 2 out]
        n964 = property on="I_Flow control" class="Ring (strict)"("Visible"=w1719) -> ()  [unwired: 2 in, 2 out]
        n965 = property on="I_Dev ID IEEE" class="DigNum (strict)"("Visible"=w1718) -> ()  [unwired: 2 in, 2 out]
        n966 = property on="I_How many" class="DigNum (strict)"() -> ("Value"=w1716:u32)  [unwired: 2 in, 2 out]
        n967 = local read "SoundCard"() -> (w1709:T5)
        n968 = Equal To 0?(x=w1716) -> (x = 0?=w1717:bool)
        n969 = Select(t=u8 2 ("Disabled"), s=w1717, f=u8 0 ("Disabled")) -> (s? t:f=w1714:u8)
        n970 = Unbundle By Name(w1709) -> ("Interf settings"=w1708:T14)
        n971 = property on="I_Dev ID IEEE" class="DigNum (strict)"("Disabled"=w1714) -> ()  [unwired: 2 in, 2 out]
        n972 = local read "I_No"() -> (w1711:u32)
        n973 = Index Array(array=w1708, index=w1711) -> (element=w1707:T11)
        n974 = Bundle By Name(cluster=w1707, "Type"=w1712) -> (w1706:T11)
        n975 = Replace Array Subset(array=w1708, new element=w1706, index=w1711) -> (w1710:T14)
        n976 = Bundle By Name(cluster=w1709, "Interf settings"=w1710) -> (w1705:T5)
        n977 = local write "SoundCard"(w1705) -> ()
      }
      event "I_COM Port": Value Change {
        n978 = event-data() -> ("NewVal"=w1721:u8)  [unwired: 1 out]
        n979 = local read "SoundCard"() -> (w1725:T5)
        n980 = Unbundle By Name(w1725) -> ("Interf settings"=w1724:T14)
        n981 = local read "I_No"() -> (w1727:u32)
        n982 = Index Array(array=w1724, index=w1727) -> (element=w1723:T11)
        n983 = Bundle By Name(cluster=w1723, "COM Port"=w1721) -> (w1722:T11)
        n984 = property on="I_COM Port" class="DigNum (strict)"("Value"=w1721) -> ()  [unwired: 2 in, 2 out]
        n985 = Replace Array Subset(array=w1724, new element=w1722, index=w1727) -> (w1726:T14)
        n986 = Bundle By Name(cluster=w1725, "Interf settings"=w1726) -> (w1720:T5)
        n987 = local write "SoundCard"(w1720) -> ()
      }
      event "I_Baud": Value Change {
        n988 = event-data() -> ("NewVal"=w1730:u16)  [unwired: 6 out]
        n989 = local read "SoundCard"() -> (w1733:T5)
        n990 = Unbundle By Name(w1733) -> ("Interf settings"=w1732:T14)
        n991 = local read "I_No"() -> (w1735:u32)
        n992 = Index Array(array=w1732, index=w1735) -> (element=w1731:T11)
        n993 = Bundle By Name(cluster=w1731, "Baud rate"=w1730) -> (w1729:T11)
        n994 = Replace Array Subset(array=w1732, new element=w1729, index=w1735) -> (w1734:T14)
        n995 = Bundle By Name(cluster=w1733, "Interf settings"=w1734) -> (w1728:T5)
        n996 = local write "SoundCard"(w1728) -> ()
      }
      event "I_Data bits": Value Change {
        n997 = event-data() -> ("NewVal"=w1737:u8)  [unwired: 1 out]
        n998 = local read "SoundCard"() -> (w1741:T5)
        n999 = Unbundle By Name(w1741) -> ("Interf settings"=w1740:T14)
        n1000 = local read "I_No"() -> (w1743:u32)
        n1001 = Index Array(array=w1740, index=w1743) -> (element=w1739:T11)
        n1002 = Bundle By Name(cluster=w1739, "Data bits"=w1737) -> (w1738:T11)
        n1003 = Replace Array Subset(array=w1740, new element=w1738, index=w1743) -> (w1742:T14)
        n1004 = Bundle By Name(cluster=w1741, "Interf settings"=w1742) -> (w1736:T5)
        n1005 = local write "SoundCard"(w1736) -> ()
      }
      event "I_Parity": Value Change {
        n1006 = event-data() -> ("NewVal"=w1746:u8)  [unwired: 1 out]
        n1007 = local read "SoundCard"() -> (w1749:T5)
        n1008 = Unbundle By Name(w1749) -> ("Interf settings"=w1748:T14)
        n1009 = local read "I_No"() -> (w1751:u32)
        n1010 = Index Array(array=w1748, index=w1751) -> (element=w1747:T11)
        n1011 = Bundle By Name(cluster=w1747, "Parity"=w1746) -> (w1745:T11)
        n1012 = Replace Array Subset(array=w1748, new element=w1745, index=w1751) -> (w1750:T14)
        n1013 = Bundle By Name(cluster=w1749, "Interf settings"=w1750) -> (w1744:T5)
        n1014 = local write "SoundCard"(w1744) -> ()
      }
      event "I_Stop bits": Value Change {
        n1015 = event-data() -> ("NewVal"=w1754:u8)  [unwired: 1 out]
        n1016 = local read "SoundCard"() -> (w1757:T5)
        n1017 = Unbundle By Name(w1757) -> ("Interf settings"=w1756:T14)
        n1018 = local read "I_No"() -> (w1759:u32)
        n1019 = Index Array(array=w1756, index=w1759) -> (element=w1755:T11)
        n1020 = Bundle By Name(cluster=w1755, "Stop bits"=w1754) -> (w1753:T11)
        n1021 = Replace Array Subset(array=w1756, new element=w1753, index=w1759) -> (w1758:T14)
        n1022 = Bundle By Name(cluster=w1757, "Interf settings"=w1758) -> (w1752:T5)
        n1023 = local write "SoundCard"(w1752) -> ()
      }
      event "I_Flow control": Value Change {
        n1024 = event-data() -> ("NewVal"=w1762:u8)  [unwired: 1 out]
        n1025 = local read "SoundCard"() -> (w1765:T5)
        n1026 = Unbundle By Name(w1765) -> ("Interf settings"=w1764:T14)
        n1027 = local read "I_No"() -> (w1767:u32)
        n1028 = Index Array(array=w1764, index=w1767) -> (element=w1763:T11)
        n1029 = Bundle By Name(cluster=w1763, "Flow control"=w1762) -> (w1761:T11)
        n1030 = Replace Array Subset(array=w1764, new element=w1761, index=w1767) -> (w1766:T14)
        n1031 = Bundle By Name(cluster=w1765, "Interf settings"=w1766) -> (w1760:T5)
        n1032 = local write "SoundCard"(w1760) -> ()
      }
      event "I_Dev ID IEEE": Value Change {
        n1033 = event-data() -> ("NewVal"=w1769:u8)  [unwired: 1 out]
        n1034 = local read "SoundCard"() -> (w1773:T5)
        n1035 = Unbundle By Name(w1773) -> ("Interf settings"=w1772:T14)
        n1036 = local read "I_No"() -> (w1775:u32)
        n1037 = Index Array(array=w1772, index=w1775) -> (element=w1771:T11)
        n1038 = Bundle By Name(cluster=w1771, "Dev ID IEEE"=w1769) -> (w1770:T11)
        n1039 = Replace Array Subset(array=w1772, new element=w1770, index=w1775) -> (w1774:T14)
        n1040 = Bundle By Name(cluster=w1773, "Interf settings"=w1774) -> (w1768:T5)
        n1041 = local write "SoundCard"(w1768) -> ()
      }
      event "DC_Enable": Value Change {
        n1042 = event-data() -> ("NewVal"=w1777:bool)  [unwired: 6 out]
        n1043 = local read "SoundCard"() -> (w1778:T5)
        n1044 = Bundle By Name(cluster=w1778, "udev enable"=w1777) -> (w1776:T5)
        n1045 = Select(t=u8 0 ("Disabled"), s=w1777, f=u8 2 ("Disabled")) -> (s? t:f=w1779:u8)
        n1046 = property on="DC_Table" class="Tbl (strict)"("Disabled"=w1779) -> ()  [unwired: 2 in, 2 out]
        n1047 = local write "SoundCard"(w1776) -> ()
      }
      event "DC_Table": Value Change {
        n1048 = event-data() -> ("NewVal"=w1788:string[][])  [unwired: 1 out]
        n1049 = Index Array(array=w1788, index (row)=0, index (col)=0 ("disabled index (col)")) -> (element=w1785:string)
        n1050 = Decimal String To Number(string=w1785) -> (number=w1784:i32)  [unwired: 3 out]
        n1051 = Build Array(w1784) -> (w1783:i32[])
        n1052 = local read "SoundCard"() -> (w1789:T5)
        n1053 = Bundle By Name(cluster=w1789, "udev SNs"=w1783) -> (w1782:T5)
        n1054 = local write "SoundCard"(w1782) -> ()
      }
      event "Calibration Seq": Value Change {
        n1055 = event-data() -> ()  [unwired: 2 out]
        n1056 = property on="Calibration Seq" class="Ring (strict)"() -> ("RingText.Text"=w1791:string)  [unwired: 2 in, 2 out]
        n1057 = local read "SoundCard"() -> (w1792:T5)
        n1058 = Bundle By Name(cluster=w1792, "Cal sequence"=w1791) -> (w1790:T5)
        n1059 = local write "SoundCard"(w1790) -> ()
      }
      event "Help": Value Change {
        n1060 = event-data() -> ("NewVal"=w1794:string)  [unwired: 1 out]
        n1061 = local read "SoundCard"() -> (w1795:T5)
        n1062 = Bundle By Name(cluster=w1795, "Help"=w1794) -> (w1793:T5)
        n1063 = local write "SoundCard"(w1793) -> ()
      }
    }
    n1064 = global read "CRYMain Sub Window Global.vi" "gStop"() -> (w44:bool)
    n1065 = Or(x="Refresh", y="Load Test") -> (x .or. y?=w32:bool)
    n1066 = Or(x=w44, y="stop") -> (x .or. y?=w29:bool)
    n1067 = Bundle(w32, "AO_Add"="AO_Add", "AO_Delete"="AO_Delete", "AO_Rename"="AO_Rename", "AI_Add"="AI_Add", "AI_Delete"="AI_Delete", "AI_Rename"="AI_Rename", "Open_Table"="Open_Table", "Calibrartion"="Calibrartion", "SaveSoundCard"="SaveSoundCard", "Cancel"="Cancel") -> (w48:T15)  [unwired: 1 out]
    n1068 = local read "O_Channel Info"() -> (w31:T2[])
    n1069 = local read "I_Channel Info"() -> (w30:T2[])
    n1070 = Cluster To Array(cluster=w48) -> (array=w47:bool[])
    n1071 = Search 1D Array(1D array=w47, element=TRUE) -> (index of element=w45:i32)  [unwired: 1 out]
    n1072 = case shown="9" w45 {
      selector: w45 -> [_ w287 _ _ _ _ _ _]
      tunnel: w31 -> [w63 _ _ _ _ _ _ _]
      tunnel: w30 -> [w62 _ _ _ _ _ _ _]
      frame 0 {
        n1073 = flat-sequence {
          tunnel: [w110] -> w59
          tunnel: [w111] -> w61
          tunnel: [w66] -> w57
          tunnel: [w73] -> w55
          tunnel: [w72] -> w53
          tunnel: w63 -> [w77]
          tunnel: w62 -> [w76]
          tunnel: [w71] -> w51
          tunnel: [w70] -> w50
          tunnel: w61 -> [w133]
          tunnel: [w133] -> w60
          tunnel: w59 -> [w132]
          tunnel: [w132] -> w58
          tunnel: w57 -> [w131]
          tunnel: [w131] -> w56
          tunnel: w55 -> [w127]
          tunnel: [w127] -> w54
          tunnel: w53 -> [w128]
          tunnel: [w128] -> w52
          tunnel: w51 -> [w130]
          tunnel: w50 -> [w129]
          tunnel: [w253] -> w65
          tunnel: [w252] -> w64
          tunnel: w60 -> [w252]
          tunnel: w58 -> [w253]
          tunnel: w56 -> [w198]
          tunnel: w54 -> [w181]
          tunnel: w52 -> [w187]
          tunnel: w65 -> [w260]
          tunnel: w64 -> [w259]
          frame #0 {
            w78 = enum16{"Load", "SaveAs", "Revert"}."Load" ("Mode")
            # "DC Connect"
            # "Interface"
            # "Digital I/O"
            # "Get Current Device"
            n1074 = flat-sequence {
              tunnel: [w112] -> w89
              frame #0 {
                n1075 = call "CRYClose All Operator.vi"() -> ()  [unwired: 12 in]
              }
              frame #1 {
                n1076 = local read "SoundCard"() -> (w112:T5)
              }
            }
            n1077 = call "CRYGet Default Hardware.vi"("Hardware Cluster In"=w89) -> ("Hardware Cluster Out"=w66:T5, "O_Device Info Out"=w87:T3, "AO_Hardware Channel Name Out"=w108:string[], "I_Device Info Out"=w107:T3, "AI_Hardware Channel Name Out"=w109:string[], "O_Channel Info Out"=w74:T2[], "I_Channel Info Out"=w75:T2[], "Real Output Device Name Out"=w72:cluster{"MME":string[], "ASIO":string[]}, "Real Input Device Name Out"=w73:cluster{"MME":string[], "ASIO":string[]}, "Error"=w110:bool, "No Device Name"=w111:string[])  [unwired: 8 out]
            n1078 = local write "O_Channel Info"(w74) -> ()
            n1079 = local write "O_Device Info"(w87) -> ()
            n1080 = local write "I_Channel Info"(w75) -> ()
            n1081 = local write "I_Device Info"(w107) -> ()
            n1082 = property on="AI_SoundCard Channel" class="Ring (strict)"("Strings []"=w109) -> ()  [unwired: 2 in, 2 out]
            n1083 = property on="AO_SoundCard Channel" class="Ring (strict)"("Strings []"=w108) -> ()  [unwired: 2 in, 2 out]
            n1084 = local write "SoundCard"(w66) -> ()
            n1085 = call "CRYGet IOChannel Name.vi"("O_Channel Info In"=w74, "I_Channel Info In"=w75) -> ("O_Name Out"=w80:string[][], "I_Name Out"=w83:string[][])  [unwired: 7 in]
            n1086 = property on="I_Name" class="Arr (strict)"() -> ("Value"=w84:string[][])  [unwired: 2 in, 2 out]
            n1087 = property on="O_Name" class="Arr (strict)"() -> ("Value"=w81:string[][])  [unwired: 2 in, 2 out]
            n1088 = Unbundle By Name(w66) -> ("Digital I/O"=w86:u16, "Dig Dev ID"=w96:u8, "N ports"=w95:u8, "Dig I/O Ports"=w90:T9, "SelectedOut"=w71:u16, "SelectedIn"=w70:u16)
            n1089 = Unbundle By Name(w66) -> ("Interf settings"=w88:T14)
            n1090 = call "CRYFlatten SoundCard.vi"("SoundCard"=w66) -> ("SoundCard flattened"=w69:string)  [unwired: 10 in]
            n1091 = Unbundle By Name(w66) -> ("udev SNs"=w101:i16[], "udev enable"=w106:bool)
            n1092 = call "CRYSet Channel State.vi"("New Channel Info"=w75, "Old Channel Info"=w76, "New Name In"=w83, "Old Name In"=w84, "Mode"=w78) -> ("Name Out"=→"I_Name":string[][])  [unwired: 6 in]
            n1093 = call "CRYSet Channel State.vi"("New Channel Info"=w74, "Old Channel Info"=w77, "New Name In"=w80, "Old Name In"=w81, "Mode"=w78) -> ("Name Out"=→"O_Name":string[][])  [unwired: 6 in]
            n1094 = global read "CRYProject Editor Global.vi" "SoundCard Step"() -> (w68:T6)
            n1095 = Bundle By Name(cluster=w68, "Seq setup flattened"=w69) -> (w67:T6)
            n1096 = Not Equal To 0?(x=w86) -> (x != 0?=w85:bool)
            n1097 = Array Size(array=w88) -> (size(s)=w99:i32)
            n1098 = property on="D_Device ID" class="DigNum (strict)"("Value"=w96) -> ()  [unwired: 2 in, 2 out]
            n1099 = property on="D_No.of Ports" class="DigNum (strict)"("Value"=w95) -> ()  [unwired: 2 in, 2 out]
            n1100 = Number To Decimal String(number=w101) -> (decimal integer string=w100:string[])  [unwired: 1 out]
            n1101 = property on="D_Enable" class="Bool (strict)"("Val(Sgnl)"=w85) -> ()  [unwired: 2 in, 2 out]
            n1102 = call "CRYGet Interface Array.vi"("N interfs"=w99) -> ("Interface no Array"=w97:cluster{"String":string, "Value":ext}[])  [unwired: 10 out]
            n1103 = Select(t=u8 0 ("Disabled"), s=w106, f=u8 2 ("Disabled")) -> (s? t:f=w104:u8)
            n1104 = Build Array(w100) -> (w105:string[][])
            n1105 = call "CRYGet Digital Port Array.vi"("Dig I/O Ports"=w90) -> ("Digital Port Array"=w91:cluster{"String":string, "Value":ext}[])  [unwired: 10 out]
            n1106 = Index Array(array=w90, index=0) -> (element=w93:T10)
            n1107 = property on="I_No" class="Ring (strict)"("StringsAndValues[]"=w97) -> ()  [unwired: 2 in, 2 out]
            n1108 = property on="DC_Table" class="Tbl (strict)"("Disabled"=w104) -> ()  [unwired: 2 in, 2 out]
            n1109 = property on="I_How many" class="DigNum (strict)"("Value"=w99) -> ()  [unwired: 2 in, 2 out]
            n1110 = property on="DC_Table" class="Tbl (strict)"("Value"=w105) -> ()  [unwired: 2 in, 2 out]
            n1111 = global write "CRYProject Editor Global.vi" "SoundCard Step"(w67) -> ()
            n1112 = Unbundle By Name(w93) -> ("port #"=w92:i16)
            n1113 = property on="D_Port No." class="Ring (strict)"("StringsAndValues[]"=w91) -> ()  [unwired: 2 in, 2 out]
            n1114 = property on="DC_Enable" class="Bool (strict)"("Value"=w106) -> ()  [unwired: 2 in, 2 out]
            n1115 = Equal To 0?(x=w99) -> (x = 0?=w98:bool)
            n1116 = property on="D_Port No." class="Ring (strict)"("Val(Sgnl)"=w92) -> ()  [unwired: 2 in, 2 out]
            n1117 = case shown="False" w98 {
              tunnel: w88 -> [w116 _]
              frame False {
                n1118 = Index Array(array=w116, index=1) -> (element=w114:T11)
                n1119 = Unbundle By Name(w114) -> ("Type"=w113:u16)
                n1120 = property on="I_Type" class="Ring (strict)"("Val(Sgnl)"=w113) -> ()  [unwired: 2 in, 2 out]
                n1121 = property on="I_No" class="Ring (strict)"("Val(Sgnl)"=u32 0 ("Value (Signaling)")) -> ()  [unwired: 2 in, 2 out]
                n1122 = property on="I_No" class="Ring (strict)"("Disabled"=u8 0) -> ()  [unwired: 2 in, 2 out]
                n1123 = property on="I_Type" class="Ring (strict)"("Disabled"=u8 0 ("Value (Signaling)")) -> ()  [unwired: 2 in, 2 out]
              }
              frame True {
                n1124 = property on="I_No" class="Ring (strict)"("Disabled"=u8 2) -> ()  [unwired: 2 in, 2 out]
                n1125 = property on="I_Type" class="Ring (strict)"("Val(Sgnl)"=u8 0 ("Value (Signaling)")) -> ()  [unwired: 2 in, 2 out]
                n1126 = property on="I_Type" class="Ring (strict)"("Disabled"=u8 2 ("Value (Signaling)")) -> ()  [unwired: 2 in, 2 out]
              }
            }
          }
          frame #1 {
            n1127 = local read "O_Device Info"() -> (w126:T3)
            n1128 = local read "I_Device Info"() -> (w123:T3)
            n1129 = flat-sequence {
              tunnel: w130 -> [w163]
              tunnel: w129 -> [w161]
              frame #0 {
                n1130 = local read "O_Channel Info"() -> (w162:T2[])
                n1131 = local read "I_Channel Info"() -> (w160:T2[])
                n1132 = Index Array(array=w160, index=w161) -> (element=w158:T2)
                n1133 = Index Array(array=w162, index=w163) -> (element=w159:T2)
                n1134 = Unbundle By Name(w158) -> ("Audio Driver"=w151:u16)
                n1135 = Unbundle By Name(w159) -> ("Audio Driver"=w157:u16)
                n1136 = Equal To 0?(x=w157) -> (x = 0?=w156:bool)
                n1137 = Equal To 0?(x=w151) -> (x = 0?=w152:bool)
                n1138 = Select(t=w151, s=w152, f=u16 1) -> (s? t:f=w150:u16)
                n1139 = local write "AI_Audio Driver"(w150) -> ()
                n1140 = Select(t=w157, s=w156, f=u16 1) -> (s? t:f=w154:u16)
                n1141 = local write "AO_Audio Driver"(w154) -> ()
              }
              frame #1 {
                n1142 = local read "O_Channel Info"() -> (w170:T2[])
                n1143 = local read "I_Channel Info"() -> (w169:T2[])
                n1144 = local read "O_Device Info"() -> (w164:T3)
                n1145 = property on="AO_Audio Driver" class="RadioBtnsControl (strict)"() -> ("Value"=w171:enum32{"Radio Selection 1", "Radio Selection 2"})  [unwired: 2 in, 2 out]
                n1146 = local read "I_Device Info"() -> (w168:T3)
                n1147 = property on="AI_Audio Driver" class="RadioBtnsControl (strict)"() -> ("Value"=w172:enum32{"Radio Selection 1", "Radio Selection 2"})  [unwired: 2 in, 2 out]
                n1148 = call "CRYGet Disable Device State.vi"("I_Channel Info"=w169, "I_Device Info In"=w168, "Audio Driver"=w172, "In/Out"=TRUE) -> ("Device Names"=w174:string[], "Disabled Items"=w175:i32[])  [unwired: 5 in, 1 out]
                n1149 = call "CRYGet Disable Device State.vi"("O_Channel Info"=w170, "O_Device Info In"=w164, "Audio Driver"=w171, "In/Out"=FALSE) -> ("Device Names"=w173:string[], "Disabled Items"=w166:i32[])  [unwired: 5 in, 1 out]
                n1150 = property on="AI_Device Name" class="Ring (strict)"("Strings []"=w174) -> ()  [unwired: 2 in, 2 out]
                n1151 = property on="AI_Device Name" class="Ring (strict)"("Disabled Items []"=w175) -> ()  [unwired: 2 in, 2 out]
                n1152 = property on="AO_Device Name" class="Ring (strict)"("Strings []"=w173) -> ()  [unwired: 2 in, 2 out]
                n1153 = property on="AO_Device Name" class="Ring (strict)"("Disabled Items []"=w166) -> ()  [unwired: 2 in, 2 out]
              }
            }
            n1154 = call "CRYIs Empty Asio Device.vi"("Device Info"=w126) -> ("IsEmptyASIO"=w125:bool)  [unwired: 10 in]
            n1155 = call "CRYIs Empty Asio Device.vi"("Device Info"=w123) -> ("IsEmptyASIO"=w124:bool)  [unwired: 10 in]
            n1156 = case shown="True" w124 {
              frame True {
                n1157 = property on="AI_Audio Driver" class="RadioBtnsControl (strict)"() -> ("Controls[]"=w134:refnum<vi>[])  [unwired: 2 in, 2 out]
                n1158 = Index Array(array=w134, index=1) -> (element=w136:refnum<vi>)
                n1159 = property class="Ctl"(reference=w136, "DisabledEnum"=T7."Disabled and Grayed Out" ("Disabled")) -> ()  [unwired: 1 in, 2 out]
              }
              frame False {
                n1160 = property on="AI_Audio Driver" class="RadioBtnsControl (strict)"() -> ("Controls[]"=w138:refnum<vi>[])  [unwired: 2 in, 2 out]
                n1161 = Index Array(array=w138, index=1) -> (element=w140:refnum<vi>)
                n1162 = property class="Ctl"(reference=w140, "DisabledEnum"=T7."Enabled" ("Disabled")) -> ()  [unwired: 1 in, 2 out]
              }
            }
            n1163 = case shown="False" w125 {
              frame True {
                n1164 = property on="AO_Audio Driver" class="RadioBtnsControl (strict)"() -> ("Controls[]"=w145:refnum<vi>[])  [unwired: 2 in, 2 out]
                n1165 = Index Array(array=w145, index=1) -> (element=w143:refnum<vi>)
                n1166 = property class="Ctl"(reference=w143, "DisabledEnum"=T7."Disabled and Grayed Out" ("Disabled")) -> ()  [unwired: 1 in, 2 out]
              }
              frame False {
                n1167 = property on="AO_Audio Driver" class="RadioBtnsControl (strict)"() -> ("Controls[]"=w149:refnum<vi>[])  [unwired: 2 in, 2 out]
                n1168 = Index Array(array=w149, index=1) -> (element=w147:refnum<vi>)
                n1169 = property class="Ctl"(reference=w147, "DisabledEnum"=T7."Enabled" ("Disabled")) -> ()  [unwired: 1 in, 2 out]
              }
            }
          }
          frame #2 {
            w195 = T7."Enabled" ("Disabled")
            w194 = T7."Disabled and Grayed Out" ("Disabled")
            w204 = u16 0 items=[""] ("AO_Hardware Channel")
            # "Current Device and Setting Device Test"
            # "Tab Position setting/Set Channel Information"
            n1170 = local read "I_Channel Info"() -> (w211:T2[])
            n1171 = local read "O_Channel Info"() -> (w234:T2[])
            n1172 = local read "I_Device Info"() -> (w239:T3)
            n1173 = local read "I_Device Info"() -> (w231:T3)
            n1174 = local read "O_Device Info"() -> (w241:T3)
            n1175 = local read "O_Device Info"() -> (w235:T3)
            n1176 = Unbundle By Name(w198) -> ("SelectedOut"=w203:u16, "SelectedIn"=w202:u16, "Cal sequence"=w216:string, "Help"=w200:string, "Advanced"=w201:bool, "SelectedTab"=w199:u16)
            n1177 = Index Array(array=w234, index=w203) -> (element=w233:T2)
            n1178 = Unbundle By Name(w233) -> ("Device Name"=w236:string, "Sampling Rate (Hz)"=w219:u32, "Anti-aliasing Factor (%fs)"=w228:sgl)
            n1179 = Index Array(array=w211, index=w202) -> (element=w232:T2)
            n1180 = Unbundle By Name(w232) -> ("Device Name"=w230:string, "Sampling Rate (Hz)"=w218:u32, "Anti-aliasing Factor (%fs)"=w229:sgl)
            n1181 = call "CRYGet Device Index to Channel.vi"("Device Name In"=w230, "Device Info In"=w231) -> ("Device Total Index Out"=w177:i32)  [unwired: 8 in, 1 out]
            n1182 = Index Array(array=w239, index=w177) -> (element=w179:T12)
            n1183 = call "CRYGet Device Index to Channel.vi"("Device Name In"=w236, "Device Info In"=w235) -> ("Device Total Index Out"=w176:i32)  [unwired: 8 in, 1 out]
            n1184 = Index Array(array=w241, index=w176) -> (element=w189:T12)
            n1185 = Unbundle By Name(w189) -> ("Channel Names"=w188:string[])
            n1186 = call "CRYGet Freq Bit Array.vi"("Device Infor"=w189) -> ("MaxFreq"=w209:u32, "MinFreq"=w238:u32, "Bit Depth"=w243:cluster{"String":string, "Value":ext}[], "Samplein Rate"=w242:cluster{"String":string, "Value":ext}[])  [unwired: 1 in, 6 out]
            n1187 = call "CRYGet Freq Bit Array.vi"("Device Infor"=w179) -> ("MaxFreq"=w208:u32, "MinFreq"=w237:u32, "Bit Depth"=w240:cluster{"String":string, "Value":ext}[], "Samplein Rate"=w210:cluster{"String":string, "Value":ext}[])  [unwired: 1 in, 6 out]
            n1188 = Unbundle By Name(w179) -> ("Channel Names"=w178:string[])
            n1189 = property on="AI_Sampling Rate" class="Ring (strict)"("StringsAndValues[]"=w210) -> ()  [unwired: 2 in, 2 out]
            n1190 = property on="AI_Sampling User" class="DigNum (strict)"("Maximum"=w208) -> ()  [unwired: 2 in, 2 out]
            n1191 = property on="AO_Sampling Rate" class="Ring (strict)"("StringsAndValues[]"=w242) -> ()  [unwired: 2 in, 2 out]
            n1192 = property on="AO_Sampling User" class="DigNum (strict)"("Maximum"=w209) -> ()  [unwired: 2 in, 2 out]
            n1193 = property on="AO_Sampling Rate" class="Ring (strict)"("Value"=w219) -> ()  [unwired: 2 in, 2 out]
            n1194 = property on="AO_Alias freq" class="DigNum (strict)"("Value"=w228) -> ()  [unwired: 2 in, 2 out]
            n1195 = property on="AI_Sampling Rate" class="Ring (strict)"("Value"=w218) -> ()  [unwired: 2 in, 2 out]
            n1196 = property on="AI_Alias freq" class="DigNum (strict)"("Value"=w229) -> ()  [unwired: 2 in, 2 out]
            n1197 = property on="AI_Sampling User" class="DigNum (strict)"("Minimum"=w237) -> ()  [unwired: 2 in, 2 out]
            n1198 = property on="AI_Select Channel1" class="Ring (strict)"("Strings []"=w178) -> ()  [unwired: 2 in, 2 out]
            n1199 = property on="AO_Select Channel1" class="Ring (strict)"("Strings []"=w188) -> ()  [unwired: 2 in, 2 out]
            n1200 = property on="AO_Sampling User" class="DigNum (strict)"("Minimum"=w238) -> ()  [unwired: 2 in, 2 out]
            n1201 = property on="AI_Bit Depth" class="Ring (strict)"("StringsAndValues[]"=w240) -> ()  [unwired: 2 in, 2 out]
            n1202 = Divide(x=w219, y=2.0) -> (x/y=w221:dbl)
            n1203 = Divide(x=w218, y=2.0) -> (x/y=w224:dbl)
            n1204 = property on="AO_Bit Depth" class="Ring (strict)"("StringsAndValues[]"=w243) -> ()  [unwired: 2 in, 2 out]
            n1205 = property on="AO_Alias freq" class="DigNum (strict)"("Maximum"=w221) -> ()  [unwired: 2 in, 2 out]
            n1206 = property on="AI_Alias freq" class="DigNum (strict)"("Maximum"=w224) -> ()  [unwired: 2 in, 2 out]
            n1207 = property on="AI_Sampling User" class="DigNum (strict)"("Value"=w208) -> ()  [unwired: 2 in, 2 out]
            n1208 = property on="AO_Sampling User" class="DigNum (strict)"("Value"=w209) -> ()  [unwired: 2 in, 2 out]
            n1209 = local read "AddStep"() -> (w190:bool)
            n1210 = property on="AO_Alias freq" class="DigNum (strict)"("Minimum"=0.0 ("Data Entry Limits:Minimum")) -> ()  [unwired: 2 in, 2 out]
            n1211 = property on="AI_Alias freq" class="DigNum (strict)"("Minimum"=0.0 ("Data Entry Limits:Minimum")) -> ()  [unwired: 2 in, 2 out]
            n1212 = property on="Calibration Seq" class="Ring (strict)"() -> ("Strings []"=w217:string[])  [unwired: 2 in, 2 out]
            n1213 = property on="Advanced View" class="Bool (strict)"("Val(Sgnl)"=w201) -> ()  [unwired: 2 in, 2 out]
            n1214 = local write "Help"(w200) -> ()
            n1215 = Equal?(x=w218, y=u32 0) -> (x = y?=w220:bool)
            n1216 = Equal?(x=w219, y=u32 0) -> (x = y?=w226:bool)
            n1217 = property on="AO_Sampling User" class="DigNum (strict)"("Visible"=w226) -> ()  [unwired: 2 in, 2 out]
            n1218 = Search 1D Array(1D array=w217, element=w216) -> (index of element=w214:i32)  [unwired: 1 in]
            n1219 = property on="AI_Sampling User" class="DigNum (strict)"("Visible"=w220) -> ()  [unwired: 2 in, 2 out]
            n1220 = case shown="True" w190 {
              frame False {
              }
              frame True {
                n1221 = local write "Mode"("AddStep" ("Mode")) -> ()
              }
            }
            n1222 = Unbundle By Name(w187) -> ("MME"=w186:string[], "ASIO"=w185:string[])
            n1223 = Greater Than 0?(x=w214) -> (x > 0?=w215:bool)
            n1224 = Unbundle By Name(w181) -> ("MME"=w182:string[], "ASIO"=w183:string[])
            n1225 = Quotient & Remainder(x=w199, y=u16 10) -> (x-y*floor(x/y)=w247:u16, floor(x/y)=w246:u16)
            n1226 = Select(t=w214, s=w215, f=0) -> (s? t:f=w213:i32)
            n1227 = Insert Into Array(array=w186, new element=w185) -> (w184:string[])  [unwired: 1 in]
            n1228 = property on="Main Tab" class="TabCtl (strict)"("Value"=w246) -> ()  [unwired: 2 in, 2 out]
            n1229 = property on="Audio I/O Tab" class="TabCtl (strict)"("Value"=w247) -> ()  [unwired: 2 in, 2 out]
            n1230 = property on="Calibration Seq" class="Ring (strict)"("Value"=w213) -> ()  [unwired: 2 in, 2 out]
            n1231 = Insert Into Array(array=w182, new element=w183) -> (w180:string[])  [unwired: 1 in]
            n1232 = property on="D_No.of Ports" class="DigNum (strict)"("Minimum"=1.0 ("Data Entry Limits:Minimum")) -> ()  [unwired: 2 in, 2 out]
            n1233 = Array Size(array=w184) -> (size(s)=w207:i32)
            n1234 = Array Size(array=w180) -> (size(s)=w191:i32)
            n1235 = Greater Than 0?(x=w191) -> (x > 0?=w197:bool)
            n1236 = Greater Than 0?(x=w207) -> (x > 0?=w192:bool)
            n1237 = control-ref of="Board Tab"() -> (w249:refnum<vi>)
            n1238 = Select(t=w202, s=w197, f=w204) -> (s? t:f=w206:u16)
            n1239 = Select(t=w203, s=w192, f=w204) -> (s? t:f=w205:u16)
            n1240 = control-ref of="This VI"() -> (w251:refnum<vi>)
            n1241 = property on="AO_SoundCard Channel" class="Ring (strict)"("Val(Sgnl)"=w205) -> ()  [unwired: 2 in, 2 out]
            n1242 = Select(t=w195, s=w197, f=w194) -> (s? t:f=w193:T7)
            n1243 = property on="AI_SoundCard Channel" class="Ring (strict)"("Val(Sgnl)"=w206) -> ()  [unwired: 2 in, 2 out]
            n1244 = Select(t=w195, s=w192, f=w194) -> (s? t:f=w196:T7)
            n1245 = call "CRYAlign Steps VI Center.vi"("Tab2"=w249, "Input/Output"=TRUE ("Preview"), "VIRef"=w251) -> ()  [unwired: 1 in, 8 out]
            n1246 = property on="AI_Rename" class="Bool"("DisabledEnum"=w193) -> ()  [unwired: 2 in, 2 out]
            n1247 = property on="AI_Add" class="Bool"("DisabledEnum"=w193) -> ()  [unwired: 2 in, 2 out]
            n1248 = property on="AO_Add" class="Bool"("DisabledEnum"=w196) -> ()  [unwired: 2 in, 2 out]
            n1249 = property on="AO_Rename" class="Bool"("DisabledEnum"=w196) -> ()  [unwired: 2 in, 2 out]
          }
          frame #3 {
            w256 = FALSE ("Load Test")
            # "Apply"
            n1250 = local read "Mode"() -> (w257:string)
            n1251 = property on="Board Tab" class="TabCtl (strict)"("Visible"=TRUE) -> ()  [unwired: 2 in, 2 out]
            n1252 = local write "Load Test"(w256) -> ()
            n1253 = local write "AddStep"(w256) -> ()
            n1254 = case shown="True" w260 {
              tunnel: w259 -> [w270 _]
              frame True {
                w269 = "\r"
                n1255 = Concatenate Strings(w269, w269) -> (w268:string)
                n1256 = for {
                  tunnel: w270 -> [w279] mode=indexing
                  shift-right: [w277] -> w271
                  shift-left: w268 -> [w280]
                  n1257 = Concatenate Strings(w280, w279, "\r") -> (w277:string)
                }
                n1258 = call "CRYGet Error Message.vi"("Error No"=0 ("No"), "Kind"="SoundCard") -> ("Message"=w274:string, "Window Title"=w272:string)  [unwired: 4 in, 4 out]
                n1259 = Format Into String(format string=w274, w271) -> (resulting string=w273:string)  [unwired: 2 in, 1 out]
                n1260 = call "CRYMessage Dialog.vi"("Window Title"=w272, "Message Content"=w273) -> ()  [unwired: 8 in, 2 out]
              }
              frame False {
              }
            }
            n1261 = case shown="\"AddStep\", \"Load\", \"OpenTable\", \"Revert\"" w257 {
              frame "False", Default {
              }
              frame "AddStep", "Load", "OpenTable", "Revert" {
                n1262 = local read "Proper VI No"() -> (w265:i32)
                n1263 = local read "SoundCard"() -> (w262:T5)
                n1264 = property on="I_Name" class="Arr (strict)"() -> ("Value"=w264:string[][])  [unwired: 2 in, 2 out]
                n1265 = property on="O_Name" class="Arr (strict)"() -> ("Value"=w263:string[][])  [unwired: 2 in, 2 out]
                n1266 = call "CRYSoundCard.vi"("O_Name In"=w263, "I_Name In"=w264, "SoundCard In"=w262, "Proper VI No In"=w265) -> ("O_Name Out"=w266:string[][], "I_Name Out"=w267:string[][])  [unwired: 6 in]
                n1267 = local write "Mode"("" ("Mode")) -> ()
                n1268 = property on="I_Name" class="Arr (strict)"("Value"=w267) -> ()  [unwired: 2 in, 2 out]
                n1269 = property on="O_Name" class="Arr (strict)"("Value"=w266) -> ()  [unwired: 2 in, 2 out]
              }
            }
          }
        }
      }
      frame 1..6 {
        # "???"
        # "Delete"
        n1270 = Decrement(x=w287) -> (x-1=w283:i32)
        n1271 = Quotient & Remainder(x=w283, y=3) -> (x-y*floor(x/y)=w285:i32, floor(x/y)=w290:i32)
        n1272 = call "CRYGet Error Message.vi"("Kind"="SoundCard Sub") -> ("Message Sub"=w281:string[])  [unwired: 5 in, 5 out]
        n1273 = Index Array(array=w281, index=w283) -> (element=w288:string)
        n1274 = case shown="0" w290 {
          tunnel: [w467 w475] -> w286
          tunnel: [w461 w469] -> w284
          frame 0 {
            n1275 = property on="AO_SoundCard Channel" class="Ring (strict)"() -> ("Strings []"=w468:string[])  [unwired: 2 in, 2 out]
            n1276 = property on="AO_SoundCard Channel" class="Ring (strict)"() -> ("Value"=w463:u16)  [unwired: 2 in, 2 out]
            n1277 = Equal To 0?(x=w463) -> (x = 0?=w466:bool)
            n1278 = Select(t=1 ("y"), s=w466, f=0 ("y")) -> (s? t:f=w462:i32)
            n1279 = Index Array(array=w468, index #1=w463, index #2=w462) -> (element #1=w467:string, element #2=w461:string)
          }
          frame 1, Default {
            n1280 = property on="AI_SoundCard Channel" class="Ring (strict)"() -> ("Value"=w474:u16)  [unwired: 2 in, 2 out]
            n1281 = property on="AI_SoundCard Channel" class="Ring (strict)"() -> ("Strings []"=w476:string[])  [unwired: 2 in, 2 out]
            n1282 = Equal To 0?(x=w474) -> (x = 0?=w473:bool)
            n1283 = Select(t=1 ("y"), s=w473, f=0 ("y")) -> (s? t:f=w470:i32)
            n1284 = Index Array(array=w476, index #1=w474, index #2=w470) -> (element #1=w475:string, element #2=w469:string)
          }
        }
        n1285 = case shown="1" w285 {
          tunnel: [w480 w484 w487] -> w291
          tunnel: w288 -> [w478 w483 _]
          tunnel: w286 -> [w479 _ w493]
          tunnel: [w477 w481 w492] -> w289
          tunnel: w284 -> [_ _ w492]
          frame 2, Default {
            # "Rename"
            n1286 = call "CRYGet Channel Name Dialog.vi"("Channel Name"=w479, "Window Title"=w478) -> ("Channel Name Out"=w477:string, "Return Flag"=w480:bool)  [unwired: 8 out]
          }
          frame 0 {
            # "Add"
            n1287 = call "CRYGet Channel Name Dialog.vi"("Channel Name"="", "Window Title"=w483) -> ("Channel Name Out"=w481:string, "Return Flag"=w484:bool)  [unwired: 8 out]
          }
          frame 1 {
            # "Delete"
            n1288 = call "CRYGet Error Message.vi"("Error No"=1 ("No"), "Kind"="SoundCard") -> ("Message"=w489:string, "Window Title"=w485:string)  [unwired: 4 in, 4 out]
            n1289 = Format Into String(format string=w489, w493) -> (resulting string=w488:string)  [unwired: 2 in, 1 out]
            n1290 = call "CRYMessage Dialog.vi"("Window Title"=w485, "YesNoCancel"=T8."YesNo", "Message Content"=w488) -> ("YesNo"=w487:bool)  [unwired: 7 in, 1 out]
          }
        }
        n1291 = case shown="True" w291 {
          tunnel: w289 -> [_ w296]
          tunnel: w283 -> [_ w297]
          tunnel: w286 -> [_ w295]
          frame False {
          }
          frame True {
            # "Out_Add, Delete, Rename\n   In_Add, Delete, Rename"
            n1292 = local read "O_Channel Info"() -> (w294:T2[])
            n1293 = local read "I_Channel Info"() -> (w293:T2[])
            n1294 = case shown="4" w297 {
              tunnel: w296 -> [w300 _ w359 w382 _ w440]
              tunnel: w294 -> [w298 w355 w357 _ _ _]
              tunnel: w293 -> [_ _ _ w380 w436 w438]
              tunnel: w295 -> [_ w348 w356 _ w429 w437]
              frame 0, Default {
                # "Output Add"
                n1295 = call "CRYTest Duplicate Channels.vi"("Channel Info"=w298, "Channel Name"=w300) -> ("Exist Flag"=w299:bool)  [unwired: 9 out]
                n1296 = case shown="True" w299 {
                  tunnel: w300 -> [_ w307]
                  tunnel: w298 -> [_ w306]
                  frame True {
                    n1297 = call "CRYGet Error Message.vi"("Error No"=2 ("No"), "Kind"="SoundCard") -> ("Message"=w305:string, "Window Title"=w301:string)  [unwired: 4 in, 4 out]
                    n1298 = call "CRYMessage Dialog.vi"("Window Title"=w301, "YesNoCancel"=T8."OK", "Message Content"=w305) -> ()  [unwired: 7 in, 2 out]
                  }
                  frame False {
                    n1299 = flat-sequence {
                      tunnel: w307 -> [w319]
                      tunnel: [w309] -> w308
                      tunnel: w306 -> [w320]
                      tunnel: w308 -> [w346]
                      frame #0 {
                        n1300 = local read "AO_Select Channel1"() -> (w341:u16)
                        n1301 = local read "AO_Sampling Rate"() -> (w330:u32)
                        n1302 = local read "AO_Sampling User"() -> (w337:u32)
                        n1303 = local read "AO_Select SMode"() -> (w334:enum32{"Analog", "Digital"})
                        n1304 = local read "AO_Device Name"() -> (w321:u16)
                        n1305 = property on="AO_SoundCard Channel" class="Ring (strict)"() -> ("Value"=w326:u16)  [unwired: 2 in, 2 out]
                        n1306 = local read "AO_Audio Driver"() -> (w314:enum32{"Radio Selection 1", "Radio Selection 2"})
                        n1307 = local read "AO_Bit Depth"() -> (w340:u16)
                        n1308 = local read "AO_Alias freq"() -> (w327:u32)
                        n1309 = property on="AO_Device Name" class="Ring (strict)"() -> ("RingText.Text"=w336:string)  [unwired: 2 in, 2 out]
                        n1310 = local read "AO_Vp"() -> (w339:dbl)
                        n1311 = Increment(x=w326) -> (x+1=w323:u16)
                        n1312 = Equal To 0?(x=w314) -> (x = 0?=w315:bool)
                        n1313 = Not Equal To 0?(x=w330) -> (x != 0?=w338:bool)
                        n1314 = Array Size(array=w320) -> (size(s)=w325:i32)
                        n1315 = Select(t=w330, s=w338, f=w337) -> (s? t:f=w329:u32)
                        n1316 = Equal?(x=w334, y=enum32{"Analog", "Digital"}."Digital" ("AO_Select Channel2")) -> (x = y?=w332:bool)
                        n1317 = Select(t=w314, s=w315, f=2) -> (s? t:f=w312:u32)
                        n1318 = Equal To 0?(x=w325) -> (x = 0?=w324:bool)
                        n1319 = Select(t=u16 0, s=w324, f=w323) -> ()  [unwired: 1 out]
                        n1320 = local read "Channel Info"() -> (w342:T2)
                        n1321 = Bundle By Name(cluster=w342, "ID"=w321, "Name"=w319, "Digital"=w332, "Input"=FALSE, "Device Name"=w336, "Hardware Ch ID"=w341, "Vmax (V)"=w339, "Latency (samples)"=0.0, "Sampling Rate (Hz)"=w329, "Bit Depth"=w340, "Anti-aliasing Factor (%fs)"=w327, "Audio Driver"=w312) -> (w343:T2)
                        n1322 = Insert Into Array(array=w320, new element=w343) -> (w328:T2[])  [unwired: 1 in]
                        n1323 = for {
                          tunnel: w328 -> [w345] mode=indexing
                          tunnel: [w344] -> w310 mode=indexing
                          n1324 = Unbundle By Name(w345) -> ("Name"=w344:string)
                        }
                        n1325 = local write "O_Channel Info"(w328) -> ()
                        n1326 = property on="O_Name" class="Arr (strict)"() -> ("Value"=w318:string[][])  [unwired: 2 in, 2 out]
                        n1327 = call "CRYSet Channel Changing State.vi"("Name In"=w318, "New Channel Name"=w319, "Mode"=enum16{"Add", "Delete", "Rename", "Load/Revert"}."Add") -> ("Name Out"=w317:string[][])  [unwired: 8 in]
                        n1328 = property on="AO_SoundCard Channel" class="Ring (strict)"("Strings []"=w310) -> ()  [unwired: 2 in, 2 out]
                        n1329 = Array Size(array=w310) -> (size(s)=w311:i32)
                        n1330 = property on="O_Name" class="Arr (strict)"("Value"=w317) -> ()  [unwired: 2 in, 2 out]
                        n1331 = Decrement(x=w311) -> (x-1=w309:i32)
                      }
                      frame #1 {
                        n1332 = property on="AO_SoundCard Channel" class="Ring (strict)"("Val(Sgnl)"=w346) -> ()  [unwired: 2 in, 2 out]
                      }
                    }
                  }
                }
              }
              frame 1 {
                # "Delete"
                n1333 = property on="AO_SoundCard Channel" class="Ring (strict)"() -> ("Value"=w351:u16)  [unwired: 2 in, 2 out]
                n1334 = property on="O_Name" class="Arr (strict)"() -> ("Value"=w350:string[][])  [unwired: 2 in, 2 out]
                n1335 = call "CRYDelete Channel Info.vi"("Channel Info In"=w355, "Selected Index"=w351) -> ("Channel Info Out"=w354:T2[], "Name Array"=w352:string[], "New Index"=w353:u16)  [unwired: 7 in]
                n1336 = call "CRYSet Channel Changing State.vi"("Name In"=w350, "Old Channel Name"=w348, "Mode"=enum16{"Add", "Delete", "Rename", "Load/Revert"}."Delete") -> ("Name Out"=w349:string[][])  [unwired: 8 in]
                n1337 = local write "O_Channel Info"(w354) -> ()
                n1338 = property on="AO_SoundCard Channel" class="Ring (strict)"("Strings []"=w352) -> ()  [unwired: 2 in, 2 out]
                n1339 = property on="AO_SoundCard Channel" class="Ring (strict)"("Val(Sgnl)"=w353) -> ()  [unwired: 2 in, 2 out]
                n1340 = property on="O_Name" class="Arr (strict)"("Value"=w349) -> ()  [unwired: 2 in, 2 out]
              }
              frame 2 {
                # "Rename"
                n1341 = call "CRYTest Duplicate Channels.vi"("Channel Info"=w357, "Channel Name"=w359) -> ("Exist Flag"=w358:bool)  [unwired: 9 out]
                n1342 = case shown="True" w358 {
                  tunnel: w357 -> [_ w367]
                  tunnel: w359 -> [_ w366]
                  tunnel: w356 -> [_ w365]
                  frame True {
                    n1343 = call "CRYGet Error Message.vi"("Error No"=2 ("No"), "Kind"="SoundCard") -> ("Message"=w360:string, "Window Title"=w364:string)  [unwired: 4 in, 4 out]
                    n1344 = call "CRYMessage Dialog.vi"("Window Title"=w364, "YesNoCancel"=T8."OK", "Message Content"=w360) -> ()  [unwired: 7 in, 2 out]
                  }
                  frame False {
                    n1345 = flat-sequence {
                      tunnel: [w374] -> w368
                      tunnel: w366 -> [w371]
                      tunnel: w367 -> [w377]
                      tunnel: w365 -> [w370]
                      tunnel: w368 -> [w379]
                      frame #0 {
                        n1346 = property on="AO_SoundCard Channel" class="Ring (strict)"() -> ("Value"=w378:u16)  [unwired: 2 in, 2 out]
                        n1347 = property on="O_Name" class="Arr (strict)"() -> ("Value"=w372:string[][])  [unwired: 2 in, 2 out]
                        n1348 = call "CRYRename Channel Info.vi"("Channel Info In"=w377, "Channel Name"=w371, "Selected Index"=w378) -> ("Channel Info Out"=w376:T2[], "Name Array"=w375:string[], "New Index"=w374:u16)  [unwired: 6 in]
                        n1349 = call "CRYSet Channel Changing State.vi"("Name In"=w372, "New Channel Name"=w371, "Old Channel Name"=w370, "Mode"=enum16{"Add", "Delete", "Rename", "Load/Revert"}."Rename") -> ("Name Out"=w373:string[][])  [unwired: 7 in]
                        n1350 = local write "O_Channel Info"(w376) -> ()
                        n1351 = property on="AO_SoundCard Channel" class="Ring (strict)"("Strings []"=w375) -> ()  [unwired: 2 in, 2 out]
                        n1352 = property on="O_Name" class="Arr (strict)"("Value"=w373) -> ()  [unwired: 2 in, 2 out]
                      }
                      frame #1 {
                        n1353 = property on="AO_SoundCard Channel" class="Ring (strict)"("Val(Sgnl)"=w379) -> ()  [unwired: 2 in, 2 out]
                      }
                    }
                  }
                }
              }
              frame 3 {
                # "Input Add"
                n1354 = call "CRYTest Duplicate Channels.vi"("Channel Info"=w380, "Channel Name"=w382) -> ("Exist Flag"=w381:bool)  [unwired: 9 out]
                n1355 = case shown="True" w381 {
                  tunnel: w380 -> [_ w389]
                  tunnel: w382 -> [_ w388]
                  frame True {
                    n1356 = call "CRYGet Error Message.vi"("Error No"=2 ("No"), "Kind"="SoundCard") -> ("Message"=w387:string, "Window Title"=w383:string)  [unwired: 4 in, 4 out]
                    n1357 = call "CRYMessage Dialog.vi"("Window Title"=w383, "YesNoCancel"=T8."OK", "Message Content"=w387) -> ()  [unwired: 7 in, 2 out]
                  }
                  frame False {
                    n1358 = flat-sequence {
                      tunnel: w388 -> [w399]
                      tunnel: [w391] -> w390
                      tunnel: w389 -> [w402]
                      tunnel: w390 -> [w427]
                      frame #0 {
                        n1359 = property on="AI_SoundCard Channel" class="Ring (strict)"() -> ("Value"=w405:u16)  [unwired: 2 in, 2 out]
                        n1360 = local read "AI_Device Name"() -> (w403:u16)
                        n1361 = local read "AI_Sampling Rate"() -> (w412:u32)
                        n1362 = local read "AI_Sampling User"() -> (w418:u32)
                        n1363 = local read "AI_Select Channel1"() -> (w422:u16)
                        n1364 = local read "AI_Bit Depth"() -> (w421:u16)
                        n1365 = property on="AI_Device Name" class="Ring (strict)"() -> ("RingText.Text"=w417:string)  [unwired: 2 in, 2 out]
                        n1366 = local read "AI_Latency"() -> (w411:u32)
                        n1367 = local read "AI_Vp"() -> (w420:dbl)
                        n1368 = local read "AI_Alias freq"() -> (w408:u32)
                        n1369 = local read "AI_Select SMode"() -> (w416:enum32{"Analog", "Digital"})
                        n1370 = local read "AI_Audio Driver"() -> (w396:enum32{"Radio Selection 1", "Radio Selection 2"})
                        n1371 = Increment(x=w405) -> ()  [unwired: 1 out]
                        n1372 = Array Size(array=w402) -> (size(s)=w407:i32)
                        n1373 = Equal To 0?(x=w396) -> (x = 0?=w397:bool)
                        n1374 = Not Equal To 0?(x=w412) -> (x != 0?=w419:bool)
                        n1375 = Select(t=w412, s=w419, f=w418) -> (s? t:f=w410:u32)
                        n1376 = Equal?(x=w416, y=enum32{"Analog", "Digital"}."Digital" ("AO_Select Channel2")) -> (x = y?=w414:bool)
                        n1377 = Equal To 0?(x=w407) -> (x = 0?=w404:bool)
                        n1378 = Select(t=w396, s=w397, f=2) -> (s? t:f=w394:u32)
                        n1379 = Select(t=u16 0, s=w404, f=w405) -> ()  [unwired: 1 out]
                        n1380 = local read "Channel Info"() -> (w423:T2)
                        n1381 = Bundle By Name(cluster=w423, "ID"=w403, "Name"=w399, "Digital"=w414, "Input"=TRUE, "Device Name"=w417, "Hardware Ch ID"=w422, "Vmax (V)"=w420, "Latency (samples)"=w411, "Sampling Rate (Hz)"=w410, "Bit Depth"=w421, "Anti-aliasing Factor (%fs)"=w408, "Audio Driver"=w394) -> (w424:T2)
                        n1382 = Insert Into Array(array=w402, new element=w424) -> (w409:T2[])  [unwired: 1 in]
                        n1383 = for {
                          tunnel: w409 -> [w426] mode=indexing
                          tunnel: [w425] -> w393 mode=indexing
                          n1384 = Unbundle By Name(w426) -> ("Name"=w425:string)
                        }
                        n1385 = local write "I_Channel Info"(w409) -> ()
                        n1386 = property on="I_Name" class="Arr (strict)"() -> ("Value"=w400:string[][])  [unwired: 2 in, 2 out]
                        n1387 = call "CRYSet Channel Changing State.vi"("Name In"=w400, "New Channel Name"=w399, "Mode"=enum16{"Add", "Delete", "Rename", "Load/Revert"}."Add") -> ("Name Out"=w401:string[][])  [unwired: 8 in]
                        n1388 = property on="I_Name" class="Arr (strict)"("Value"=w401) -> ()  [unwired: 2 in, 2 out]
                        n1389 = property on="AI_SoundCard Channel" class="Ring (strict)"("Strings []"=w393) -> ()  [unwired: 2 in, 2 out]
                        n1390 = Array Size(array=w393) -> (size(s)=w392:i32)
                        n1391 = Decrement(x=w392) -> (x-1=w391:i32)
                      }
                      frame #1 {
                        n1392 = property on="AI_SoundCard Channel" class="Ring (strict)"("Val(Sgnl)"=w427) -> ()  [unwired: 2 in, 2 out]
                      }
                    }
                  }
                }
              }
              frame 4 {
                # "Delete"
                n1393 = property on="AI_SoundCard Channel" class="Ring (strict)"() -> ("Value"=w434:u16)  [unwired: 2 in, 2 out]
                n1394 = property on="I_Name" class="Arr (strict)"() -> ("Value"=w431:string[][])  [unwired: 2 in, 2 out]
                n1395 = call "CRYSet Channel Changing State.vi"("Name In"=w431, "Old Channel Name"=w429, "Mode"=enum16{"Add", "Delete", "Rename", "Load/Revert"}."Delete") -> ("Name Out"=w430:string[][])  [unwired: 8 in]
                n1396 = call "CRYDelete Channel Info.vi"("Channel Info In"=w436, "Selected Index"=w434) -> ("Channel Info Out"=w435:T2[], "Name Array"=w432:string[], "New Index"=w433:u16)  [unwired: 7 in]
                n1397 = property on="I_Name" class="Arr (strict)"("Value"=w430) -> ()  [unwired: 2 in, 2 out]
                n1398 = property on="AI_SoundCard Channel" class="Ring (strict)"("Val(Sgnl)"=w433) -> ()  [unwired: 2 in, 2 out]
                n1399 = property on="AI_SoundCard Channel" class="Ring (strict)"("Strings []"=w432) -> ()  [unwired: 2 in, 2 out]
                n1400 = local write "I_Channel Info"(w435) -> ()
              }
              frame 5 {
                # "Rename"
                n1401 = call "CRYTest Duplicate Channels.vi"("Channel Info"=w438, "Channel Name"=w440) -> ("Exist Flag"=w439:bool)  [unwired: 9 out]
                n1402 = case shown="True" w439 {
                  tunnel: w440 -> [_ w448]
                  tunnel: w438 -> [_ w447]
                  tunnel: w437 -> [_ w446]
                  frame True {
                    n1403 = call "CRYGet Error Message.vi"("Error No"=2 ("No"), "Kind"="SoundCard") -> ("Message"=w441:string, "Window Title"=w445:string)  [unwired: 4 in, 4 out]
                    n1404 = call "CRYMessage Dialog.vi"("Window Title"=w445, "YesNoCancel"=T8."OK", "Message Content"=w441) -> ()  [unwired: 7 in, 2 out]
                  }
                  frame False {
                    n1405 = flat-sequence {
                      tunnel: [w455] -> w449
                      tunnel: w448 -> [w452]
                      tunnel: w447 -> [w459]
                      tunnel: w446 -> [w451]
                      tunnel: w449 -> [w460]
                      frame #0 {
                        n1406 = property on="AI_SoundCard Channel" class="Ring (strict)"() -> ("Value"=w458:u16)  [unwired: 2 in, 2 out]
                        n1407 = call "CRYRename Channel Info.vi"("Channel Info In"=w459, "Channel Name"=w452, "Selected Index"=w458) -> ("Channel Info Out"=w457:T2[], "Name Array"=w456:string[], "New Index"=w455:u16)  [unwired: 6 in]
                        n1408 = property on="I_Name" class="Arr (strict)"() -> ("Value"=w453:string[][])  [unwired: 2 in, 2 out]
                        n1409 = local write "I_Channel Info"(w457) -> ()
                        n1410 = property on="AI_SoundCard Channel" class="Ring (strict)"("Strings []"=w456) -> ()  [unwired: 2 in, 2 out]
                        n1411 = call "CRYSet Channel Changing State.vi"("Name In"=w453, "New Channel Name"=w452, "Old Channel Name"=w451, "Mode"=enum16{"Add", "Delete", "Rename", "Load/Revert"}."Rename") -> ("Name Out"=w454:string[][])  [unwired: 7 in]
                        n1412 = property on="I_Name" class="Arr (strict)"("Value"=w454) -> ()  [unwired: 2 in, 2 out]
                      }
                      frame #1 {
                        n1413 = property on="AI_SoundCard Channel" class="Ring (strict)"("Val(Sgnl)"=w460) -> ()  [unwired: 2 in, 2 out]
                      }
                    }
                  }
                }
              }
            }
          }
        }
      }
      frame 7 {
        # "Open Table"
        n1414 = local read "O_Channel Info"() -> (w499:T2[])
        n1415 = local read "I_Channel Info"() -> (w498:T2[])
        n1416 = local read "O_Device Info"() -> (w503:T3)
        n1417 = local read "I_Device Info"() -> (w502:T3)
        n1418 = property on="O_Name" class="Arr (strict)"() -> ("Value"=w494:string[][])  [unwired: 2 in, 2 out]
        n1419 = property on="I_Name" class="Arr (strict)"() -> ("Value"=w495:string[][])  [unwired: 2 in, 2 out]
        n1420 = call "CRYChannel Table.vi"("I_Device Info"=w502, "I_Channel Info"=w498, "I_Name In"=w495, "O_Name In"=w494, "O_Device Info"=w503, "O_Channel Info"=w499) -> ("O_Channel Info Out"=w501:T2[], "I_Channel Info Out"=w500:T2[], "I_Name Out"=w497:string[][], "O_Name Out"=w496:string[][], "Return Flag"=w504:bool)  [unwired: 5 in]
        n1421 = case shown="True" w504 {
          tunnel: w501 -> [_ w507]
          tunnel: w500 -> [_ w508]
          tunnel: w497 -> [_ w506]
          tunnel: w496 -> [_ w505]
          frame False {
          }
          frame True {
            n1422 = flat-sequence {
              tunnel: w508 -> [w517]
              tunnel: w507 -> [w516]
              tunnel: w506 -> [w511]
              tunnel: w505 -> [w510]
              frame #0 {
                w513 = u16 0 ("SelectedOut")
                n1423 = property on="O_Name" class="Arr (strict)"("Value"=w510) -> ()  [unwired: 2 in, 2 out]
                n1424 = property on="I_Name" class="Arr (strict)"("Value"=w511) -> ()  [unwired: 2 in, 2 out]
                n1425 = local write "O_Channel Info"(w516) -> ()
                n1426 = local write "I_Channel Info"(w517) -> ()
                n1427 = local read "SoundCard"() -> (w514:T5)
                n1428 = Insert Into Array(array=w516, new element=w517) -> (w515:T2[])  [unwired: 1 in]
                n1429 = Bundle By Name(cluster=w514, "Channel Array"=w515, "SelectedOut"=w513, "SelectedIn"=w513) -> (w512:T5)
                n1430 = local write "SoundCard"(w512) -> ()
                n1431 = local write "Mode"("OpenTable" ("Mode")) -> ()
              }
              frame #1 {
                n1432 = local write "Load Test"(TRUE ("Load Test")) -> ()
              }
            }
          }
        }
      }
      frame 8 {
        # "Calibrate"
        n1433 = flat-sequence {
          tunnel: [w524] -> w521
          tunnel: [w523] -> w520
          tunnel: [w522] -> w519
          tunnel: w521 -> [w541]
          tunnel: w520 -> [w540]
          tunnel: w519 -> [w539]
          frame #0 {
            w527 = 1.0 ("Sens Out")
            w528 = u16 0 ("Signal Type Out")
            n1434 = local read "O_Channel Info"() -> (w534:T2[])
            n1435 = property on="AO_SoundCard Channel" class="Ring (strict)"() -> ("Value"=w532:u16)  [unwired: 2 in, 2 out]
            n1436 = property on="Calibration Seq" class="Ring (strict)"() -> ("RingText.Text"=w524:string)  [unwired: 2 in, 2 out]
            n1437 = local read "I_Channel Info"() -> (w533:T2[])
            n1438 = property on="AI_SoundCard Channel" class="Ring (strict)"() -> ("Value"=w531:u16)  [unwired: 2 in, 2 out]
            n1439 = Equal?(x=w524, y="CRY6181 Calibration") -> (x = y?=w523:bool)
            n1440 = case shown="True" w523 {
              selector: w523 -> [_ w538]
              tunnel: [FALSE ("Error") w537] -> w522
              frame False {
              }
              frame True {
                n1441 = global write "CRYCal Global.vi" "SoundCard CRY6181"(w538) -> ()
                n1442 = call "CRYMake CRY6181 Calibration Data.vi"() -> ("Error"=w537:bool)  [unwired: 11 in]
              }
            }
            n1443 = Index Array(array=w533, index=w531) -> (element=w530:T2)
            n1444 = Index Array(array=w534, index=w532) -> (element=w529:T2)
            n1445 = global write "CRYCal Global.vi" "Output Hardware Cal"(w529) -> ()
            n1446 = global write "CRYCal Global.vi" "Input Hardware Cal"(w530) -> ()
            n1447 = global write "CRYCal Global.vi" "SoundCard Calibrate"(TRUE ("Audio Interface Calibrate")) -> ()
            n1448 = global write "CRYCal Global.vi" "Signal Type Out"(w528) -> ()
            n1449 = global write "CRYCal Global.vi" "Signal Type In"(w528) -> ()
            n1450 = global write "CRYCal Global.vi" "Calibrate"(TRUE ("Calibrate")) -> ()
            n1451 = global write "CRYCal Global.vi" "Sens Out"(w527) -> ()
            n1452 = global write "CRYCal Global.vi" "Sens In"(w527) -> ()
            n1453 = call "CRYBackup Work State.vi"() -> ()  [unwired: 12 in]
          }
          frame #1 {
            n1454 = case shown="False" w539 {
              tunnel: [w544 FALSE ("run state")] -> w542
              tunnel: w541 -> [w543 _]
              frame False {
                n1455 = call "CRYRun Selected Project.vi"("sequence name"=w543) -> ("run state"=w544:bool)  [unwired: 10 out]
              }
              frame True {
              }
            }
            n1456 = case shown="True" w542 {
              tunnel: w540 -> [_ w546]
              frame False {
              }
              frame True {
                n1457 = case shown="True" w546 {
                  frame False {
                    n1458 = call "CRYGet Curve Library Array.vi"("Type In"=enum16{"Curves", "Values", "Results", "WFM"}."Values") -> ("Curve/Value array"=w547:T16)  [unwired: 8 in, 2 out]
                    n1459 = call "CRYSelect curve by name.vi"("Curve name desired (just name, if flat data not wired)"="Record Delay", "Data array"=w547) -> ("Exists?"=w549:bool, "Desired Curve"=w550:T17)  [unwired: 1 in, 7 out]
                    n1460 = call "CRYSelect curve by name.vi"("Curve name desired (just name, if flat data not wired)"="Max In", "Data array"=w547) -> ("Exists?"=w552:bool, "Desired Curve"=w553:T17)  [unwired: 1 in, 7 out]
                    n1461 = call "CRYSelect curve by name.vi"("Curve name desired (just name, if flat data not wired)"="Max Out", "Data array"=w547) -> ("Exists?"=w554:bool, "Desired Curve"=w555:T17)  [unwired: 1 in, 7 out]
                    n1462 = case shown="True" w554 {
                      tunnel: w555 -> [_ w569]
                      frame False {
                      }
                      frame True {
                        n1463 = Unbundle By Name(w569) -> ("Curve"=w568:cluster{"x":dbl, "y":dbl, "z":dbl}[])
                        n1464 = Index Array(array=w568) -> (element=w567:cluster{"x":dbl, "y":dbl, "z":dbl})  [unwired: 1 in]
                        n1465 = Unbundle By Name(w567) -> ("y"=w566:dbl)
                        n1466 = property on="AO_Vp" class="DigNum (strict)"("Val(Sgnl)"=w566) -> ()  [unwired: 2 in, 2 out]
                      }
                    }
                    n1467 = case shown="True" w552 {
                      tunnel: w553 -> [_ w565]
                      frame False {
                      }
                      frame True {
                        n1468 = Unbundle By Name(w565) -> ("Curve"=w564:cluster{"x":dbl, "y":dbl, "z":dbl}[])
                        n1469 = Index Array(array=w564) -> (element=w563:cluster{"x":dbl, "y":dbl, "z":dbl})  [unwired: 1 in]
                        n1470 = Unbundle By Name(w563) -> ("y"=w562:dbl)
                        n1471 = property on="AI_Vp" class="DigNum (strict)"("Val(Sgnl)"=w562) -> ()  [unwired: 2 in, 2 out]
                      }
                    }
                    n1472 = case shown="True" w549 {
                      tunnel: w550 -> [_ w559]
                      frame False {
                      }
                      frame True {
                        n1473 = Unbundle By Name(w559) -> ("Curve"=w560:cluster{"x":dbl, "y":dbl, "z":dbl}[])
                        n1474 = Index Array(array=w560) -> (element=w561:cluster{"x":dbl, "y":dbl, "z":dbl})  [unwired: 1 in]
                        n1475 = Unbundle By Name(w561) -> ("z"=w558:dbl)
                        n1476 = property on="AI_Latency" class="DigNum (strict)"("Val(Sgnl)"=w558) -> ()  [unwired: 2 in, 2 out]
                      }
                    }
                  }
                  frame True {
                    w578 = 3.5 ("x")
                    n1477 = call "CRYGet Curve Library Array.vi"("Type In"=enum16{"Curves", "Values", "Results", "WFM"}."Curves") -> ("Curve/Value array"=w605:T16)  [unwired: 8 in, 2 out]
                    n1478 = call "CRYSelect curve by name.vi"("Curve name desired (just name, if flat data not wired)"="Input Voltage2", "Data array"=w605) -> ("Exists?"=w595:bool, "Desired Curve"=w599:T17)  [unwired: 1 in, 7 out]
                    n1479 = call "CRYSelect curve by name.vi"("Curve name desired (just name, if flat data not wired)"="Input Voltage4", "Data array"=w605) -> ("Exists?"=w593:bool, "Desired Curve"=w597:T17)  [unwired: 1 in, 7 out]
                    n1480 = call "CRYSelect curve by name.vi"("Curve name desired (just name, if flat data not wired)"="Input Voltage1", "Data array"=w605) -> ("Exists?"=w596:bool, "Desired Curve"=w600:T17)  [unwired: 1 in, 7 out]
                    n1481 = call "CRYSelect curve by name.vi"("Curve name desired (just name, if flat data not wired)"="Input Voltage3", "Data array"=w605) -> ("Exists?"=w594:bool, "Desired Curve"=w598:T17)  [unwired: 1 in, 7 out]
                    n1482 = call "CRYSelect curve by name.vi"("Curve name desired (just name, if flat data not wired)"="Output Voltage2", "Data array"=w605) -> ("Exists?"=w591:bool, "Desired Curve"=w592:T17)  [unwired: 1 in, 7 out]
                    n1483 = call "CRYSelect curve by name.vi"("Curve name desired (just name, if flat data not wired)"="Output Voltage1", "Data array"=w605) -> ("Exists?"=w615:bool, "Desired Curve"=w616:T17)  [unwired: 1 in, 7 out]
                    n1484 = case shown="True" w615 {
                      tunnel: w616 -> [_ w745]
                      tunnel: [0.0 ("y") w737] -> w575
                      frame False {
                      }
                      frame True {
                        n1485 = Unbundle By Name(w745) -> ("Curve"=w743:cluster{"x":dbl, "y":dbl, "z":dbl}[])
                        n1486 = for {
                          tunnel: w743 -> [w748] mode=indexing
                          tunnel: [w747] -> w742 mode=indexing
                          tunnel: [w746] -> w740 mode=indexing
                          n1487 = Unbundle By Name(w748) -> ("x"=w747:dbl, "y"=w746:dbl)
                        }
                        n1488 = Search 1D Array(1D array=w742, element=1000.0) -> (index of element=w741:i32)  [unwired: 1 in]
                        n1489 = Index Array(array=w740, index=w741) -> (element=w738:dbl)
                        n1490 = Multiply(x=35.0, y=w738) -> (x*y=w737:dbl)
                      }
                    }
                    n1491 = case shown="True" w591 {
                      tunnel: w592 -> [_ w698]
                      tunnel: [0.0 ("y") w690] -> w572
                      frame False {
                      }
                      frame True {
                        n1492 = Unbundle By Name(w698) -> ("Curve"=w696:cluster{"x":dbl, "y":dbl, "z":dbl}[])
                        n1493 = for {
                          tunnel: w696 -> [w701] mode=indexing
                          tunnel: [w700] -> w695 mode=indexing
                          tunnel: [w699] -> w693 mode=indexing
                          n1494 = Unbundle By Name(w701) -> ("x"=w700:dbl, "y"=w699:dbl)
                        }
                        n1495 = Search 1D Array(1D array=w695, element=1000.0) -> (index of element=w694:i32)  [unwired: 1 in]
                        n1496 = Index Array(array=w693, index=w694) -> (element=w691:dbl)
                        n1497 = Multiply(x=35.0, y=w691) -> (x*y=w690:dbl)
                      }
                    }
                    n1498 = case shown="True" w596 {
                      tunnel: w600 -> [_ w725]
                      tunnel: [0.0 ("y") w721] -> w574
                      frame False {
                      }
                      frame True {
                        n1499 = Unbundle By Name(w725) -> ("Curve"=w724:cluster{"x":dbl, "y":dbl, "z":dbl}[])
                        n1500 = Index Array(array=w724) -> (element=w723:cluster{"x":dbl, "y":dbl, "z":dbl})  [unwired: 1 in]
                        n1501 = Unbundle By Name(w723) -> ("y"=w722:dbl)
                        n1502 = Reciprocal(x=w722) -> (1/x=w721:dbl)
                      }
                    }
                    n1503 = case shown="True" w595 {
                      tunnel: w599 -> [_ w719]
                      tunnel: [0.0 ("y") w715] -> w570
                      frame False {
                      }
                      frame True {
                        n1504 = Unbundle By Name(w719) -> ("Curve"=w718:cluster{"x":dbl, "y":dbl, "z":dbl}[])
                        n1505 = Index Array(array=w718) -> (element=w717:cluster{"x":dbl, "y":dbl, "z":dbl})  [unwired: 1 in]
                        n1506 = Unbundle By Name(w717) -> ("y"=w716:dbl)
                        n1507 = Reciprocal(x=w716) -> (1/x=w715:dbl)
                      }
                    }
                    n1508 = case shown="True" w594 {
                      tunnel: w598 -> [_ w713]
                      tunnel: [0.0 ("y") w709] -> w580
                      frame False {
                      }
                      frame True {
                        n1509 = Unbundle By Name(w713) -> ("Curve"=w712:cluster{"x":dbl, "y":dbl, "z":dbl}[])
                        n1510 = Index Array(array=w712) -> (element=w711:cluster{"x":dbl, "y":dbl, "z":dbl})  [unwired: 1 in]
                        n1511 = Unbundle By Name(w711) -> ("y"=w710:dbl)
                        n1512 = Reciprocal(x=w710) -> (1/x=w709:dbl)
                      }
                    }
                    n1513 = case shown="True" w593 {
                      tunnel: w597 -> [_ w707]
                      tunnel: [0.0 ("y") w703] -> w579
                      frame False {
                      }
                      frame True {
                        n1514 = Unbundle By Name(w707) -> ("Curve"=w706:cluster{"x":dbl, "y":dbl, "z":dbl}[])
                        n1515 = Index Array(array=w706) -> (element=w705:cluster{"x":dbl, "y":dbl, "z":dbl})  [unwired: 1 in]
                        n1516 = Unbundle By Name(w705) -> ("y"=w704:dbl)
                        n1517 = Reciprocal(x=w704) -> (1/x=w703:dbl)
                      }
                    }
                    n1518 = Multiply(x=w578, y=w574) -> (x*y=w582:dbl)
                    n1519 = Multiply(x=w578, y=w570) -> (x*y=w581:dbl)
                    n1520 = Multiply(x=w578, y=w580) -> (x*y=w576:dbl)
                    n1521 = Multiply(x=w578, y=w579) -> (x*y=w577:dbl)
                    n1522 = Multiply(x=w575, y=w574) -> (x*y=w573:dbl)
                    n1523 = Multiply(x=w572, y=w570) -> (x*y=w571:dbl)
                    n1524 = call "CRYGet Curve Library Array.vi"("Type In"=enum16{"Curves", "Values", "Results", "WFM"}."Values") -> ("Curve/Value array"=w609:T16)  [unwired: 8 in, 2 out]
                    n1525 = call "CRYSelect curve by name.vi"("Curve name desired (just name, if flat data not wired)"="Record Delay1", "Data array"=w609) -> ("Exists?"=w612:bool, "Desired Curve"=w613:T17)  [unwired: 1 in, 7 out]
                    n1526 = call "CRYSelect curve by name.vi"("Curve name desired (just name, if flat data not wired)"="Record Delay2", "Data array"=w609) -> ("Exists?"=w606:bool, "Desired Curve"=w607:T17)  [unwired: 1 in, 7 out]
                    n1527 = local read "SoundCard"() -> (w590:T5)
                    n1528 = case shown="True" w612 {
                      tunnel: w613 -> [_ w733]
                      tunnel: [0.0 ("z") w732] -> w584
                      frame False {
                      }
                      frame True {
                        n1529 = Unbundle By Name(w733) -> ("Curve"=w734:cluster{"x":dbl, "y":dbl, "z":dbl}[])
                        n1530 = Index Array(array=w734) -> (element=w735:cluster{"x":dbl, "y":dbl, "z":dbl})  [unwired: 1 in]
                        n1531 = Unbundle By Name(w735) -> ("z"=w732:dbl)
                      }
                    }
                    n1532 = case shown="True" w606 {
                      tunnel: w607 -> [_ w728]
                      tunnel: [0.0 ("z") w727] -> w583
                      frame False {
                      }
                      frame True {
                        n1533 = Unbundle By Name(w728) -> ("Curve"=w729:cluster{"x":dbl, "y":dbl, "z":dbl}[])
                        n1534 = Index Array(array=w729) -> (element=w730:cluster{"x":dbl, "y":dbl, "z":dbl})  [unwired: 1 in]
                        n1535 = Unbundle By Name(w730) -> ("z"=w727:dbl)
                      }
                    }
                    n1536 = Unbundle By Name(w590) -> ("Channel Array"=w587:T2[])
                    n1537 = for {
                      tunnel: w587 -> [w688] mode=indexing
                      tunnel: [w687] -> w588 mode=indexing
                      n1538 = Unbundle By Name(w688) -> ("Name"=w687:string)
                    }
                    n1539 = for {
                      tunnel: string[] ["Input 1", "Input 2", "Input 3", "Input 4", "Output 1", "Output 2", "Output 3", "Output 4"] -> [w621] mode=indexing
                      tunnel: w588 -> [w632]
                      shift-right: [w628] -> w586
                      shift-left: w587 -> [w629]
                      tunnel: w582 -> [w627]
                      tunnel: w584 -> [w626]
                      tunnel: w583 -> [w625]
                      tunnel: w581 -> [w624]
                      tunnel: w576 -> [w623]
                      tunnel: w577 -> [w622]
                      tunnel: w573 -> [w620]
                      tunnel: w571 -> [w619]
                      i -> [w631]
                      n1540 = Search 1D Array(1D array=w632, element=w621) -> (index of element=w630:i32)  [unwired: 1 in]
                      n1541 = case shown="1, Default" w630 {
                        selector: w630 -> [_ w637]
                        tunnel: w631 -> [_ w645]
                        tunnel: w629 -> [w633 w644]
                        tunnel: [w633 w643] -> w628
                        tunnel: w627 -> [_ w634]
                        tunnel: w626 -> [_ w641]
                        tunnel: w625 -> [_ w640]
                        tunnel: w624 -> [_ w642]
                        tunnel: w623 -> [_ w639]
                        tunnel: w622 -> [_ w638]
                        tunnel: w620 -> [_ w636]
                        tunnel: w619 -> [_ w635]
                        frame -1 {
                        }
                        frame 1, Default {
                          n1542 = case shown="5, 7" w645 {
                            tunnel: w644 -> [w646 w651 w658 w665 w672 w678 w684]
                            tunnel: [w646 w653 w660 w667 w674 w680 w686] -> w643
                            tunnel: w642 -> [_ _ w656 _ _ _ _]
                            tunnel: w641 -> [_ w649 _ w662 _ _ _]
                            tunnel: w640 -> [_ _ w655 _ w669 _ _]
                            tunnel: w639 -> [_ _ _ w663 _ _ _]
                            tunnel: w638 -> [_ _ _ _ w670 _ _]
                            tunnel: w637 -> [_ w648 w654 w661 w668 w676 w682]
                            tunnel: w636 -> [_ _ _ _ _ w675 _]
                            tunnel: w635 -> [_ _ _ _ _ _ w681]
                            tunnel: w634 -> [_ w647 _ _ _ _ _]
                            frame Default {
                            }
                            frame 0 {
                              n1543 = Index Array(array=w651, index=w648) -> (element=w652:T2)
                              n1544 = Bundle By Name(cluster=w652, "Latency (samples)"=w649, "Vmax (V)"=w647) -> (w650:T2)
                              n1545 = Replace Array Subset(array=w651, new element=w650, index=w648) -> (w653:T2[])
                            }
                            frame 1 {
                              n1546 = Index Array(array=w658, index=w654) -> (element=w659:T2)
                              n1547 = Bundle By Name(cluster=w659, "Latency (samples)"=w655, "Vmax (V)"=w656) -> (w657:T2)
                              n1548 = Replace Array Subset(array=w658, new element=w657, index=w654) -> (w660:T2[])
                            }
                            frame 2 {
                              n1549 = Index Array(array=w665, index=w661) -> (element=w666:T2)
                              n1550 = Bundle By Name(cluster=w666, "Latency (samples)"=w662, "Vmax (V)"=w663) -> (w664:T2)
                              n1551 = Replace Array Subset(array=w665, new element=w664, index=w661) -> (w667:T2[])
                            }
                            frame 3 {
                              n1552 = Index Array(array=w672, index=w668) -> (element=w673:T2)
                              n1553 = Bundle By Name(cluster=w673, "Latency (samples)"=w669, "Vmax (V)"=w670) -> (w671:T2)
                              n1554 = Replace Array Subset(array=w672, new element=w671, index=w668) -> (w674:T2[])
                            }
                            frame 4, 6 {
                              n1555 = Index Array(array=w678, index=w676) -> (element=w679:T2)
                              n1556 = Bundle By Name(cluster=w679, "Vmax (V)"=w675) -> (w677:T2)
                              n1557 = Replace Array Subset(array=w678, new element=w677, index=w676) -> (w680:T2[])
                            }
                            frame 5, 7 {
                              n1558 = Index Array(array=w684, index=w682) -> (element=w685:T2)
                              n1559 = Bundle By Name(cluster=w685, "Vmax (V)"=w681) -> (w683:T2)
                              n1560 = Replace Array Subset(array=w684, new element=w683, index=w682) -> (w686:T2[])
                            }
                          }
                        }
                      }
                    }
                    n1561 = Bundle By Name(cluster=w590, "Channel Array"=w586) -> (w585:T5)
                    n1562 = local write "SoundCard"(w585) -> ()
                  }
                }
              }
            }
          }
          frame #2 {
            n1563 = call "CRYRestore Work State.vi"() -> ()  [unwired: 12 in]
            n1564 = call "CRYBackup All.vi"("sOption"="Restore") -> ()  [unwired: 11 in]
          }
          frame #3 {
            n1565 = local write "Calibrartion"(FALSE ("Calibrartion")) -> ()
            n1566 = local write "Load Test"(TRUE ("Load Test")) -> ()
            n1567 = global write "CRYCal Global.vi" "Calibrate"(FALSE ("Calibrate")) -> ()
            n1568 = global write "CRYCal Global.vi" "SoundCard CRY6181"(FALSE ("Audio Interface Calibrate")) -> ()
            n1569 = global write "CRYCal Global.vi" "SoundCard Calibrate"(FALSE ("Audio Interface Calibrate")) -> ()
          }
        }
      }
      frame 9 {
        n1570 = local write "stop"(TRUE ("stop")) -> ()
        n1571 = flat-sequence {
          frame #0 {
            n1572 = global read "CRYMainGlobal.vi" "Access Level"() -> (w757:enum16{"Engineer", "Technician", "Operator"})
            n1573 = case shown="\"Operator\", Default" w757 {
              tunnel: [_ ""] -> w756
              frame "Operator", Default {
                n1574 = call "CRYGet Error Message.vi"("Kind"="Step Setup") -> ("Window Title"=w760:string)  [unwired: 5 in, 5 out]
                n1575 = call "CRYGet Access Level Message.vi"("sAction"="OK") -> ("Multibyte string"=w762:string)  [unwired: 10 in]
                n1576 = call "CRYMessage Dialog.vi"("Window Title"=w760, "YesNoCancel"=T8."OK", "Message Content"=w762) -> ()  [unwired: 7 in, 2 out]
              }
              frame "Engineer" {
                n1577 = flat-sequence {
                  tunnel: [w766] -> w764
                  tunnel: w764 -> [w781]
                  frame #0 {
                    n1578 = local read "O_Channel Info"() -> (w771:T2[])
                    n1579 = local read "I_Channel Info"() -> (w770:T2[])
                    n1580 = local read "SoundCard"() -> (w772:T5)
                    n1581 = Build Array (concatenate)(w771, w770) -> (w769:T2[])
                    n1582 = global read "CRYProject Editor Global.vi" "SoundCard Step"() -> (w768:T6)
                    n1583 = Bundle By Name(cluster=w772, "Channel Array"=w769) -> (w766:T5)
                    n1584 = call "CRYFlatten SoundCard.vi"("SoundCard"=w766) -> ("SoundCard flattened"=w767:string)  [unwired: 10 in]
                    n1585 = Bundle By Name(cluster=w768, "Seq setup flattened"=w767) -> (w765:T6)
                    n1586 = local write "SoundCard"(w766) -> ()
                    n1587 = local read "Proper VI No"() -> (w775:i32)
                    n1588 = property on="I_Name" class="Arr (strict)"() -> ("Value"=w774:string[][])  [unwired: 2 in, 2 out]
                    n1589 = property on="O_Name" class="Arr (strict)"() -> ("Value"=w773:string[][])  [unwired: 2 in, 2 out]
                    n1590 = global write "CRYProject Editor Global.vi" "SoundCard Step"(w765) -> ()
                    n1591 = call "CRYSoundCard.vi"("O_Name In"=w773, "I_Name In"=w774, "SoundCard In"=w766, "Proper VI No In"=w775) -> ("O_Name Out"=w776:string[][], "I_Name Out"=w777:string[][])  [unwired: 6 in]
                    n1592 = property on="I_Name" class="Arr (strict)"("Value"=w777) -> ()  [unwired: 2 in, 2 out]
                    n1593 = property on="O_Name" class="Arr (strict)"("Value"=w776) -> ()  [unwired: 2 in, 2 out]
                  }
                  frame #1 {
                    w782 = "SoundCard" ("Step File Name")
                    n1594 = global read "CRYMainGlobal.vi" "SoundCard Step FileName"() -> (w778:string)
                    n1595 = global read "CRYMainGlobal.vi" "Steps path"() -> (w779:path)
                    n1596 = Build Path(base path=w779, name or relative path=w778) -> (appended path=w780:path)
                    n1597 = call "CRYFlatten SoundCard.vi"("SoundCard"=w781) -> ("SoundCard flattened"=w784:string)  [unwired: 10 out]
                    n1598 = call "CRYStep Write.vi"("Category Name"=w782, "All/Name/Write(0,1,2)?"=u8 2, "Step File Path"=w780, "Step flattened"=w784, "Step File Name"=w782) -> ()  [unwired: 4 in, 3 out]
                  }
                }
              }
            }
            n1599 = flat-sequence {
              tunnel: w756 -> [_]
              frame #0 {
                n1600 = call "CRYClose All Operator.vi"() -> ()  [unwired: 12 in]
              }
              frame #1 {
                n1601 = call "CRYASIOExit.vi"() -> ()  [unwired: 10 in, 2 out]
              }
            }
          }
          frame #1 {
            n1602 = local write "SaveSoundCard"(FALSE ("OK")) -> ()
          }
        }
        n1603 = disable-structure shown="Disabled" {
          frame Disabled {
            n1604 = local read "SoundCard"() -> (w794:T5)
            n1605 = local read "I_Channel Info"() -> (w792:T2[])
            n1606 = local read "O_Channel Info"() -> (w788:T2[])
            n1607 = Unbundle By Name(w794) -> ("In Audio Driver"=w793:u16, "SelectedIn"=w791:u16, "Out Audio Driver"=w789:u16, "SelectedOut"=w786:u16)
            n1608 = Index Array(array=w788, index=w786) -> (element=w787:T2)
            n1609 = Index Array(array=w792, index=w791) -> (element=w790:T2)
            n1610 = case shown="1" w793 {
              tunnel: w790 -> [_ w800]
              frame 0, Default {
              }
              frame 1 {
                n1611 = Unbundle By Name(w800) -> ("Device Name"=w799:string)
                n1612 = call "CRYASIOInitialize.vi"("Sampling Rate"=u32 0, "Driver Name"=w799) -> ()  [unwired: 8 in, 2 out]
              }
            }
            n1613 = case shown="1" w789 {
              tunnel: w787 -> [_ w797]
              frame 0, Default {
              }
              frame 1 {
                n1614 = Unbundle By Name(w797) -> ("Device Name"=w796:string)
                n1615 = call "CRYASIOInitialize.vi"("Sampling Rate"=u32 0, "Driver Name"=w796) -> ()  [unwired: 8 in, 2 out]
              }
            }
          }
          frame Enabled {
          }
        }
      }
      frame 10 {
        n1616 = local write "stop"(TRUE ("stop")) -> ()
        n1617 = local write "Cancel"(FALSE ("Cancel")) -> ()
      }
      frame 11 {
        n1618 = local write "SaveSoundCard"(FALSE ("OK")) -> ()
        n1619 = local write "Cancel"(FALSE ("Cancel")) -> ()
        n1620 = local write "stop"(TRUE ("stop")) -> ()
      }
      frame Default {
      }
    }
  }
  n1621 = flat-sequence {
    tunnel: w1 -> [_]
    frame #0 {
      n1622 = control-ref of="This VI"() -> (w1796:refnum<vi>)
      n1623 = call "CRYWork Before Step Close.vi"("StepVI Ref"=w1796) -> ()  [unwired: 11 in]
    }
    frame #1 {
      "EndFlag" <- TRUE ("EndFlag")
    }
  }
